vi "单体采集信息-new.vi"(0 "can卡类型":u8, 1 "设备索引号":u8, 2 "CAN端口":u8, 3 "VIC_Receive":refnum<vi>, 4 "数据":refnum<vi>, 5 "数据位置":refnum<vi>) -> ()   [LabVIEW 2013]
panel:
  out "Life:":dbl=25.0
  in  "213":bool
  in  "一次置位":bool
  in  "刷新":bool
  out "VCI_Receive 2":T1
  in  "板号":u8
  out "电池信息":T2
  in  "电池信息读取":bool
  out "时间":string
  in  "充电均衡":u32(colorbox)=6618880
  in  "放电均衡":u32(colorbox)=16711680
  out "均衡信息":string[][](table)=[["第1串", "1", "单体检测其它故障", "第25串", "1", "单体检测其它故障", "第49串", "1", "单体检测其它故障", "第73串", "1", "单体检测其它故障", "第97串", "1", "单体检测其它故障", "第121串", "1", "单体检测其它故障", "第145串", "1", "单体检测其它故障", "第169串", "1", "单体检测其它故障", "第193串", "1", "单体检测其它故障", "第217串", "1", "单体检测其它故障", "第241串", "1", "单体检测其它故障", "第265串", "1", "单体检测其它故障", "第289串", "1", "单体检测其它故障", ""], ["第2串", "", "", "第26串", "", "", "第50串", "", "", "第74串", "", "", "第98串", "", "", "第122串", "", "", "第146串", "", "", "第170串", "", "", "第194串", "", "", "第218串", "", "", "第242串", "", "", "第266串", "", "", "第290串", "", "", ""], ["第3串", "", "", "第27串", "", "", "第51串", "", "", "第75串", "", "", "第99串", "", "", "第123串", "", "", "第147串", "", "", "第171串", "", "", "第195串", "", "", "第219串", "", "", "第243串", "", "", "第267串", "", "", "第291串", "", "", ""], ["第4串", "", "", "第28串", "", "", "第52串", "", "", "第76串", "", "", "第100串", "", "", "第124串", "", "", "第148串", "", "", "第172串", "", "", "第196串", "", "", "第220串", "", "", "第244串", "", "", "第268串", "", "", "第292串", "", "", ""], ["第5串", "", "", "第29串", "", "", "第53串", "", "", "第77串", "", "", "第101串", "", "", "第125串", "", "", "第149串", "", "", "第173串", "", "", "第197串", "", "", "第221串", "", "", "第245串", "", "", "第269串", "", "", "第293串", "", "", ""], ["第6串", "", "", "第30串", "", "", "第54串", "", "", "第78串", "", "", "第102串", "", "", "第126串", "", "", "第150串", "", "", "第174串", "", "", "第198串", "", "", "第222串", "", "", "第246串", "", "", "第270串", "", "", "第294串", "", "", ""], ["第7串", "", "", "第31串", "", "", "第55串", "", "", "第79串", "", "", "第103串", "", "", "第127串", "", "", "第151串", "", "", "第175串", "", "", "第199串", "", "", "第223串", "", "", "第247串", "", "", "第271串", "", "", "第295串", "", "", ""], ["第8串", "", "", "第32串", "", "", "第56串", "", "", "第80串", "", "", "第104串", "", "", "第128串", "", "", "第152串", "", "", "第176串", "", "", "第200串", "", "", "第224串", "", "", "第248串", "", "", "第272串", "", "", "第296串", "", "", ""], ["第9串", "", "", "第33串", "", "", "第57串", "", "", "第81串", "", "", "第105串", "", "", "第129串", "", "", "第153串", "", "", "第177串", "", "", "第201串", "", "", "第225串", "", "", "第249串", "", "", "第273串", "", "", "第297串", "", "", ""], ["第10串", "", "", "第34串", "", "", "第58串", "", "", "第82串", "", "", "第106串", "", "", "第130串", "", "", "第154串", "", "", "第178串", "", "", "第202串", "", "", "第226串", "", "", "第250串", "", "", "第274串", "", "", "第298串", "", "", ""], ["第11串", "", "", "第35串", "", "", "第59串", "", "", "第83串", "", "", "第107串", "", "", "第131串", "", "", "第155串", "", "", "第179串", "", "", "第203串", "", "", "第227串", "", "", "第251串", "", "", "第275串", "", "", "第299串", "", "", ""], ["第12串", "", "", "第36串", "", "", "第60串", "", "", "第84串", "", "", "第108串", "", "", "第132串", "", "", "第156串", "", "", "第180串", "", "", "第204串", "", "", "第228串", "", "", "第252串", "", "", "第276串", "", "", "第300串", "", "", ""], ["第13串", "", "", "第37串", "", "", "第61串", "", "", "第85串", "", "", "第109串", "", "", "第133串", "", "", "第157串", "", "", "第181串", "", "", "第205串", "", "", "第229串", "", "", "第253串", "", "", "第277串", "", "", "", "", "", ""], ["第14串", "", "", "第38串", "", "", "第62串", "", "", "第86串", "", "", "第110串", "", "", "第134串", "", "", "第158串", "", "", "第182串", "", "", "第206串", "", "", "第230串", "", "", "第254串", "", "", "第278串", "", "", "", "", "", ""], ["第15串", "", "", "第39串", "", "", "第63串", "", "", "第87串", "", "", "第111串", "", "", "第135串", "", "", "第159串", "", "", "第183串", "", "", "第207串", "", "", "第231串", "", "", "第255串", "", "", "第279串", "", "", "", "", "", ""], ["第16串", "", "", "第40串", "", "", "第64串", "", "", "第88串", "", "", "第112串", "", "", "第136串", "", "", "第160串", "", "", "第184串", "", "", "第208串", "", "", "第232串", "", "", "第256串", "", "", "第280串", "", "", "", "", "", ""], ["第17串", "", "", "第41串", "", "", "第65串", "", "", "第89串", "", "", "第113串", "", "", "第137串", "", "", "第161串", "", "", "第185串", "", "", "第209串", "", "", "第233串", "", "", "第257串", "", "", "第281串", "", "", "", "", "", ""], ["第18串", "", "", "第42串", "", "", "第66串", "", "", "第90串", "", "", "第114串", "", "", "第138串", "", "", "第162串", "", "", "第186串", "", "", "第210串", "", "", "第234串", "", "", "第258串", "", "", "第282串", "", "", "", "", "", ""], ["第19串", "", "", "第43串", "", "", "第67串", "", "", "第91串", "", "", "第115串", "", "", "第139串", "", "", "第163串", "", "", "第187串", "", "", "第211串", "", "", "第235串", "", "", "第259串", "", "", "第283串", "", "", "", "", "", ""], ["第20串", "", "", "第44串", "", "", "第68串", "", "", "第92串", "", "", "第116串", "", "", "第140串", "", "", "第164串", "", "", "第188串", "", "", "第212串", "", "", "第236串", "", "", "第260串", "", "", "第284串", "", "", "", "", "", ""], ["第21串", "", "", "第45串", "", "", "第69串", "", "", "第93串", "", "", "第117串", "", "", "第141串", "", "", "第165串", "", "", "第189串", "", "", "第213串", "", "", "第237串", "", "", "第261串", "", "", "第285串", "", "", "", "", "", ""], ["第22串", "", "", "第46串", "", "", "第70串", "", "", "第94串", "", "", "第118串", "", "", "第142串", "", "", "第166串", "", "", "第190串", "", "", "第214串", "", "", "第238串", "", "", "第262串", "", "", "第286串", "", "", "", "", "", ""], ["第23串", "", "", "第47串", "", "", "第71串", "", "", "第95串", "", "", "第119串", "", "", "第143串", "", "", "第167串", "", "", "第191串", "", "", "第215串", "", "", "第239串", "", "", "第263串", "", "", "第287串", "", "", "", "", "", ""], ["第24串", "", "", "第48串", "", "", "第72串", "", "", "第96串", "", "", "第120串", "", "", "第144串", "", "", "第168串", "", "", "第192串", "", "", "第216串", "", "", "第240串", "", "", "第264串", "", "", "第288串", "", "", "", "", "", ""]]
  out "SOC":string[][](table)=[["第1串", "", "", "第25串", "", "", "第49串", "", "", "第73串", "", "", "第97串", "", "", "第121串", "", "", "第145串", "", "", "第169串", "", "", "第193串", "", "", "第217串", "", "", "第241串", "", "", "第265串", "", "", "第289串", "", "", ""], ["第2串", "", "", "第26串", "", "", "第50串", "", "", "第74串", "", "", "第98串", "", "", "第122串", "", "", "第146串", "", "", "第170串", "", "", "第194串", "", "", "第218串", "", "", "第242串", "", "", "第266串", "", "", "第290串", "", "", ""], ["第3串", "", "", "第27串", "", "", "第51串", "", "", "第75串", "", "", "第99串", "", "", "第123串", "", "", "第147串", "", "", "第171串", "", "", "第195串", "", "", "第219串", "", "", "第243串", "", "", "第267串", "", "", "第291串", "", "", ""], ["第4串", "", "", "第28串", "", "", "第52串", "", "", "第76串", "", "", "第100串", "", "", "第124串", "", "", "第148串", "", "", "第172串", "", "", "第196串", "", "", "第220串", "", "", "第244串", "", "", "第268串", "", "", "第292串", "", "", ""], ["第5串", "", "", "第29串", "", "", "第53串", "", "", "第77串", "", "", "第101串", "", "", "第125串", "", "", "第149串", "", "", "第173串", "", "", "第197串", "", "", "第221串", "", "", "第245串", "", "", "第269串", "", "", "第293串", "", "", ""], ["第6串", "", "", "第30串", "", "", "第54串", "", "", "第78串", "", "", "第102串", "", "", "第126串", "", "", "第150串", "", "", "第174串", "", "", "第198串", "", "", "第222串", "", "", "第246串", "", "", "第270串", "", "", "第294串", "", "", ""], ["第7串", "", "", "第31串", "", "", "第55串", "", "", "第79串", "", "", "第103串", "", "", "第127串", "", "", "第151串", "", "", "第175串", "", "", "第199串", "", "", "第223串", "", "", "第247串", "", "", "第271串", "", "", "第295串", "", "", ""], ["第8串", "", "", "第32串", "", "", "第56串", "", "", "第80串", "", "", "第104串", "", "", "第128串", "", "", "第152串", "", "", "第176串", "", "", "第200串", "", "", "第224串", "", "", "第248串", "", "", "第272串", "", "", "第296串", "", "", ""], ["第9串", "", "", "第33串", "", "", "第57串", "", "", "第81串", "", "", "第105串", "", "", "第129串", "", "", "第153串", "", "", "第177串", "", "", "第201串", "", "", "第225串", "", "", "第249串", "", "", "第273串", "", "", "第297串", "", "", ""], ["第10串", "", "", "第34串", "", "", "第58串", "", "", "第82串", "", "", "第106串", "", "", "第130串", "", "", "第154串", "", "", "第178串", "", "", "第202串", "", "", "第226串", "", "", "第250串", "", "", "第274串", "", "", "第298串", "", "", ""], ["第11串", "", "", "第35串", "", "", "第59串", "", "", "第83串", "", "", "第107串", "", "", "第131串", "", "", "第155串", "", "", "第179串", "", "", "第203串", "", "", "第227串", "", "", "第251串", "", "", "第275串", "", "", "第299串", "", "", ""], ["第12串", "", "", "第36串", "", "", "第60串", "", "", "第84串", "", "", "第108串", "", "", "第132串", "", "", "第156串", "", "", "第180串", "", "", "第204串", "", "", "第228串", "", "", "第252串", "", "", "第276串", "", "", "第300串", "", "", ""], ["第13串", "", "", "第37串", "", "", "第61串", "", "", "第85串", "", "", "第109串", "", "", "第133串", "", "", "第157串", "", "", "第181串", "", "", "第205串", "", "", "第229串", "", "", "第253串", "", "", "第277串", "", "", "", "", "", ""], ["第14串", "", "", "第38串", "", "", "第62串", "", "", "第86串", "", "", "第110串", "", "", "第134串", "", "", "第158串", "", "", "第182串", "", "", "第206串", "", "", "第230串", "", "", "第254串", "", "", "第278串", "", "", "", "", "", ""], ["第15串", "", "", "第39串", "", "", "第63串", "", "", "第87串", "", "", "第111串", "", "", "第135串", "", "", "第159串", "", "", "第183串", "", "", "第207串", "", "", "第231串", "", "", "第255串", "", "", "第279串", "", "", "", "", "", ""], ["第16串", "", "", "第40串", "", "", "第64串", "", "", "第88串", "", "", "第112串", "", "", "第136串", "", "", "第160串", "", "", "第184串", "", "", "第208串", "", "", "第232串", "", "", "第256串", "", "", "第280串", "", "", "", "", "", ""], ["第17串", "", "", "第41串", "", "", "第65串", "", "", "第89串", "", "", "第113串", "", "", "第137串", "", "", "第161串", "", "", "第185串", "", "", "第209串", "", "", "第233串", "", "", "第257串", "", "", "第281串", "", "", "", "", "", ""], ["第18串", "", "", "第42串", "", "", "第66串", "", "", "第90串", "", "", "第114串", "", "", "第138串", "", "", "第162串", "", "", "第186串", "", "", "第210串", "", "", "第234串", "", "", "第258串", "", "", "第282串", "", "", "", "", "", ""], ["第19串", "", "", "第43串", "", "", "第67串", "", "", "第91串", "", "", "第115串", "", "", "第139串", "", "", "第163串", "", "", "第187串", "", "", "第211串", "", "", "第235串", "", "", "第259串", "", "", "第283串", "", "", "", "", "", ""], ["第20串", "", "", "第44串", "", "", "第68串", "", "", "第92串", "", "", "第116串", "", "", "第140串", "", "", "第164串", "", "", "第188串", "", "", "第212串", "", "", "第236串", "", "", "第260串", "", "", "第284串", "", "", "", "", "", ""], ["第21串", "", "", "第45串", "", "", "第69串", "", "", "第93串", "", "", "第117串", "", "", "第141串", "", "", "第165串", "", "", "第189串", "", "", "第213串", "", "", "第237串", "", "", "第261串", "", "", "第285串", "", "", "", "", "", ""], ["第22串", "", "", "第46串", "", "", "第70串", "", "", "第94串", "", "", "第118串", "", "", "第142串", "", "", "第166串", "", "", "第190串", "", "", "第214串", "", "", "第238串", "", "", "第262串", "", "", "第286串", "", "", "", "", "", ""], ["第23串", "", "", "第47串", "", "", "第71串", "", "", "第95串", "", "", "第119串", "", "", "第143串", "", "", "第167串", "", "", "第191串", "", "", "第215串", "", "", "第239串", "", "", "第263串", "", "", "第287串", "", "", "", "", "", ""], ["第24串", "", "", "第48串", "", "", "第72串", "", "", "第96串", "", "", "第120串", "", "", "第144串", "", "", "第168串", "", "", "第192串", "", "", "第216串", "", "", "第240串", "", "", "第264串", "", "", "第288串", "", "", "", "", "", ""]]
  out "内阻":string[][](table)=[["第1串", "", "", "第25串", "", "", "第49串", "", "", "第73串", "", "", "第97串", "", "", "第121串", "", "", "第145串", "", "", "第169串", "", "", "第193串", "", "", "第217串", "", "", "第241串", "", "", "第265串", "", "", "第289串", "", "", ""], ["第2串", "", "", "第26串", "", "", "第50串", "", "", "第74串", "", "", "第98串", "", "", "第122串", "", "", "第146串", "", "", "第170串", "", "", "第194串", "", "", "第218串", "", "", "第242串", "", "", "第266串", "", "", "第290串", "", "", ""], ["第3串", "", "", "第27串", "", "", "第51串", "", "", "第75串", "", "", "第99串", "", "", "第123串", "", "", "第147串", "", "", "第171串", "", "", "第195串", "", "", "第219串", "", "", "第243串", "", "", "第267串", "", "", "第291串", "", "", ""], ["第4串", "", "", "第28串", "", "", "第52串", "", "", "第76串", "", "", "第100串", "", "", "第124串", "", "", "第148串", "", "", "第172串", "", "", "第196串", "", "", "第220串", "", "", "第244串", "", "", "第268串", "", "", "第292串", "", "", ""], ["第5串", "", "", "第29串", "", "", "第53串", "", "", "第77串", "", "", "第101串", "", "", "第125串", "", "", "第149串", "", "", "第173串", "", "", "第197串", "", "", "第221串", "", "", "第245串", "", "", "第269串", "", "", "第293串", "", "", ""], ["第6串", "", "", "第30串", "", "", "第54串", "", "", "第78串", "", "", "第102串", "", "", "第126串", "", "", "第150串", "", "", "第174串", "", "", "第198串", "", "", "第222串", "", "", "第246串", "", "", "第270串", "", "", "第294串", "", "", ""], ["第7串", "", "", "第31串", "", "", "第55串", "", "", "第79串", "", "", "第103串", "", "", "第127串", "", "", "第151串", "", "", "第175串", "", "", "第199串", "", "", "第223串", "", "", "第247串", "", "", "第271串", "", "", "第295串", "", "", ""], ["第8串", "", "", "第32串", "", "", "第56串", "", "", "第80串", "", "", "第104串", "", "", "第128串", "", "", "第152串", "", "", "第176串", "", "", "第200串", "", "", "第224串", "", "", "第248串", "", "", "第272串", "", "", "第296串", "", "", ""], ["第9串", "", "", "第33串", "", "", "第57串", "", "", "第81串", "", "", "第105串", "", "", "第129串", "", "", "第153串", "", "", "第177串", "", "", "第201串", "", "", "第225串", "", "", "第249串", "", "", "第273串", "", "", "第297串", "", "", ""], ["第10串", "", "", "第34串", "", "", "第58串", "", "", "第82串", "", "", "第106串", "", "", "第130串", "", "", "第154串", "", "", "第178串", "", "", "第202串", "", "", "第226串", "", "", "第250串", "", "", "第274串", "", "", "第298串", "", "", ""], ["第11串", "", "", "第35串", "", "", "第59串", "", "", "第83串", "", "", "第107串", "", "", "第131串", "", "", "第155串", "", "", "第179串", "", "", "第203串", "", "", "第227串", "", "", "第251串", "", "", "第275串", "", "", "第299串", "", "", ""], ["第12串", "", "", "第36串", "", "", "第60串", "", "", "第84串", "", "", "第108串", "", "", "第132串", "", "", "第156串", "", "", "第180串", "", "", "第204串", "", "", "第228串", "", "", "第252串", "", "", "第276串", "", "", "第300串", "", "", ""], ["第13串", "", "", "第37串", "", "", "第61串", "", "", "第85串", "", "", "第109串", "", "", "第133串", "", "", "第157串", "", "", "第181串", "", "", "第205串", "", "", "第229串", "", "", "第253串", "", "", "第277串", "", "", "", "", "", ""], ["第14串", "", "", "第38串", "", "", "第62串", "", "", "第86串", "", "", "第110串", "", "", "第134串", "", "", "第158串", "", "", "第182串", "", "", "第206串", "", "", "第230串", "", "", "第254串", "", "", "第278串", "", "", "", "", "", ""], ["第15串", "", "", "第39串", "", "", "第63串", "", "", "第87串", "", "", "第111串", "", "", "第135串", "", "", "第159串", "", "", "第183串", "", "", "第207串", "", "", "第231串", "", "", "第255串", "", "", "第279串", "", "", "", "", "", ""], ["第16串", "", "", "第40串", "", "", "第64串", "", "", "第88串", "", "", "第112串", "", "", "第136串", "", "", "第160串", "", "", "第184串", "", "", "第208串", "", "", "第232串", "", "", "第256串", "", "", "第280串", "", "", "", "", "", ""], ["第17串", "", "", "第41串", "", "", "第65串", "", "", "第89串", "", "", "第113串", "", "", "第137串", "", "", "第161串", "", "", "第185串", "", "", "第209串", "", "", "第233串", "", "", "第257串", "", "", "第281串", "", "", "", "", "", ""], ["第18串", "", "", "第42串", "", "", "第66串", "", "", "第90串", "", "", "第114串", "", "", "第138串", "", "", "第162串", "", "", "第186串", "", "", "第210串", "", "", "第234串", "", "", "第258串", "", "", "第282串", "", "", "", "", "", ""], ["第19串", "", "", "第43串", "", "", "第67串", "", "", "第91串", "", "", "第115串", "", "", "第139串", "", "", "第163串", "", "", "第187串", "", "", "第211串", "", "", "第235串", "", "", "第259串", "", "", "第283串", "", "", "", "", "", ""], ["第20串", "", "", "第44串", "", "", "第68串", "", "", "第92串", "", "", "第116串", "", "", "第140串", "", "", "第164串", "", "", "第188串", "", "", "第212串", "", "", "第236串", "", "", "第260串", "", "", "第284串", "", "", "", "", "", ""], ["第21串", "", "", "第45串", "", "", "第69串", "", "", "第93串", "", "", "第117串", "", "", "第141串", "", "", "第165串", "", "", "第189串", "", "", "第213串", "", "", "第237串", "", "", "第261串", "", "", "第285串", "", "", "", "", "", ""], ["第22串", "", "", "第46串", "", "", "第70串", "", "", "第94串", "", "", "第118串", "", "", "第142串", "", "", "第166串", "", "", "第190串", "", "", "第214串", "", "", "第238串", "", "", "第262串", "", "", "第286串", "", "", "", "", "", ""], ["第23串", "", "", "第47串", "", "", "第71串", "", "", "第95串", "", "", "第119串", "", "", "第143串", "", "", "第167串", "", "", "第191串", "", "", "第215串", "", "", "第239串", "", "", "第263串", "", "", "第287串", "", "", "", "", "", ""], ["第24串", "", "", "第48串", "", "", "第72串", "", "", "第96串", "", "", "第120串", "", "", "第144串", "", "", "第168串", "", "", "第192串", "", "", "第216串", "", "", "第240串", "", "", "第264串", "", "", "第288串", "", "", "", "", "", ""]]
  out "温度表格":string[][](table)=[["第1串", "", "", "第25串", "", "", "第49串", "", "", "第73串", "", "", "第97串", "", "", "第121串", "", "", "第145串", "", "", "第169串", "", "", "第193串", "", "", "第217串", "", "", "第241串", "", "", "第265串", "", "", "第289串", "", "", ""], ["第2串", "", "", "第26串", "", "", "第50串", "", "", "第74串", "", "", "第98串", "", "", "第122串", "", "", "第146串", "", "", "第170串", "", "", "第194串", "", "", "第218串", "", "", "第242串", "", "", "第266串", "", "", "第290串", "", "", ""], ["第3串", "", "", "第27串", "", "", "第51串", "", "", "第75串", "", "", "第99串", "", "", "第123串", "", "", "第147串", "", "", "第171串", "", "", "第195串", "", "", "第219串", "", "", "第243串", "", "", "第267串", "", "", "第291串", "", "", ""], ["第4串", "", "", "第28串", "", "", "第52串", "", "", "第76串", "", "", "第100串", "", "", "第124串", "", "", "第148串", "", "", "第172串", "", "", "第196串", "", "", "第220串", "", "", "第244串", "", "", "第268串", "", "", "第292串", "", "", ""], ["第5串", "", "", "第29串", "", "", "第53串", "", "", "第77串", "", "", "第101串", "", "", "第125串", "", "", "第149串", "", "", "第173串", "", "", "第197串", "", "", "第221串", "", "", "第245串", "", "", "第269串", "", "", "第293串", "", "", ""], ["第6串", "", "", "第30串", "", "", "第54串", "", "", "第78串", "", "", "第102串", "", "", "第126串", "", "", "第150串", "", "", "第174串", "", "", "第198串", "", "", "第222串", "", "", "第246串", "", "", "第270串", "", "", "第294串", "", "", ""], ["第7串", "", "", "第31串", "", "", "第55串", "", "", "第79串", "", "", "第103串", "", "", "第127串", "", "", "第151串", "", "", "第175串", "", "", "第199串", "", "", "第223串", "", "", "第247串", "", "", "第271串", "", "", "第295串", "", "", ""], ["第8串", "", "", "第32串", "", "", "第56串", "", "", "第80串", "", "", "第104串", "", "", "第128串", "", "", "第152串", "", "", "第176串", "", "", "第200串", "", "", "第224串", "", "", "第248串", "", "", "第272串", "", "", "第296串", "", "", ""], ["第9串", "", "", "第33串", "", "", "第57串", "", "", "第81串", "", "", "第105串", "", "", "第129串", "", "", "第153串", "", "", "第177串", "", "", "第201串", "", "", "第225串", "", "", "第249串", "", "", "第273串", "", "", "第297串", "", "", ""], ["第10串", "", "", "第34串", "", "", "第58串", "", "", "第82串", "", "", "第106串", "", "", "第130串", "", "", "第154串", "", "", "第178串", "", "", "第202串", "", "", "第226串", "", "", "第250串", "", "", "第274串", "", "", "第298串", "", "", ""], ["第11串", "", "", "第35串", "", "", "第59串", "", "", "第83串", "", "", "第107串", "", "", "第131串", "", "", "第155串", "", "", "第179串", "", "", "第203串", "", "", "第227串", "", "", "第251串", "", "", "第275串", "", "", "第299串", "", "", ""], ["第12串", "", "", "第36串", "", "", "第60串", "", "", "第84串", "", "", "第108串", "", "", "第132串", "", "", "第156串", "", "", "第180串", "", "", "第204串", "", "", "第228串", "", "", "第252串", "", "", "第276串", "", "", "第300串", "", "", ""], ["第13串", "", "", "第37串", "", "", "第61串", "", "", "第85串", "", "", "第109串", "", "", "第133串", "", "", "第157串", "", "", "第181串", "", "", "第205串", "", "", "第229串", "", "", "第253串", "", "", "第277串", "", "", "", "", "", ""], ["第14串", "", "", "第38串", "", "", "第62串", "", "", "第86串", "", "", "第110串", "", "", "第134串", "", "", "第158串", "", "", "第182串", "", "", "第206串", "", "", "第230串", "", "", "第254串", "", "", "第278串", "", "", "", "", "", ""], ["第15串", "", "", "第39串", "", "", "第63串", "", "", "第87串", "", "", "第111串", "", "", "第135串", "", "", "第159串", "", "", "第183串", "", "", "第207串", "", "", "第231串", "", "", "第255串", "", "", "第279串", "", "", "", "", "", ""], ["第16串", "", "", "第40串", "", "", "第64串", "", "", "第88串", "", "", "第112串", "", "", "第136串", "", "", "第160串", "", "", "第184串", "", "", "第208串", "", "", "第232串", "", "", "第256串", "", "", "第280串", "", "", "", "", "", ""], ["第17串", "", "", "第41串", "", "", "第65串", "", "", "第89串", "", "", "第113串", "", "", "第137串", "", "", "第161串", "", "", "第185串", "", "", "第209串", "", "", "第233串", "", "", "第257串", "", "", "第281串", "", "", "", "", "", ""], ["第18串", "", "", "第42串", "", "", "第66串", "", "", "第90串", "", "", "第114串", "", "", "第138串", "", "", "第162串", "", "", "第186串", "", "", "第210串", "", "", "第234串", "", "", "第258串", "", "", "第282串", "", "", "", "", "", ""], ["第19串", "", "", "第43串", "", "", "第67串", "", "", "第91串", "", "", "第115串", "", "", "第139串", "", "", "第163串", "", "", "第187串", "", "", "第211串", "", "", "第235串", "", "", "第259串", "", "", "第283串", "", "", "", "", "", ""], ["第20串", "", "", "第44串", "", "", "第68串", "", "", "第92串", "", "", "第116串", "", "", "第140串", "", "", "第164串", "", "", "第188串", "", "", "第212串", "", "", "第236串", "", "", "第260串", "", "", "第284串", "", "", "", "", "", ""], ["第21串", "", "", "第45串", "", "", "第69串", "", "", "第93串", "", "", "第117串", "", "", "第141串", "", "", "第165串", "", "", "第189串", "", "", "第213串", "", "", "第237串", "", "", "第261串", "", "", "第285串", "", "", "", "", "", ""], ["第22串", "", "", "第46串", "", "", "第70串", "", "", "第94串", "", "", "第118串", "", "", "第142串", "", "", "第166串", "", "", "第190串", "", "", "第214串", "", "", "第238串", "", "", "第262串", "", "", "第286串", "", "", "", "", "", ""], ["第23串", "", "", "第47串", "", "", "第71串", "", "", "第95串", "", "", "第119串", "", "", "第143串", "", "", "第167串", "", "", "第191串", "", "", "第215串", "", "", "第239串", "", "", "第263串", "", "", "第287串", "", "", "", "", "", ""], ["第24串", "", "", "第48串", "", "", "第72串", "", "", "第96串", "", "", "第120串", "", "", "第144串", "", "", "第168串", "", "", "第192串", "", "", "第216串", "", "", "第240串", "", "", "第264串", "", "", "第288串", "", "", "", "", "", ""]]
  in  "主界面选项":T3(radio)
  in  "电池信息选项":enum16{"电池信息", "历史信息"}(ring)
  out "位置":dbl[](array[numeric])
  out "输出数据":dbl[](array[numeric])
  in  "命令":u32=133
  in  "VCI_Receive":T1 {"Rsv3" max=0 format="%x"; "Rsv2" min=101 format="%x"; "Rsv1" format="%x"; "Data8" format="%x"; "Data7" format="%x"; "Data6" format="%x"; "Data5" format="%x"; "Data4" format="%x"; "Data3" format="%x"; "Data2" format="%x"; "Data1" format="%x"; "DataLen" format="%x"; "ExternFlag" format="%x"; "RemoteFlag" format="%x"; "SendType" format="%x"; "TimeFlag" format="%x"; "TimeStamp" format="%x"; "ID" format="%x"}
  out "状态":bool
  in  "停止":bool
  in  "选项卡控件":enum32{"单体电压", "单体温度", "单体内阻", "单体SOC"}(tab)
  in  "偏差":dbl=0.008 format="%.3f"
  in  "基准":dbl=3.3 format="%.3f"
  out "等待均衡":u32(colorbox)=16776770
  in  "故障信息选择按键 2":enum32{"单选选项2", "单选选项2 2", "单选选项2 3", "单选选项1"}(radio)=enum."单选选项1"
  out "电压选择":enum32{"1-96", "97-192", "193-288", "289-300"}(tab)
  out "1":T4={"1 102"={"第1串"=0.0, "第2串"=0.0, "第3串"=0.0, "第4串"=0.0, "第5串"=0.0, "第6串"=0.0, "第7串"=0.0, "第8串"=0.0, "第9串"=0.0, "第10串"=0.0, "第11串"=0.0, "第12串"=0.0, "第一串 2"=0.0, "第一串 4"=0.0, "第一串 6"=0.0, "第一串 8"=0.0, "第一串 10"=0.0, "第一串 12"=0.0, "第一串 14"=0.0, "第一串 16"=0.0, "第一串 18"=0.0, "第一串 20"=0.0, "第一串 22"=0.0, "第一串 24"=0.0}, "1 3"={"第13串"=0.0, "第14串"=0.0, "第15串"=0.0, "第16串"=0.0, "第17串"=0.0, "第18串"=0.0, "第19串"=0.0, "第20串"=0.0, "第21串"=0.0, "第22串"=0.0, "第23串"=0.0, "第24串"=0.0, "第一串 2"=0.0, "第一串 4"=0.0, "第一串 6"=0.0, "第一串 8"=0.0, "第一串 10"=0.0, "第一串 12"=0.0, "第一串 14"=0.0, "第一串 16"=0.0, "第一串 18"=0.0, "第一串 20"=0.0, "第一串 22"=0.0, "第一串 24"=0.0}, "1 4"={"第25串"=0.0, "第26串"=0.0, "第27串"=0.0, "第28串"=0.0, "第29串"=0.0, "第30串"=0.0, "第31串"=0.0, "第32串"=0.0, "第33串"=0.0, "第34串"=0.0, "第35串"=0.0, "第36串"=0.0, "第一串 2"=0.0, "第一串 4"=0.0, "第一串 6"=0.0, "第一串 8"=0.0, "第一串 10"=0.0, "第一串 12"=0.0, "第一串 14"=0.0, "第一串 16"=0.0, "第一串 18"=0.0, "第一串 20"=0.0, "第一串 22"=0.0, "第一串 24"=0.0}, "1 6"={"第37串"=0.0, "第38串"=0.0, "第39串"=0.0, "第40串"=0.0, "第41串"=0.0, "第42串"=0.0, "第43串"=0.0, "第44串"=0.0, "第45串"=0.0, "第46串"=0.0, "第47串"=0.0, "第48串"=0.0, "第一串 2"=0.0, "第一串 4"=0.0, "第一串 6"=0.0, "第一串 8"=0.0, "第一串 10"=0.0, "第一串 12"=0.0, "第一串 14"=0.0, "第一串 16"=0.0, "第一串 18"=0.0, "第一串 20"=0.0, "第一串 22"=0.0, "第一串 24"=0.0}, "1 7"={"第49串"=0.0, "第50串"=0.0, "第51串"=0.0, "第52串"=0.0, "第53串"=0.0, "第54串"=0.0, "第55串"=0.0, "第56串"=0.0, "第57串"=0.0, "第58串"=0.0, "第59串"=0.0, "第60串"=0.0, "第一串 2"=0.0, "第一串 4"=0.0, "第一串 6"=0.0, "第一串 8"=0.0, "第一串 10"=0.0, "第一串 12"=0.0, "第一串 14"=0.0, "第一串 16"=0.0, "第一串 18"=0.0, "第一串 20"=0.0, "第一串 22"=0.0, "第一串 24"=0.0}, "1 8"={"第61串"=0.0, "第62串"=0.0, "第63串"=0.0, "第64串"=0.0, "第65串"=0.0, "第66串"=0.0, "第67串"=0.0, "第68串"=0.0, "第69串"=0.0, "第70串"=0.0, "第71串"=0.0, "第72串"=0.0, "第一串 2"=0.0, "第一串 4"=0.0, "第一串 6"=0.0, "第一串 8"=0.0, "第一串 10"=0.0, "第一串 12"=0.0, "第一串 14"=0.0, "第一串 16"=0.0, "第一串 18"=0.0, "第一串 20"=0.0, "第一串 22"=0.0, "第一串 24"=0.0}, "1 9"={"第73串"=0.0, "第74串"=0.0, "第75串"=0.0, "第76串"=0.0, "第77串"=0.0, "第78串"=0.0, "第79串"=0.0, "第80串"=0.0, "第81串"=0.0, "第82串"=0.0, "第83串"=0.0, "第84串"=0.0, "第一串 2"=0.0, "第一串 4"=0.0, "第一串 6"=0.0, "第一串 8"=0.0, "第一串 10"=0.0, "第一串 12"=0.0, "第一串 14"=0.0, "第一串 16"=0.0, "第一串 18"=0.0, "第一串 20"=0.0, "第一串 22"=0.0, "第一串 24"=0.0}, "1 10"={"第85串"=0.0, "第86串"=0.0, "第87串"=0.0, "第88串"=0.0, "第89串"=0.0, "第90串"=0.0, "第91串"=0.0, "第92串"=0.0, "第93串"=0.0, "第94串"=0.0, "第95串"=0.0, "第96串"=0.0, "第一串 2"=0.0, "第一串 4"=0.0, "第一串 6"=0.0, "第一串 8"=0.0, "第一串 10"=0.0, "第一串 12"=0.0, "第一串 14"=0.0, "第一串 16"=0.0, "第一串 18"=0.0, "第一串 20"=0.0, "第一串 22"=0.0, "第一串 24"=0.0}, "1 12"={"充电1"=13816530, "充电1"=13816530, "充电1"=13816530, "充电1"=13816530, "充电1"=13816530, "充电1"=13816530, "充电1"=13816530, "充电1"=13816530, "充电1"=13816530, "充电1"=13816530, "充电1"=13816530, "充电1"=13816530}, "1 28"={"充电1"=13816530, "充电1"=13816530, "充电1"=13816530, "充电1"=13816530, "充电1"=13816530, "充电1"=13816530, "充电1"=13816530, "充电1"=13816530, "充电1"=13816530, "充电1"=13816530, "充电1"=13816530, "充电1"=13816530}, "1 25"={"充电1"=0, "充电1"=0, "充电1"=0, "充电1"=0, "充电1"=0, "充电1"=0, "充电1"=0, "充电1"=0, "充电1"=0, "充电1"=0, "充电1"=0, "充电1"=0}, "1 31"={"充电1"=0, "充电1"=0, "充电1"=0, "充电1"=0, "充电1"=0, "充电1"=0, "充电1"=0, "充电1"=0, "充电1"=0, "充电1"=0, "充电1"=0, "充电1"=0}, "1 16"={"充电1"=0, "充电1"=0, "充电1"=0, "充电1"=0, "充电1"=0, "充电1"=0, "充电1"=0, "充电1"=0, "充电1"=0, "充电1"=0, "充电1"=0, "充电1"=0}, "1 19"={"充电1"=0, "充电1"=0, "充电1"=0, "充电1"=0, "充电1"=0, "充电1"=0, "充电1"=0, "充电1"=0, "充电1"=0, "充电1"=0, "充电1"=0, "充电1"=0}, "1 22"={"充电1"=0, "充电1"=0, "充电1"=0, "充电1"=0, "充电1"=0, "充电1"=0, "充电1"=0, "充电1"=0, "充电1"=0, "充电1"=0, "充电1"=0, "充电1"=0}, "1 34"={"充电1"=0, "充电1"=0, "充电1"=0, "充电1"=0, "充电1"=0, "充电1"=0, "充电1"=0, "充电1"=0, "充电1"=0, "充电1"=0, "充电1"=0, "充电1"=0}, "1 11"={"充电1"=13816530, "充电1"=13816530, "充电1"=13816530, "充电1"=13816530, "充电1"=13816530, "充电1"=13816530, "充电1"=13816530, "充电1"=13816530, "充电1"=13816530, "充电1"=13816530, "充电1"=13816530, "充电1"=13816530}, "1 27"={"充电1"=0, "充电1"=0, "充电1"=0, "充电1"=0, "充电1"=0, "充电1"=0, "充电1"=0, "充电1"=0, "充电1"=0, "充电1"=0, "充电1"=0, "充电1"=0}, "1 24"={"充电1"=0, "充电1"=0, "充电1"=0, "充电1"=0, "充电1"=0, "充电1"=0, "充电1"=0, "充电1"=0, "充电1"=0, "充电1"=0, "充电1"=0, "充电1"=0}, "1 30"={"充电1"=0, "充电1"=0, "充电1"=0, "充电1"=0, "充电1"=0, "充电1"=0, "充电1"=0, "充电1"=0, "充电1"=0, "充电1"=0, "充电1"=0, "充电1"=0}, "1 15"={"充电1"=0, "充电1"=0, "充电1"=0, "充电1"=0, "充电1"=0, "充电1"=0, "充电1"=0, "充电1"=0, "充电1"=0, "充电1"=0, "充电1"=0, "充电1"=0}, "1 18"={"充电1"=0, "充电1"=0, "充电1"=0, "充电1"=0, "充电1"=0, "充电1"=0, "充电1"=0, "充电1"=0, "充电1"=0, "充电1"=0, "充电1"=0, "充电1"=0}, "1 21"={"充电1"=0, "充电1"=0, "充电1"=0, "充电1"=0, "充电1"=0, "充电1"=0, "充电1"=0, "充电1"=0, "充电1"=0, "充电1"=0, "充电1"=0, "充电1"=0}, "1 33"={"充电1"=0, "充电1"=0, "充电1"=0, "充电1"=0, "充电1"=0, "充电1"=0, "充电1"=0, "充电1"=0, "充电1"=0, "充电1"=0, "充电1"=0, "充电1"=0}, "1 13"={"均衡故障"=0, "均衡故障 2"=0.0, "均衡故障 3"=0.0, "均衡故障 4"=0.0, "均衡故障 5"=0.0, "均衡故障 6"=0.0, "均衡故障 7"=0.0, "均衡故障 8"=0.0, "均衡故障 9"=0.0, "均衡故障 10"=0.0, "均衡故障 11"=0.0, "均衡故障 12"=0.0}, "1 26"={"均衡故障"=0, "均衡故障 2"=0.0, "均衡故障 3"=0.0, "均衡故障 4"=0.0, "均衡故障 5"=0.0, "均衡故障 6"=0.0, "均衡故障 7"=0.0, "均衡故障 8"=0.0, "均衡故障 9"=0.0, "均衡故障 10"=0.0, "均衡故障 11"=0.0, "均衡故障 12"=0.0}, "1 23"={"均衡故障"=0, "均衡故障 2"=0.0, "均衡故障 3"=0.0, "均衡故障 4"=0.0, "均衡故障 5"=0.0, "均衡故障 6"=0.0, "均衡故障 7"=0.0, "均衡故障 8"=0.0, "均衡故障 9"=0.0, "均衡故障 10"=0.0, "均衡故障 11"=0.0, "均衡故障 12"=0.0}, "1 29"={"均衡故障"=0, "均衡故障 2"=0.0, "均衡故障 3"=0.0, "均衡故障 4"=0.0, "均衡故障 5"=0.0, "均衡故障 6"=0.0, "均衡故障 7"=0.0, "均衡故障 8"=0.0, "均衡故障 9"=0.0, "均衡故障 10"=0.0, "均衡故障 11"=0.0, "均衡故障 12"=0.0}, "1 14"={"均衡故障"=0, "均衡故障 2"=0.0, "均衡故障 3"=0.0, "均衡故障 4"=0.0, "均衡故障 5"=0.0, "均衡故障 6"=0.0, "均衡故障 7"=0.0, "均衡故障 8"=0.0, "均衡故障 9"=0.0, "均衡故障 10"=0.0, "均衡故障 11"=0.0, "均衡故障 12"=0.0}, "1 17"={"均衡故障"=0, "均衡故障 2"=0.0, "均衡故障 3"=0.0, "均衡故障 4"=0.0, "均衡故障 5"=0.0, "均衡故障 6"=0.0, "均衡故障 7"=0.0, "均衡故障 8"=0.0, "均衡故障 9"=0.0, "均衡故障 10"=0.0, "均衡故障 11"=0.0, "均衡故障 12"=0.0}, "1 20"={"均衡故障"=0, "均衡故障 2"=0.0, "均衡故障 3"=0.0, "均衡故障 4"=0.0, "均衡故障 5"=0.0, "均衡故障 6"=0.0, "均衡故障 7"=0.0, "均衡故障 8"=0.0, "均衡故障 9"=0.0, "均衡故障 10"=0.0, "均衡故障 11"=0.0, "均衡故障 12"=0.0}, "1 32"={"均衡故障"=0, "均衡故障 2"=0.0, "均衡故障 3"=0.0, "均衡故障 4"=0.0, "均衡故障 5"=0.0, "均衡故障 6"=0.0, "均衡故障 7"=0.0, "均衡故障 8"=0.0, "均衡故障 9"=0.0, "均衡故障 10"=0.0, "均衡故障 11"=0.0, "均衡故障 12"=0.0}} {"1 102"."第一串 24" format="%#.2f"; "1 102"."第12串" format="%.3f"; "1 102"."第一串 22" format="%#.2f"; "1 102"."第11串" format="%.3f"; "1 102"."第一串 20" format="%#.2f"; "1 102"."第10串" format="%.3f"; "1 102"."第一串 18" format="%#.2f"; "1 102"."第9串" format="%.3f"; "1 102"."第一串 16" format="%#.2f"; "1 102"."第8串" format="%.3f"; "1 102"."第一串 14" format="%#.2f"; "1 102"."第7串" format="%.3f"; "1 102"."第一串 12" format="%#.2f"; "1 102"."第6串" format="%.3f"; "1 102"."第一串 10" format="%#.2f"; "1 102"."第5串" format="%.3f"; "1 102"."第一串 8" format="%#.2f"; "1 102"."第4串" format="%.3f"; "1 102"."第一串 6" format="%#.2f"; "1 102"."第3串" format="%.3f"; "1 102"."第一串 4" format="%#.2f"; "1 102"."第2串" format="%.3f"; "1 102"."第一串 2" format="%#.2f"; "1 102"."第1串" format="%.3f"; "1 10"."第96串" format="%.3f"; "1 10"."第95串" format="%.3f"; "1 10"."第94串" format="%.3f"; "1 10"."第93串" format="%.3f"; "1 10"."第92串" format="%.3f"; "1 10"."第91串" format="%.3f"; "1 10"."第90串" format="%.3f"; "1 10"."第89串" format="%.3f"; "1 10"."第88串" format="%.3f"; "1 10"."第87串" format="%.3f"; "1 10"."第86串" format="%.3f"; "1 10"."第85串" format="%.3f"; "1 9"."第84串" format="%.3f"; "1 9"."第83串" format="%.3f"; "1 9"."第82串" format="%.3f"; "1 9"."第81串" format="%.3f"; "1 9"."第80串" format="%.3f"; "1 9"."第79串" format="%.3f"; "1 9"."第78串" format="%.3f"; "1 9"."第77串" format="%.3f"; "1 9"."第76串" format="%.3f"; "1 9"."第75串" format="%.3f"; "1 9"."第74串" format="%.3f"; "1 9"."第73串" format="%.3f"; "1 8"."第72串" format="%.3f"; "1 8"."第71串" format="%.3f"; "1 8"."第70串" format="%.3f"; "1 8"."第69串" format="%.3f"; "1 8"."第68串" format="%.3f"; "1 8"."第67串" format="%.3f"; "1 8"."第66串" format="%.3f"; "1 8"."第65串" format="%.3f"; "1 8"."第64串" format="%.3f"; "1 8"."第63串" format="%.3f"; "1 8"."第62串" format="%.3f"; "1 8"."第61串" format="%.3f"; "1 7"."第60串" format="%.3f"; "1 7"."第59串" format="%.3f"; "1 7"."第58串" format="%.3f"; "1 7"."第57串" format="%.3f"; "1 7"."第56串" format="%.3f"; "1 7"."第55串" format="%.3f"; "1 7"."第54串" format="%.3f"; "1 7"."第53串" format="%.3f"; "1 7"."第52串" format="%.3f"; "1 7"."第51串" format="%.3f"; "1 7"."第50串" format="%.3f"; "1 7"."第49串" format="%.3f"; "1 6"."第48串" format="%.3f"; "1 6"."第47串" format="%.3f"; "1 6"."第46串" format="%.3f"; "1 6"."第45串" format="%.3f"; "1 6"."第44串" format="%.3f"; "1 6"."第43串" format="%.3f"; "1 6"."第42串" format="%.3f"; "1 6"."第41串" format="%.3f"; "1 6"."第40串" format="%.3f"; "1 6"."第39串" format="%.3f"; "1 6"."第38串" format="%.3f"; "1 6"."第37串" format="%.3f"; "1 4"."第36串" format="%.3f"; "1 4"."第35串" format="%.3f"; "1 4"."第34串" format="%.3f"; "1 4"."第33串" format="%.3f"; "1 4"."第32串" format="%.3f"; "1 4"."第31串" format="%.3f"; "1 4"."第30串" format="%.3f"; "1 4"."第29串" format="%.3f"; "1 4"."第28串" format="%.3f"; "1 4"."第27串" format="%.3f"; "1 4"."第26串" format="%.3f"; "1 4"."第25串" format="%.3f"; "1 3"."第24串" format="%.3f"; "1 3"."第23串" format="%.3f"; "1 3"."第22串" format="%.3f"; "1 3"."第21串" format="%.3f"; "1 3"."第20串" format="%.3f"; "1 3"."第19串" format="%.3f"; "1 3"."第18串" format="%.3f"; "1 3"."第17串" format="%.3f"; "1 3"."第16串" format="%.3f"; "1 3"."第15串" format="%.3f"; "1 3"."第14串" format="%.3f"; "1 3"."第13串" format="%.3f"}
  out "2":T5={"1 26"={"第97串"=0.0, "第98串"=0.0, "第99串"=0.0, "第100串"=0.0, "第101串"=0.0, "第102串"=0.0, "第103串"=0.0, "第104串"=0.0, "第105串"=0.0, "第106串"=0.0, "第107串"=0.0, "第108串"=0.0, "第一串 2"=0.0, "第一串 4"=0.0, "第一串 6"=0.0, "第一串 8"=0.0, "第一串 10"=0.0, "第一串 12"=0.0, "第一串 14"=0.0, "第一串 16"=0.0, "第一串 18"=0.0, "第一串 20"=0.0, "第一串 22"=0.0, "第一串 24"=0.0}, "1 27"={"第109串"=0.0, "第110串"=0.0, "第111串"=0.0, "第112串"=0.0, "第113串"=0.0, "第114串"=0.0, "第115串"=0.0, "第116串"=0.0, "第117串"=0.0, "第118串"=0.0, "第119串"=0.0, "第120串"=0.0, "第一串 2"=0.0, "第一串 4"=0.0, "第一串 6"=0.0, "第一串 8"=0.0, "第一串 10"=0.0, "第一串 12"=0.0, "第一串 14"=0.0, "第一串 16"=0.0, "第一串 18"=0.0, "第一串 20"=0.0, "第一串 22"=0.0, "第一串 24"=0.0}, "1 28"={"第121串"=0.0, "第122串"=0.0, "第123串"=0.0, "第124串"=0.0, "第125串"=0.0, "第126串"=0.0, "第127串"=0.0, "第128串"=0.0, "第129串"=0.0, "第130串"=0.0, "第131串"=0.0, "第132串"=0.0, "第一串 2"=0.0, "第一串 4"=0.0, "第一串 6"=0.0, "第一串 8"=0.0, "第一串 10"=0.0, "第一串 12"=0.0, "第一串 14"=0.0, "第一串 16"=0.0, "第一串 18"=0.0, "第一串 20"=0.0, "第一串 22"=0.0, "第一串 24"=0.0}, "1 29"={"第133串"=0.0, "第134串"=0.0, "第135串"=0.0, "第136串"=0.0, "第137串"=0.0, "第138串"=0.0, "第139串"=0.0, "第140串"=0.0, "第141串"=0.0, "第142串"=0.0, "第143串"=0.0, "第144串"=0.0, "第一串 2"=0.0, "第一串 4"=0.0, "第一串 6"=0.0, "第一串 8"=0.0, "第一串 10"=0.0, "第一串 12"=0.0, "第一串 14"=0.0, "第一串 16"=0.0, "第一串 18"=0.0, "第一串 20"=0.0, "第一串 22"=0.0, "第一串 24"=0.0}, "1 30"={"第145串"=0.0, "第146串"=0.0, "第147串"=0.0, "第148串"=0.0, "第149串"=0.0, "第150串"=0.0, "第151串"=0.0, "第152串"=0.0, "第153串"=0.0, "第154串"=0.0, "第155串"=0.0, "第156串"=0.0, "第一串 2"=0.0, "第一串 4"=0.0, "第一串 6"=0.0, "第一串 8"=0.0, "第一串 10"=0.0, "第一串 12"=0.0, "第一串 14"=0.0, "第一串 16"=0.0, "第一串 18"=0.0, "第一串 20"=0.0, "第一串 22"=0.0, "第一串 24"=0.0}, "1 31"={"第157串"=0.0, "第158串"=0.0, "第159串"=0.0, "第160串"=0.0, "第161串"=0.0, "第162串"=0.0, "第163串"=0.0, "第164串"=0.0, "第165串"=0.0, "第166串"=0.0, "第167串"=0.0, "第168串"=0.0, "第一串 2"=0.0, "第一串 4"=0.0, "第一串 6"=0.0, "第一串 8"=0.0, "第一串 10"=0.0, "第一串 12"=0.0, "第一串 14"=0.0, "第一串 16"=0.0, "第一串 18"=0.0, "第一串 20"=0.0, "第一串 22"=0.0, "第一串 24"=0.0}, "1 32"={"第169串"=0.0, "第170串"=0.0, "第171串"=0.0, "第172串"=0.0, "第173串"=0.0, "第174串"=0.0, "第175串"=0.0, "第176串"=0.0, "第177串"=0.0, "第178串"=0.0, "第179串"=0.0, "第180串"=0.0, "第一串 2"=0.0, "第一串 4"=0.0, "第一串 6"=0.0, "第一串 8"=0.0, "第一串 10"=0.0, "第一串 12"=0.0, "第一串 14"=0.0, "第一串 16"=0.0, "第一串 18"=0.0, "第一串 20"=0.0, "第一串 22"=0.0, "第一串 24"=0.0}, "1 33"={"第181串"=0.0, "第182串"=0.0, "第183串"=0.0, "第184串"=0.0, "第185串"=0.0, "第186串"=0.0, "第187串"=0.0, "第188串"=0.0, "第189串"=0.0, "第190串"=0.0, "第191串"=0.0, "第192串"=0.0, "第一串 2"=0.0, "第一串 4"=0.0, "第一串 6"=0.0, "第一串 8"=0.0, "第一串 10"=0.0, "第一串 12"=0.0, "第一串 14"=0.0, "第一串 16"=0.0, "第一串 18"=0.0, "第一串 20"=0.0, "第一串 22"=0.0, "第一串 24"=0.0}, "1 16"={"充电1"=13816530, "充电1"=13816530, "充电1"=13816530, "充电1"=13816530, "充电1"=13816530, "充电1"=13816530, "充电1"=13816530, "充电1"=13816530, "充电1"=13816530, "充电1"=13816530, "充电1"=13816530, "充电1"=13816530}, "1 44"={"充电1"=13816530, "充电1"=13816530, "充电1"=13816530, "充电1"=13816530, "充电1"=13816530, "充电1"=13816530, "充电1"=13816530, "充电1"=13816530, "充电1"=13816530, "充电1"=13816530, "充电1"=13816530, "充电1"=13816530}, "1 36"={"充电1"=13816530, "充电1"=13816530, "充电1"=13816530, "充电1"=13816530, "充电1"=13816530, "充电1"=13816530, "充电1"=13816530, "充电1"=13816530, "充电1"=13816530, "充电1"=13816530, "充电1"=13816530, "充电1"=13816530}, "1 47"={"充电1"=13816530, "充电1"=13816530, "充电1"=13816530, "充电1"=13816530, "充电1"=13816530, "充电1"=13816530, "充电1"=13816530, "充电1"=13816530, "充电1"=13816530, "充电1"=13816530, "充电1"=13816530, "充电1"=13816530}, "1 19"={"充电1"=13816530, "充电1"=13816530, "充电1"=13816530, "充电1"=13816530, "充电1"=13816530, "充电1"=13816530, "充电1"=13816530, "充电1"=13816530, "充电1"=13816530, "充电1"=13816530, "充电1"=13816530, "充电1"=13816530}, "1 38"={"充电1"=13816530, "充电1"=13816530, "充电1"=13816530, "充电1"=13816530, "充电1"=13816530, "充电1"=13816530, "充电1"=13816530, "充电1"=13816530, "充电1"=13816530, "充电1"=13816530, "充电1"=13816530, "充电1"=13816530}, "1 41"={"充电1"=13816530, "充电1"=13816530, "充电1"=13816530, "充电1"=13816530, "充电1"=13816530, "充电1"=13816530, "充电1"=13816530, "充电1"=13816530, "充电1"=13816530, "充电1"=13816530, "充电1"=13816530, "充电1"=13816530}, "1 50"={"充电1"=13816530, "充电1"=13816530, "充电1"=13816530, "充电1"=13816530, "充电1"=13816530, "充电1"=13816530, "充电1"=13816530, "充电1"=13816530, "充电1"=13816530, "充电1"=13816530, "充电1"=13816530, "充电1"=13816530}, "1 15"={"充电1"=13816530, "充电1"=13816530, "充电1"=13816530, "充电1"=13816530, "充电1"=13816530, "充电1"=13816530, "充电1"=13816530, "充电1"=13816530, "充电1"=13816530, "充电1"=13816530, "充电1"=13816530, "充电1"=13816530}, "1 43"={"充电1"=13816530, "充电1"=13816530, "充电1"=13816530, "充电1"=13816530, "充电1"=13816530, "充电1"=13816530, "充电1"=13816530, "充电1"=13816530, "充电1"=13816530, "充电1"=13816530, "充电1"=13816530, "充电1"=13816530}, "1 35"={"充电1"=13816530, "充电1"=13816530, "充电1"=13816530, "充电1"=13816530, "充电1"=13816530, "充电1"=13816530, "充电1"=13816530, "充电1"=13816530, "充电1"=13816530, "充电1"=13816530, "充电1"=13816530, "充电1"=13816530}, "1 46"={"充电1"=13816530, "充电1"=13816530, "充电1"=13816530, "充电1"=13816530, "充电1"=13816530, "充电1"=13816530, "充电1"=13816530, "充电1"=13816530, "充电1"=13816530, "充电1"=13816530, "充电1"=13816530, "充电1"=13816530}, "1 18"={"充电1"=13816530, "充电1"=13816530, "充电1"=13816530, "充电1"=13816530, "充电1"=13816530, "充电1"=13816530, "充电1"=13816530, "充电1"=13816530, "充电1"=13816530, "充电1"=13816530, "充电1"=13816530, "充电1"=13816530}, "1 37"={"充电1"=13816530, "充电1"=13816530, "充电1"=13816530, "充电1"=13816530, "充电1"=13816530, "充电1"=13816530, "充电1"=13816530, "充电1"=13816530, "充电1"=13816530, "充电1"=13816530, "充电1"=13816530, "充电1"=13816530}, "1 40"={"充电1"=13816530, "充电1"=13816530, "充电1"=13816530, "充电1"=13816530, "充电1"=13816530, "充电1"=13816530, "充电1"=13816530, "充电1"=13816530, "充电1"=13816530, "充电1"=13816530, "充电1"=13816530, "充电1"=13816530}, "1 49"={"充电1"=13816530, "充电1"=13816530, "充电1"=13816530, "充电1"=13816530, "充电1"=13816530, "充电1"=13816530, "充电1"=13816530, "充电1"=13816530, "充电1"=13816530, "充电1"=13816530, "充电1"=13816530, "充电1"=13816530}, "1 14"={"均衡故障"=15, "均衡故障 2"=0.0, "均衡故障 3"=0.0, "均衡故障 4"=0.0, "均衡故障 5"=0.0, "均衡故障 6"=0.0, "均衡故障 7"=0.0, "均衡故障 8"=0.0, "均衡故障 9"=0.0, "均衡故障 10"=0.0, "均衡故障 11"=0.0, "均衡故障 12"=0.0}, "1 42"={"均衡故障"=15, "均衡故障 2"=0.0, "均衡故障 3"=0.0, "均衡故障 4"=0.0, "均衡故障 5"=0.0, "均衡故障 6"=0.0, "均衡故障 7"=0.0, "均衡故障 8"=0.0, "均衡故障 9"=0.0, "均衡故障 10"=0.0, "均衡故障 11"=0.0, "均衡故障 12"=0.0}, "1 34"={"均衡故障"=15, "均衡故障 2"=0.0, "均衡故障 3"=0.0, "均衡故障 4"=0.0, "均衡故障 5"=0.0, "均衡故障 6"=0.0, "均衡故障 7"=0.0, "均衡故障 8"=0.0, "均衡故障 9"=0.0, "均衡故障 10"=0.0, "均衡故障 11"=0.0, "均衡故障 12"=0.0}, "1 45"={"均衡故障"=15, "均衡故障 2"=0.0, "均衡故障 3"=0.0, "均衡故障 4"=0.0, "均衡故障 5"=0.0, "均衡故障 6"=0.0, "均衡故障 7"=0.0, "均衡故障 8"=0.0, "均衡故障 9"=0.0, "均衡故障 10"=0.0, "均衡故障 11"=0.0, "均衡故障 12"=0.0}, "1 17"={"均衡故障"=15, "均衡故障 2"=0.0, "均衡故障 3"=0.0, "均衡故障 4"=0.0, "均衡故障 5"=0.0, "均衡故障 6"=0.0, "均衡故障 7"=0.0, "均衡故障 8"=0.0, "均衡故障 9"=0.0, "均衡故障 10"=0.0, "均衡故障 11"=0.0, "均衡故障 12"=0.0}, "1 20"={"均衡故障"=15, "均衡故障 2"=0.0, "均衡故障 3"=0.0, "均衡故障 4"=0.0, "均衡故障 5"=0.0, "均衡故障 6"=0.0, "均衡故障 7"=0.0, "均衡故障 8"=0.0, "均衡故障 9"=0.0, "均衡故障 10"=0.0, "均衡故障 11"=0.0, "均衡故障 12"=0.0}, "1 39"={"均衡故障"=15, "均衡故障 2"=0.0, "均衡故障 3"=0.0, "均衡故障 4"=0.0, "均衡故障 5"=0.0, "均衡故障 6"=0.0, "均衡故障 7"=0.0, "均衡故障 8"=0.0, "均衡故障 9"=0.0, "均衡故障 10"=0.0, "均衡故障 11"=0.0, "均衡故障 12"=0.0}, "1 48"={"均衡故障"=15, "均衡故障 2"=0.0, "均衡故障 3"=0.0, "均衡故障 4"=0.0, "均衡故障 5"=0.0, "均衡故障 6"=0.0, "均衡故障 7"=0.0, "均衡故障 8"=0.0, "均衡故障 9"=0.0, "均衡故障 10"=0.0, "均衡故障 11"=0.0, "均衡故障 12"=0.0}} {"1 33"."第192串" format="%.3f"; "1 33"."第191串" format="%.3f"; "1 33"."第190串" format="%.3f"; "1 33"."第189串" format="%.3f"; "1 33"."第188串" format="%.3f"; "1 33"."第187串" format="%.3f"; "1 33"."第186串" format="%.3f"; "1 33"."第185串" format="%.3f"; "1 33"."第184串" format="%.3f"; "1 33"."第183串" format="%.3f"; "1 33"."第182串" format="%.3f"; "1 33"."第181串" format="%.3f"; "1 32"."第180串" format="%.3f"; "1 32"."第179串" format="%.3f"; "1 32"."第178串" format="%.3f"; "1 32"."第177串" format="%.3f"; "1 32"."第176串" format="%.3f"; "1 32"."第175串" format="%.3f"; "1 32"."第174串" format="%.3f"; "1 32"."第173串" format="%.3f"; "1 32"."第172串" format="%.3f"; "1 32"."第171串" format="%.3f"; "1 32"."第170串" format="%.3f"; "1 32"."第169串" format="%.3f"; "1 31"."第168串" format="%.3f"; "1 31"."第167串" format="%.3f"; "1 31"."第166串" format="%.3f"; "1 31"."第165串" format="%.3f"; "1 31"."第164串" format="%.3f"; "1 31"."第163串" format="%.3f"; "1 31"."第162串" format="%.3f"; "1 31"."第161串" format="%.3f"; "1 31"."第160串" format="%.3f"; "1 31"."第159串" format="%.3f"; "1 31"."第158串" format="%.3f"; "1 31"."第157串" format="%.3f"; "1 30"."第156串" format="%.3f"; "1 30"."第155串" format="%.3f"; "1 30"."第154串" format="%.3f"; "1 30"."第153串" format="%.3f"; "1 30"."第152串" format="%.3f"; "1 30"."第151串" format="%.3f"; "1 30"."第150串" format="%.3f"; "1 30"."第149串" format="%.3f"; "1 30"."第148串" format="%.3f"; "1 30"."第147串" format="%.3f"; "1 30"."第146串" format="%.3f"; "1 30"."第145串" format="%.3f"; "1 29"."第144串" format="%.3f"; "1 29"."第143串" format="%.3f"; "1 29"."第142串" format="%.3f"; "1 29"."第141串" format="%.3f"; "1 29"."第140串" format="%.3f"; "1 29"."第139串" format="%.3f"; "1 29"."第138串" format="%.3f"; "1 29"."第137串" format="%.3f"; "1 29"."第136串" format="%.3f"; "1 29"."第135串" format="%.3f"; "1 29"."第134串" format="%.3f"; "1 29"."第133串" format="%.3f"; "1 28"."第132串" format="%.3f"; "1 28"."第131串" format="%.3f"; "1 28"."第130串" format="%.3f"; "1 28"."第129串" format="%.3f"; "1 28"."第128串" format="%.3f"; "1 28"."第127串" format="%.3f"; "1 28"."第126串" format="%.3f"; "1 28"."第125串" format="%.3f"; "1 28"."第124串" format="%.3f"; "1 28"."第123串" format="%.3f"; "1 28"."第122串" format="%.3f"; "1 28"."第121串" format="%.3f"; "1 27"."第120串" format="%.3f"; "1 27"."第119串" format="%.3f"; "1 27"."第118串" format="%.3f"; "1 27"."第117串" format="%.3f"; "1 27"."第116串" format="%.3f"; "1 27"."第115串" format="%.3f"; "1 27"."第114串" format="%.3f"; "1 27"."第113串" format="%.3f"; "1 27"."第112串" format="%.3f"; "1 27"."第111串" format="%.3f"; "1 27"."第110串" format="%.3f"; "1 27"."第109串" format="%.3f"; "1 26"."第一串 24" format="%#.2f"; "1 26"."第108串" format="%.3f"; "1 26"."第一串 22" format="%#.2f"; "1 26"."第107串" format="%.3f"; "1 26"."第一串 20" format="%#.2f"; "1 26"."第106串" format="%.3f"; "1 26"."第一串 18" format="%#.2f"; "1 26"."第105串" format="%.3f"; "1 26"."第一串 16" format="%#.2f"; "1 26"."第104串" format="%.3f"; "1 26"."第一串 14" format="%#.2f"; "1 26"."第103串" format="%.3f"; "1 26"."第一串 12" format="%#.2f"; "1 26"."第102串" format="%.3f"; "1 26"."第一串 10" format="%#.2f"; "1 26"."第101串" format="%.3f"; "1 26"."第一串 8" format="%#.2f"; "1 26"."第100串" format="%.3f"; "1 26"."第一串 6" format="%#.2f"; "1 26"."第99串" format="%.3f"; "1 26"."第一串 4" format="%#.2f"; "1 26"."第98串" format="%.3f"; "1 26"."第一串 2" format="%#.2f"; "1 26"."第97串" format="%.3f"}
  out "3":T6={"1 18"={"第193串"=0.0, "第194串"=0.0, "第195串"=0.0, "第196串"=0.0, "第197串"=0.0, "第198串"=0.0, "第199串"=0.0, "第200串"=0.0, "第201串"=0.0, "第202串"=0.0, "第203串"=0.0, "第204串"=0.0, "第一串 2"=0.0, "第一串 4"=0.0, "第一串 6"=0.0, "第一串 8"=0.0, "第一串 10"=0.0, "第一串 12"=0.0, "第一串 14"=0.0, "第一串 16"=0.0, "第一串 18"=0.0, "第一串 20"=0.0, "第一串 22"=0.0, "第一串 24"=0.0}, "1 19"={"第205串"=0.0, "第206串"=0.0, "第207串"=0.0, "第208串"=0.0, "第209串"=0.0, "第210串"=0.0, "第211串"=0.0, "第212串"=0.0, "第213串"=0.0, "第214串"=0.0, "第215串"=0.0, "第216串"=0.0, "第一串 2"=0.0, "第一串 4"=0.0, "第一串 6"=0.0, "第一串 8"=0.0, "第一串 10"=0.0, "第一串 12"=0.0, "第一串 14"=0.0, "第一串 16"=0.0, "第一串 18"=0.0, "第一串 20"=0.0, "第一串 22"=0.0, "第一串 24"=0.0}, "1 20"={"第217串"=0.0, "第218串"=0.0, "第219串"=0.0, "第220串"=0.0, "第221串"=0.0, "第222串"=0.0, "第223串"=0.0, "第224串"=0.0, "第225串"=0.0, "第226串"=0.0, "第227串"=0.0, "第228串"=0.0, "第一串 2"=0.0, "第一串 4"=0.0, "第一串 6"=0.0, "第一串 8"=0.0, "第一串 10"=0.0, "第一串 12"=0.0, "第一串 14"=0.0, "第一串 16"=0.0, "第一串 18"=0.0, "第一串 20"=0.0, "第一串 22"=0.0, "第一串 24"=0.0}, "1 21"={"第229串"=0.0, "第230串"=0.0, "第231串"=0.0, "第232串"=0.0, "第233串"=0.0, "第234串"=0.0, "第235串"=0.0, "第236串"=0.0, "第237串"=0.0, "第238串"=0.0, "第239串"=0.0, "第240串"=0.0, "第一串 2"=0.0, "第一串 4"=0.0, "第一串 6"=0.0, "第一串 8"=0.0, "第一串 10"=0.0, "第一串 12"=0.0, "第一串 14"=0.0, "第一串 16"=0.0, "第一串 18"=0.0, "第一串 20"=0.0, "第一串 22"=0.0, "第一串 24"=0.0}, "1 22"={"第241串"=0.0, "第242串"=0.0, "第243串"=0.0, "第244串"=0.0, "第245串"=0.0, "第246串"=0.0, "第247串"=0.0, "第248串"=0.0, "第249串"=0.0, "第250串"=0.0, "第251串"=0.0, "第252串"=0.0, "第一串 2"=0.0, "第一串 4"=0.0, "第一串 6"=0.0, "第一串 8"=0.0, "第一串 10"=0.0, "第一串 12"=0.0, "第一串 14"=0.0, "第一串 16"=0.0, "第一串 18"=0.0, "第一串 20"=0.0, "第一串 22"=0.0, "第一串 24"=0.0}, "1 23"={"第253串"=0.0, "第254串"=0.0, "第255串"=0.0, "第256串"=0.0, "第257串"=0.0, "第258串"=0.0, "第259串"=0.0, "第260串"=0.0, "第261串"=0.0, "第262串"=0.0, "第263串"=0.0, "第264串"=0.0, "第一串 2"=0.0, "第一串 4"=0.0, "第一串 6"=0.0, "第一串 8"=0.0, "第一串 10"=0.0, "第一串 12"=0.0, "第一串 14"=0.0, "第一串 16"=0.0, "第一串 18"=0.0, "第一串 20"=0.0, "第一串 22"=0.0, "第一串 24"=0.0}, "1 24"={"第265串"=0.0, "第266串"=0.0, "第267串"=0.0, "第268串"=0.0, "第269串"=0.0, "第270串"=0.0, "第271串"=0.0, "第272串"=0.0, "第273串"=0.0, "第274串"=0.0, "第275串"=0.0, "第276串"=0.0, "第一串 2"=0.0, "第一串 4"=0.0, "第一串 6"=0.0, "第一串 8"=0.0, "第一串 10"=0.0, "第一串 12"=0.0, "第一串 14"=0.0, "第一串 16"=0.0, "第一串 18"=0.0, "第一串 20"=0.0, "第一串 22"=0.0, "第一串 24"=0.0}, "1 25"={"第277串"=0.0, "第278串"=0.0, "第279串"=0.0, "第280串"=0.0, "第281串"=0.0, "第282串"=0.0, "第283串"=0.0, "第284串"=0.0, "第285串"=0.0, "第286串"=0.0, "第287串"=0.0, "第288串"=0.0, "第一串 2"=0.0, "第一串 4"=0.0, "第一串 6"=0.0, "第一串 8"=0.0, "第一串 10"=0.0, "第一串 12"=0.0, "第一串 14"=0.0, "第一串 16"=0.0, "第一串 18"=0.0, "第一串 20"=0.0, "第一串 22"=0.0, "第一串 24"=0.0}, "1 12"={"充电1"=13816530, "充电1"=13816530, "充电1"=13816530, "充电1"=13816530, "充电1"=13816530, "充电1"=13816530, "充电1"=13816530, "充电1"=13816530, "充电1"=13816530, "充电1"=13816530, "充电1"=13816530, "充电1"=13816530}, "1 39"={"充电1"=13816530, "充电1"=13816530, "充电1"=13816530, "充电1"=13816530, "充电1"=13816530, "充电1"=13816530, "充电1"=13816530, "充电1"=13816530, "充电1"=13816530, "充电1"=13816530, "充电1"=13816530, "充电1"=13816530}, "1 28"={"充电1"=13816530, "充电1"=13816530, "充电1"=13816530, "充电1"=13816530, "充电1"=13816530, "充电1"=13816530, "充电1"=13816530, "充电1"=13816530, "充电1"=13816530, "充电1"=13816530, "充电1"=13816530, "充电1"=13816530}, "1 42"={"充电1"=13816530, "充电1"=13816530, "充电1"=13816530, "充电1"=13816530, "充电1"=13816530, "充电1"=13816530, "充电1"=13816530, "充电1"=13816530, "充电1"=13816530, "充电1"=13816530, "充电1"=13816530, "充电1"=13816530}, "1 16"={"充电1"=13816530, "充电1"=13816530, "充电1"=13816530, "充电1"=13816530, "充电1"=13816530, "充电1"=13816530, "充电1"=13816530, "充电1"=13816530, "充电1"=13816530, "充电1"=13816530, "充电1"=13816530, "充电1"=13816530}, "1 30"={"充电1"=13816530, "充电1"=13816530, "充电1"=13816530, "充电1"=13816530, "充电1"=13816530, "充电1"=13816530, "充电1"=13816530, "充电1"=13816530, "充电1"=13816530, "充电1"=13816530, "充电1"=13816530, "充电1"=13816530}, "1 33"={"充电1"=13816530, "充电1"=13816530, "充电1"=13816530, "充电1"=13816530, "充电1"=13816530, "充电1"=13816530, "充电1"=13816530, "充电1"=13816530, "充电1"=13816530, "充电1"=13816530, "充电1"=13816530, "充电1"=13816530}, "1 36"={"充电1"=13816530, "充电1"=13816530, "充电1"=13816530, "充电1"=13816530, "充电1"=13816530, "充电1"=13816530, "充电1"=13816530, "充电1"=13816530, "充电1"=13816530, "充电1"=13816530, "充电1"=13816530, "充电1"=13816530}, "1 11"={"充电1"=13816530, "充电1"=13816530, "充电1"=13816530, "充电1"=13816530, "充电1"=13816530, "充电1"=13816530, "充电1"=13816530, "充电1"=13816530, "充电1"=13816530, "充电1"=13816530, "充电1"=13816530, "充电1"=13816530}, "1 38"={"充电1"=13816530, "充电1"=13816530, "充电1"=13816530, "充电1"=13816530, "充电1"=13816530, "充电1"=13816530, "充电1"=13816530, "充电1"=13816530, "充电1"=13816530, "充电1"=13816530, "充电1"=13816530, "充电1"=13816530}, "1 27"={"充电1"=13816530, "充电1"=13816530, "充电1"=13816530, "充电1"=13816530, "充电1"=13816530, "充电1"=13816530, "充电1"=13816530, "充电1"=13816530, "充电1"=13816530, "充电1"=13816530, "充电1"=13816530, "充电1"=13816530}, "1 41"={"充电1"=13816530, "充电1"=13816530, "充电1"=13816530, "充电1"=13816530, "充电1"=13816530, "充电1"=13816530, "充电1"=13816530, "充电1"=13816530, "充电1"=13816530, "充电1"=13816530, "充电1"=13816530, "充电1"=13816530}, "1 15"={"充电1"=13816530, "充电1"=13816530, "充电1"=13816530, "充电1"=13816530, "充电1"=13816530, "充电1"=13816530, "充电1"=13816530, "充电1"=13816530, "充电1"=13816530, "充电1"=13816530, "充电1"=13816530, "充电1"=13816530}, "1 29"={"充电1"=13816530, "充电1"=13816530, "充电1"=13816530, "充电1"=13816530, "充电1"=13816530, "充电1"=13816530, "充电1"=13816530, "充电1"=13816530, "充电1"=13816530, "充电1"=13816530, "充电1"=13816530, "充电1"=13816530}, "1 32"={"充电1"=13816530, "充电1"=13816530, "充电1"=13816530, "充电1"=13816530, "充电1"=13816530, "充电1"=13816530, "充电1"=13816530, "充电1"=13816530, "充电1"=13816530, "充电1"=13816530, "充电1"=13816530, "充电1"=13816530}, "1 35"={"充电1"=13816530, "充电1"=13816530, "充电1"=13816530, "充电1"=13816530, "充电1"=13816530, "充电1"=13816530, "充电1"=13816530, "充电1"=13816530, "充电1"=13816530, "充电1"=13816530, "充电1"=13816530, "充电1"=13816530}, "1 13"={"均衡故障"=0, "均衡故障 2"=0.0, "均衡故障 3"=0.0, "均衡故障 4"=0.0, "均衡故障 5"=0.0, "均衡故障 6"=0.0, "均衡故障 7"=0.0, "均衡故障 8"=0.0, "均衡故障 9"=0.0, "均衡故障 10"=0.0, "均衡故障 11"=0.0, "均衡故障 12"=0.0}, "1 37"={"均衡故障"=0, "均衡故障 2"=0.0, "均衡故障 3"=0.0, "均衡故障 4"=0.0, "均衡故障 5"=0.0, "均衡故障 6"=0.0, "均衡故障 7"=0.0, "均衡故障 8"=0.0, "均衡故障 9"=0.0, "均衡故障 10"=0.0, "均衡故障 11"=0.0, "均衡故障 12"=0.0}, "1 26"={"均衡故障"=0, "均衡故障 2"=0.0, "均衡故障 3"=0.0, "均衡故障 4"=0.0, "均衡故障 5"=0.0, "均衡故障 6"=0.0, "均衡故障 7"=0.0, "均衡故障 8"=0.0, "均衡故障 9"=0.0, "均衡故障 10"=0.0, "均衡故障 11"=0.0, "均衡故障 12"=0.0}, "1 40"={"均衡故障"=0, "均衡故障 2"=0.0, "均衡故障 3"=0.0, "均衡故障 4"=0.0, "均衡故障 5"=0.0, "均衡故障 6"=0.0, "均衡故障 7"=0.0, "均衡故障 8"=0.0, "均衡故障 9"=0.0, "均衡故障 10"=0.0, "均衡故障 11"=0.0, "均衡故障 12"=0.0}, "1 14"={"均衡故障"=0, "均衡故障 2"=0.0, "均衡故障 3"=0.0, "均衡故障 4"=0.0, "均衡故障 5"=0.0, "均衡故障 6"=0.0, "均衡故障 7"=0.0, "均衡故障 8"=0.0, "均衡故障 9"=0.0, "均衡故障 10"=0.0, "均衡故障 11"=0.0, "均衡故障 12"=0.0}, "1 17"={"均衡故障"=0, "均衡故障 2"=0.0, "均衡故障 3"=0.0, "均衡故障 4"=0.0, "均衡故障 5"=0.0, "均衡故障 6"=0.0, "均衡故障 7"=0.0, "均衡故障 8"=0.0, "均衡故障 9"=0.0, "均衡故障 10"=0.0, "均衡故障 11"=0.0, "均衡故障 12"=0.0}, "1 31"={"均衡故障"=0, "均衡故障 2"=0.0, "均衡故障 3"=0.0, "均衡故障 4"=0.0, "均衡故障 5"=0.0, "均衡故障 6"=0.0, "均衡故障 7"=0.0, "均衡故障 8"=0.0, "均衡故障 9"=0.0, "均衡故障 10"=0.0, "均衡故障 11"=0.0, "均衡故障 12"=0.0}, "1 34"={"均衡故障"=0, "均衡故障 2"=0.0, "均衡故障 3"=0.0, "均衡故障 4"=0.0, "均衡故障 5"=0.0, "均衡故障 6"=0.0, "均衡故障 7"=0.0, "均衡故障 8"=0.0, "均衡故障 9"=0.0, "均衡故障 10"=0.0, "均衡故障 11"=0.0, "均衡故障 12"=0.0}} {"1 25"."第288串" format="%.3f"; "1 25"."第287串" format="%.3f"; "1 25"."第286串" format="%.3f"; "1 25"."第285串" format="%.3f"; "1 25"."第284串" format="%.3f"; "1 25"."第283串" format="%.3f"; "1 25"."第282串" format="%.3f"; "1 25"."第281串" format="%.3f"; "1 25"."第280串" format="%.3f"; "1 25"."第279串" format="%.3f"; "1 25"."第278串" format="%.3f"; "1 25"."第277串" format="%.3f"; "1 24"."第276串" format="%.3f"; "1 24"."第275串" format="%.3f"; "1 24"."第274串" format="%.3f"; "1 24"."第273串" format="%.3f"; "1 24"."第272串" format="%.3f"; "1 24"."第271串" format="%.3f"; "1 24"."第270串" format="%.3f"; "1 24"."第269串" format="%.3f"; "1 24"."第268串" format="%.3f"; "1 24"."第267串" format="%.3f"; "1 24"."第266串" format="%.3f"; "1 24"."第265串" format="%.3f"; "1 23"."第264串" format="%.3f"; "1 23"."第263串" format="%.3f"; "1 23"."第262串" format="%.3f"; "1 23"."第261串" format="%.3f"; "1 23"."第260串" format="%.3f"; "1 23"."第259串" format="%.3f"; "1 23"."第258串" format="%.3f"; "1 23"."第257串" format="%.3f"; "1 23"."第256串" format="%.3f"; "1 23"."第255串" format="%.3f"; "1 23"."第254串" format="%.3f"; "1 23"."第253串" format="%.3f"; "1 22"."第252串" format="%.3f"; "1 22"."第251串" format="%.3f"; "1 22"."第250串" format="%.3f"; "1 22"."第249串" format="%.3f"; "1 22"."第248串" format="%.3f"; "1 22"."第247串" format="%.3f"; "1 22"."第246串" format="%.3f"; "1 22"."第245串" format="%.3f"; "1 22"."第244串" format="%.3f"; "1 22"."第243串" format="%.3f"; "1 22"."第242串" format="%.3f"; "1 22"."第241串" format="%.3f"; "1 21"."第240串" format="%.3f"; "1 21"."第239串" format="%.3f"; "1 21"."第238串" format="%.3f"; "1 21"."第237串" format="%.3f"; "1 21"."第236串" format="%.3f"; "1 21"."第235串" format="%.3f"; "1 21"."第234串" format="%.3f"; "1 21"."第233串" format="%.3f"; "1 21"."第232串" format="%.3f"; "1 21"."第231串" format="%.3f"; "1 21"."第230串" format="%.3f"; "1 21"."第229串" format="%.3f"; "1 20"."第228串" format="%.3f"; "1 20"."第227串" format="%.3f"; "1 20"."第226串" format="%.3f"; "1 20"."第225串" format="%.3f"; "1 20"."第224串" format="%.3f"; "1 20"."第223串" format="%.3f"; "1 20"."第222串" format="%.3f"; "1 20"."第221串" format="%.3f"; "1 20"."第220串" format="%.3f"; "1 20"."第219串" format="%.3f"; "1 20"."第218串" format="%.3f"; "1 20"."第217串" format="%.3f"; "1 19"."第216串" format="%.3f"; "1 19"."第215串" format="%.3f"; "1 19"."第214串" format="%.3f"; "1 19"."第213串" format="%.3f"; "1 19"."第212串" format="%.3f"; "1 19"."第211串" format="%.3f"; "1 19"."第210串" format="%.3f"; "1 19"."第209串" format="%.3f"; "1 19"."第208串" format="%.3f"; "1 19"."第207串" format="%.3f"; "1 19"."第206串" format="%.3f"; "1 19"."第205串" format="%.3f"; "1 18"."第一串 24" format="%#.2f"; "1 18"."第204串" format="%.3f"; "1 18"."第一串 22" format="%#.2f"; "1 18"."第203串" format="%.3f"; "1 18"."第一串 20" format="%#.2f"; "1 18"."第202串" format="%.3f"; "1 18"."第一串 18" format="%#.2f"; "1 18"."第201串" format="%.3f"; "1 18"."第一串 16" format="%#.2f"; "1 18"."第200串" format="%.3f"; "1 18"."第一串 14" format="%#.2f"; "1 18"."第199串" format="%.3f"; "1 18"."第一串 12" format="%#.2f"; "1 18"."第198串" format="%.3f"; "1 18"."第一串 10" format="%#.2f"; "1 18"."第197串" format="%.3f"; "1 18"."第一串 8" format="%#.2f"; "1 18"."第196串" format="%.3f"; "1 18"."第一串 6" format="%#.2f"; "1 18"."第195串" format="%.3f"; "1 18"."第一串 4" format="%#.2f"; "1 18"."第194串" format="%.3f"; "1 18"."第一串 2" format="%#.2f"; "1 18"."第193串" format="%.3f"}
  out "1 5":T7 {"第一串 24" format="%#.2f"; "第300串" format="%.3f"; "第一串 22" format="%#.2f"; "第299串" format="%.3f"; "第一串 20" format="%#.2f"; "第298串" format="%.3f"; "第一串 18" format="%#.2f"; "第297串" format="%.3f"; "第一串 16" format="%#.2f"; "第296串" format="%.3f"; "第一串 14" format="%#.2f"; "第295串" format="%.3f"; "第一串 12" format="%#.2f"; "第294串" format="%.3f"; "第一串 10" format="%#.2f"; "第293串" format="%.3f"; "第一串 8" format="%#.2f"; "第292串" format="%.3f"; "第一串 6" format="%#.2f"; "第291串" format="%.3f"; "第一串 4" format="%#.2f"; "第290串" format="%.3f"; "第一串 2" format="%#.2f"; "第289串" format="%.3f"}
  out "1 13":T8
  out "放电均衡":T9={"充电1"=13816530, "充电1"=13816530, "充电1"=13816530, "充电1"=13816530, "充电1"=13816530, "充电1"=13816530, "充电1"=13816530, "充电1"=13816530, "充电1"=13816530, "充电1"=13816530, "充电1"=13816530, "充电1"=13816530}
  out "充电均衡":T9={"充电1"=13816530, "充电1"=13816530, "充电1"=13816530, "充电1"=13816530, "充电1"=13816530, "充电1"=13816530, "充电1"=13816530, "充电1"=13816530, "充电1"=13816530, "充电1"=13816530, "充电1"=13816530, "充电1"=13816530}
  out "放电均衡":u32(colorbox)=6618880
  out "充电均衡":u32(colorbox)=16860
  in  "布尔":bool caption="判定"
  in  "故障信息选择按键 3":enum32{"单选选项2", "单选选项2 2", "单选选项2 3", "单选选项1"}(radio)=enum."单选选项1"
  out "电压选择 2":enum32{"1-96", "97-192", "193-288", "289-300"}(tab)
  out "4":T10 {"1 102"."第一串 24" format="%#.2f"; "1 102"."第12串" format="%#.2f"; "1 102"."第一串 22" format="%#.2f"; "1 102"."第11串" format="%#.2f"; "1 102"."第一串 20" format="%#.2f"; "1 102"."第10串" format="%#.2f"; "1 102"."第一串 18" format="%#.2f"; "1 102"."第9串" format="%#.2f"; "1 102"."第一串 16" format="%#.2f"; "1 102"."第8串" format="%#.2f"; "1 102"."第一串 14" format="%#.2f"; "1 102"."第7串" format="%#.2f"; "1 102"."第一串 12" format="%#.2f"; "1 102"."第6串" format="%#.2f"; "1 102"."第一串 10" format="%#.2f"; "1 102"."第5串" format="%#.2f"; "1 102"."第一串 8" format="%#.2f"; "1 102"."第4串" format="%#.2f"; "1 102"."第一串 6" format="%#.2f"; "1 102"."第3串" format="%#.2f"; "1 102"."第一串 4" format="%#.2f"; "1 102"."第2串" format="%#.2f"; "1 102"."第一串 2" format="%#.2f"; "1 102"."第1串" format="%#.2f"}
  out "5":T11 {"1 26"."第一串 24" format="%#.2f"; "1 26"."第108串" format="%#.2f"; "1 26"."第一串 22" format="%#.2f"; "1 26"."第107串" format="%#.2f"; "1 26"."第一串 20" format="%#.2f"; "1 26"."第106串" format="%#.2f"; "1 26"."第一串 18" format="%#.2f"; "1 26"."第105串" format="%#.2f"; "1 26"."第一串 16" format="%#.2f"; "1 26"."第104串" format="%#.2f"; "1 26"."第一串 14" format="%#.2f"; "1 26"."第103串" format="%#.2f"; "1 26"."第一串 12" format="%#.2f"; "1 26"."第102串" format="%#.2f"; "1 26"."第一串 10" format="%#.2f"; "1 26"."第101串" format="%#.2f"; "1 26"."第一串 8" format="%#.2f"; "1 26"."第100串" format="%#.2f"; "1 26"."第一串 6" format="%#.2f"; "1 26"."第99串" format="%#.2f"; "1 26"."第一串 4" format="%#.2f"; "1 26"."第98串" format="%#.2f"; "1 26"."第一串 2" format="%#.2f"; "1 26"."第97串" format="%#.2f"}
  out "6":T12 {"1 18"."第一串 24" format="%#.2f"; "1 18"."第204串" format="%#.2f"; "1 18"."第一串 22" format="%#.2f"; "1 18"."第203串" format="%#.2f"; "1 18"."第一串 20" format="%#.2f"; "1 18"."第202串" format="%#.2f"; "1 18"."第一串 18" format="%#.2f"; "1 18"."第201串" format="%#.2f"; "1 18"."第一串 16" format="%#.2f"; "1 18"."第200串" format="%#.2f"; "1 18"."第一串 14" format="%#.2f"; "1 18"."第199串" format="%#.2f"; "1 18"."第一串 12" format="%#.2f"; "1 18"."第198串" format="%#.2f"; "1 18"."第一串 10" format="%#.2f"; "1 18"."第197串" format="%#.2f"; "1 18"."第一串 8" format="%#.2f"; "1 18"."第196串" format="%#.2f"; "1 18"."第一串 6" format="%#.2f"; "1 18"."第195串" format="%#.2f"; "1 18"."第一串 4" format="%#.2f"; "1 18"."第194串" format="%#.2f"; "1 18"."第一串 2" format="%#.2f"; "1 18"."第193串" format="%#.2f"}
  out "1 6":T7 {"第一串 24" format="%#.2f"; "第300串" format="%#.2f"; "第一串 22" format="%#.2f"; "第299串" format="%#.2f"; "第一串 20" format="%#.2f"; "第298串" format="%#.2f"; "第一串 18" format="%#.2f"; "第297串" format="%#.2f"; "第一串 16" format="%#.2f"; "第296串" format="%#.2f"; "第一串 14" format="%#.2f"; "第295串" format="%#.2f"; "第一串 12" format="%#.2f"; "第294串" format="%#.2f"; "第一串 10" format="%#.2f"; "第293串" format="%#.2f"; "第一串 8" format="%#.2f"; "第292串" format="%#.2f"; "第一串 6" format="%#.2f"; "第291串" format="%#.2f"; "第一串 4" format="%#.2f"; "第290串" format="%#.2f"; "第一串 2" format="%#.2f"; "第289串" format="%#.2f"}
  in  "偏差":dbl=2.0 format="%#.0f"
  in  "基准":dbl=25.0 format="%#.0f"
  in  "布尔 2":bool caption="判定"
  in  "故障信息选择按键 4":enum32{"单选选项2", "单选选项2 2", "单选选项2 3", "单选选项1"}(radio)=enum."单选选项1"
  out "电压选择 3":enum32{"1-96", "97-192", "193-288", "289-300"}(tab)
  out "1 106":T13 {"1 102"."第一串 24" format="%#.2f"; "1 102"."第12串" format="%#.2f"; "1 102"."第一串 22" format="%#.2f"; "1 102"."第11串" format="%#.2f"; "1 102"."第一串 20" format="%#.2f"; "1 102"."第10串" format="%#.2f"; "1 102"."第一串 18" format="%#.2f"; "1 102"."第9串" format="%#.2f"; "1 102"."第一串 16" format="%#.2f"; "1 102"."第8串" format="%#.2f"; "1 102"."第一串 14" format="%#.2f"; "1 102"."第7串" format="%#.2f"; "1 102"."第一串 12" format="%#.2f"; "1 102"."第6串" format="%#.2f"; "1 102"."第一串 10" format="%#.2f"; "1 102"."第5串" format="%#.2f"; "1 102"."第一串 8" format="%#.2f"; "1 102"."第4串" format="%#.2f"; "1 102"."第一串 6" format="%#.2f"; "1 102"."第3串" format="%#.2f"; "1 102"."第一串 4" format="%#.2f"; "1 102"."第2串" format="%#.2f"; "1 102"."第一串 2" format="%#.2f"; "1 102"."第1串" format="%#.2f"}
  out "1 107":T11 {"1 26"."第一串 24" format="%#.2f"; "1 26"."第108串" format="%#.2f"; "1 26"."第一串 22" format="%#.2f"; "1 26"."第107串" format="%#.2f"; "1 26"."第一串 20" format="%#.2f"; "1 26"."第106串" format="%#.2f"; "1 26"."第一串 18" format="%#.2f"; "1 26"."第105串" format="%#.2f"; "1 26"."第一串 16" format="%#.2f"; "1 26"."第104串" format="%#.2f"; "1 26"."第一串 14" format="%#.2f"; "1 26"."第103串" format="%#.2f"; "1 26"."第一串 12" format="%#.2f"; "1 26"."第102串" format="%#.2f"; "1 26"."第一串 10" format="%#.2f"; "1 26"."第101串" format="%#.2f"; "1 26"."第一串 8" format="%#.2f"; "1 26"."第100串" format="%#.2f"; "1 26"."第一串 6" format="%#.2f"; "1 26"."第99串" format="%#.2f"; "1 26"."第一串 4" format="%#.2f"; "1 26"."第98串" format="%#.2f"; "1 26"."第一串 2" format="%#.2f"; "1 26"."第97串" format="%#.2f"}
  out "1 28":T12 {"1 18"."第一串 24" format="%#.2f"; "1 18"."第204串" format="%#.2f"; "1 18"."第一串 22" format="%#.2f"; "1 18"."第203串" format="%#.2f"; "1 18"."第一串 20" format="%#.2f"; "1 18"."第202串" format="%#.2f"; "1 18"."第一串 18" format="%#.2f"; "1 18"."第201串" format="%#.2f"; "1 18"."第一串 16" format="%#.2f"; "1 18"."第200串" format="%#.2f"; "1 18"."第一串 14" format="%#.2f"; "1 18"."第199串" format="%#.2f"; "1 18"."第一串 12" format="%#.2f"; "1 18"."第198串" format="%#.2f"; "1 18"."第一串 10" format="%#.2f"; "1 18"."第197串" format="%#.2f"; "1 18"."第一串 8" format="%#.2f"; "1 18"."第196串" format="%#.2f"; "1 18"."第一串 6" format="%#.2f"; "1 18"."第195串" format="%#.2f"; "1 18"."第一串 4" format="%#.2f"; "1 18"."第194串" format="%#.2f"; "1 18"."第一串 2" format="%#.2f"; "1 18"."第193串" format="%#.2f"}
  out "1 7":T7 {"第一串 24" format="%#.2f"; "第300串" format="%#.2f"; "第一串 22" format="%#.2f"; "第299串" format="%#.2f"; "第一串 20" format="%#.2f"; "第298串" format="%#.2f"; "第一串 18" format="%#.2f"; "第297串" format="%#.2f"; "第一串 16" format="%#.2f"; "第296串" format="%#.2f"; "第一串 14" format="%#.2f"; "第295串" format="%#.2f"; "第一串 12" format="%#.2f"; "第294串" format="%#.2f"; "第一串 10" format="%#.2f"; "第293串" format="%#.2f"; "第一串 8" format="%#.2f"; "第292串" format="%#.2f"; "第一串 6" format="%#.2f"; "第291串" format="%#.2f"; "第一串 4" format="%#.2f"; "第290串" format="%#.2f"; "第一串 2" format="%#.2f"; "第289串" format="%#.2f"}
  in  "故障信息选择按键 5":enum32{"单选选项2", "单选选项2 2", "单选选项2 3", "单选选项1"}(radio)=enum."单选选项1"
  out "电压选择 4":enum32{"1-96", "97-192", "193-288", "289-300"}(tab)
  out "1 108":T13 {"1 102"."第一串 24" format="%#.2f"; "1 102"."第12串" format="%#.2f"; "1 102"."第一串 22" format="%#.2f"; "1 102"."第11串" format="%#.2f"; "1 102"."第一串 20" format="%#.2f"; "1 102"."第10串" format="%#.2f"; "1 102"."第一串 18" format="%#.2f"; "1 102"."第9串" format="%#.2f"; "1 102"."第一串 16" format="%#.2f"; "1 102"."第8串" format="%#.2f"; "1 102"."第一串 14" format="%#.2f"; "1 102"."第7串" format="%#.2f"; "1 102"."第一串 12" format="%#.2f"; "1 102"."第6串" format="%#.2f"; "1 102"."第一串 10" format="%#.2f"; "1 102"."第5串" format="%#.2f"; "1 102"."第一串 8" format="%#.2f"; "1 102"."第4串" format="%#.2f"; "1 102"."第一串 6" format="%#.2f"; "1 102"."第3串" format="%#.2f"; "1 102"."第一串 4" format="%#.2f"; "1 102"."第2串" format="%#.2f"; "1 102"."第一串 2" format="%#.2f"; "1 102"."第1串" format="%#.2f"}
  out "1 109":T11 {"1 26"."第一串 24" format="%#.2f"; "1 26"."第108串" format="%#.2f"; "1 26"."第一串 22" format="%#.2f"; "1 26"."第107串" format="%#.2f"; "1 26"."第一串 20" format="%#.2f"; "1 26"."第106串" format="%#.2f"; "1 26"."第一串 18" format="%#.2f"; "1 26"."第105串" format="%#.2f"; "1 26"."第一串 16" format="%#.2f"; "1 26"."第104串" format="%#.2f"; "1 26"."第一串 14" format="%#.2f"; "1 26"."第103串" format="%#.2f"; "1 26"."第一串 12" format="%#.2f"; "1 26"."第102串" format="%#.2f"; "1 26"."第一串 10" format="%#.2f"; "1 26"."第101串" format="%#.2f"; "1 26"."第一串 8" format="%#.2f"; "1 26"."第100串" format="%#.2f"; "1 26"."第一串 6" format="%#.2f"; "1 26"."第99串" format="%#.2f"; "1 26"."第一串 4" format="%#.2f"; "1 26"."第98串" format="%#.2f"; "1 26"."第一串 2" format="%#.2f"; "1 26"."第97串" format="%#.2f"}
  out "1 29":T12 {"1 18"."第一串 24" format="%#.2f"; "1 18"."第204串" format="%#.2f"; "1 18"."第一串 22" format="%#.2f"; "1 18"."第203串" format="%#.2f"; "1 18"."第一串 20" format="%#.2f"; "1 18"."第202串" format="%#.2f"; "1 18"."第一串 18" format="%#.2f"; "1 18"."第201串" format="%#.2f"; "1 18"."第一串 16" format="%#.2f"; "1 18"."第200串" format="%#.2f"; "1 18"."第一串 14" format="%#.2f"; "1 18"."第199串" format="%#.2f"; "1 18"."第一串 12" format="%#.2f"; "1 18"."第198串" format="%#.2f"; "1 18"."第一串 10" format="%#.2f"; "1 18"."第197串" format="%#.2f"; "1 18"."第一串 8" format="%#.2f"; "1 18"."第196串" format="%#.2f"; "1 18"."第一串 6" format="%#.2f"; "1 18"."第195串" format="%#.2f"; "1 18"."第一串 4" format="%#.2f"; "1 18"."第194串" format="%#.2f"; "1 18"."第一串 2" format="%#.2f"; "1 18"."第193串" format="%#.2f"}
  out "1 8":T7 {"第一串 24" format="%#.2f"; "第300串" format="%#.2f"; "第一串 22" format="%#.2f"; "第299串" format="%#.2f"; "第一串 20" format="%#.2f"; "第298串" format="%#.2f"; "第一串 18" format="%#.2f"; "第297串" format="%#.2f"; "第一串 16" format="%#.2f"; "第296串" format="%#.2f"; "第一串 14" format="%#.2f"; "第295串" format="%#.2f"; "第一串 12" format="%#.2f"; "第294串" format="%#.2f"; "第一串 10" format="%#.2f"; "第293串" format="%#.2f"; "第一串 8" format="%#.2f"; "第292串" format="%#.2f"; "第一串 6" format="%#.2f"; "第291串" format="%#.2f"; "第一串 4" format="%#.2f"; "第290串" format="%#.2f"; "第一串 2" format="%#.2f"; "第289串" format="%#.2f"}
  out "单选选项2":bool
  # "主板详细信息"
  # "主板详细信息"
  # "监控上位机"
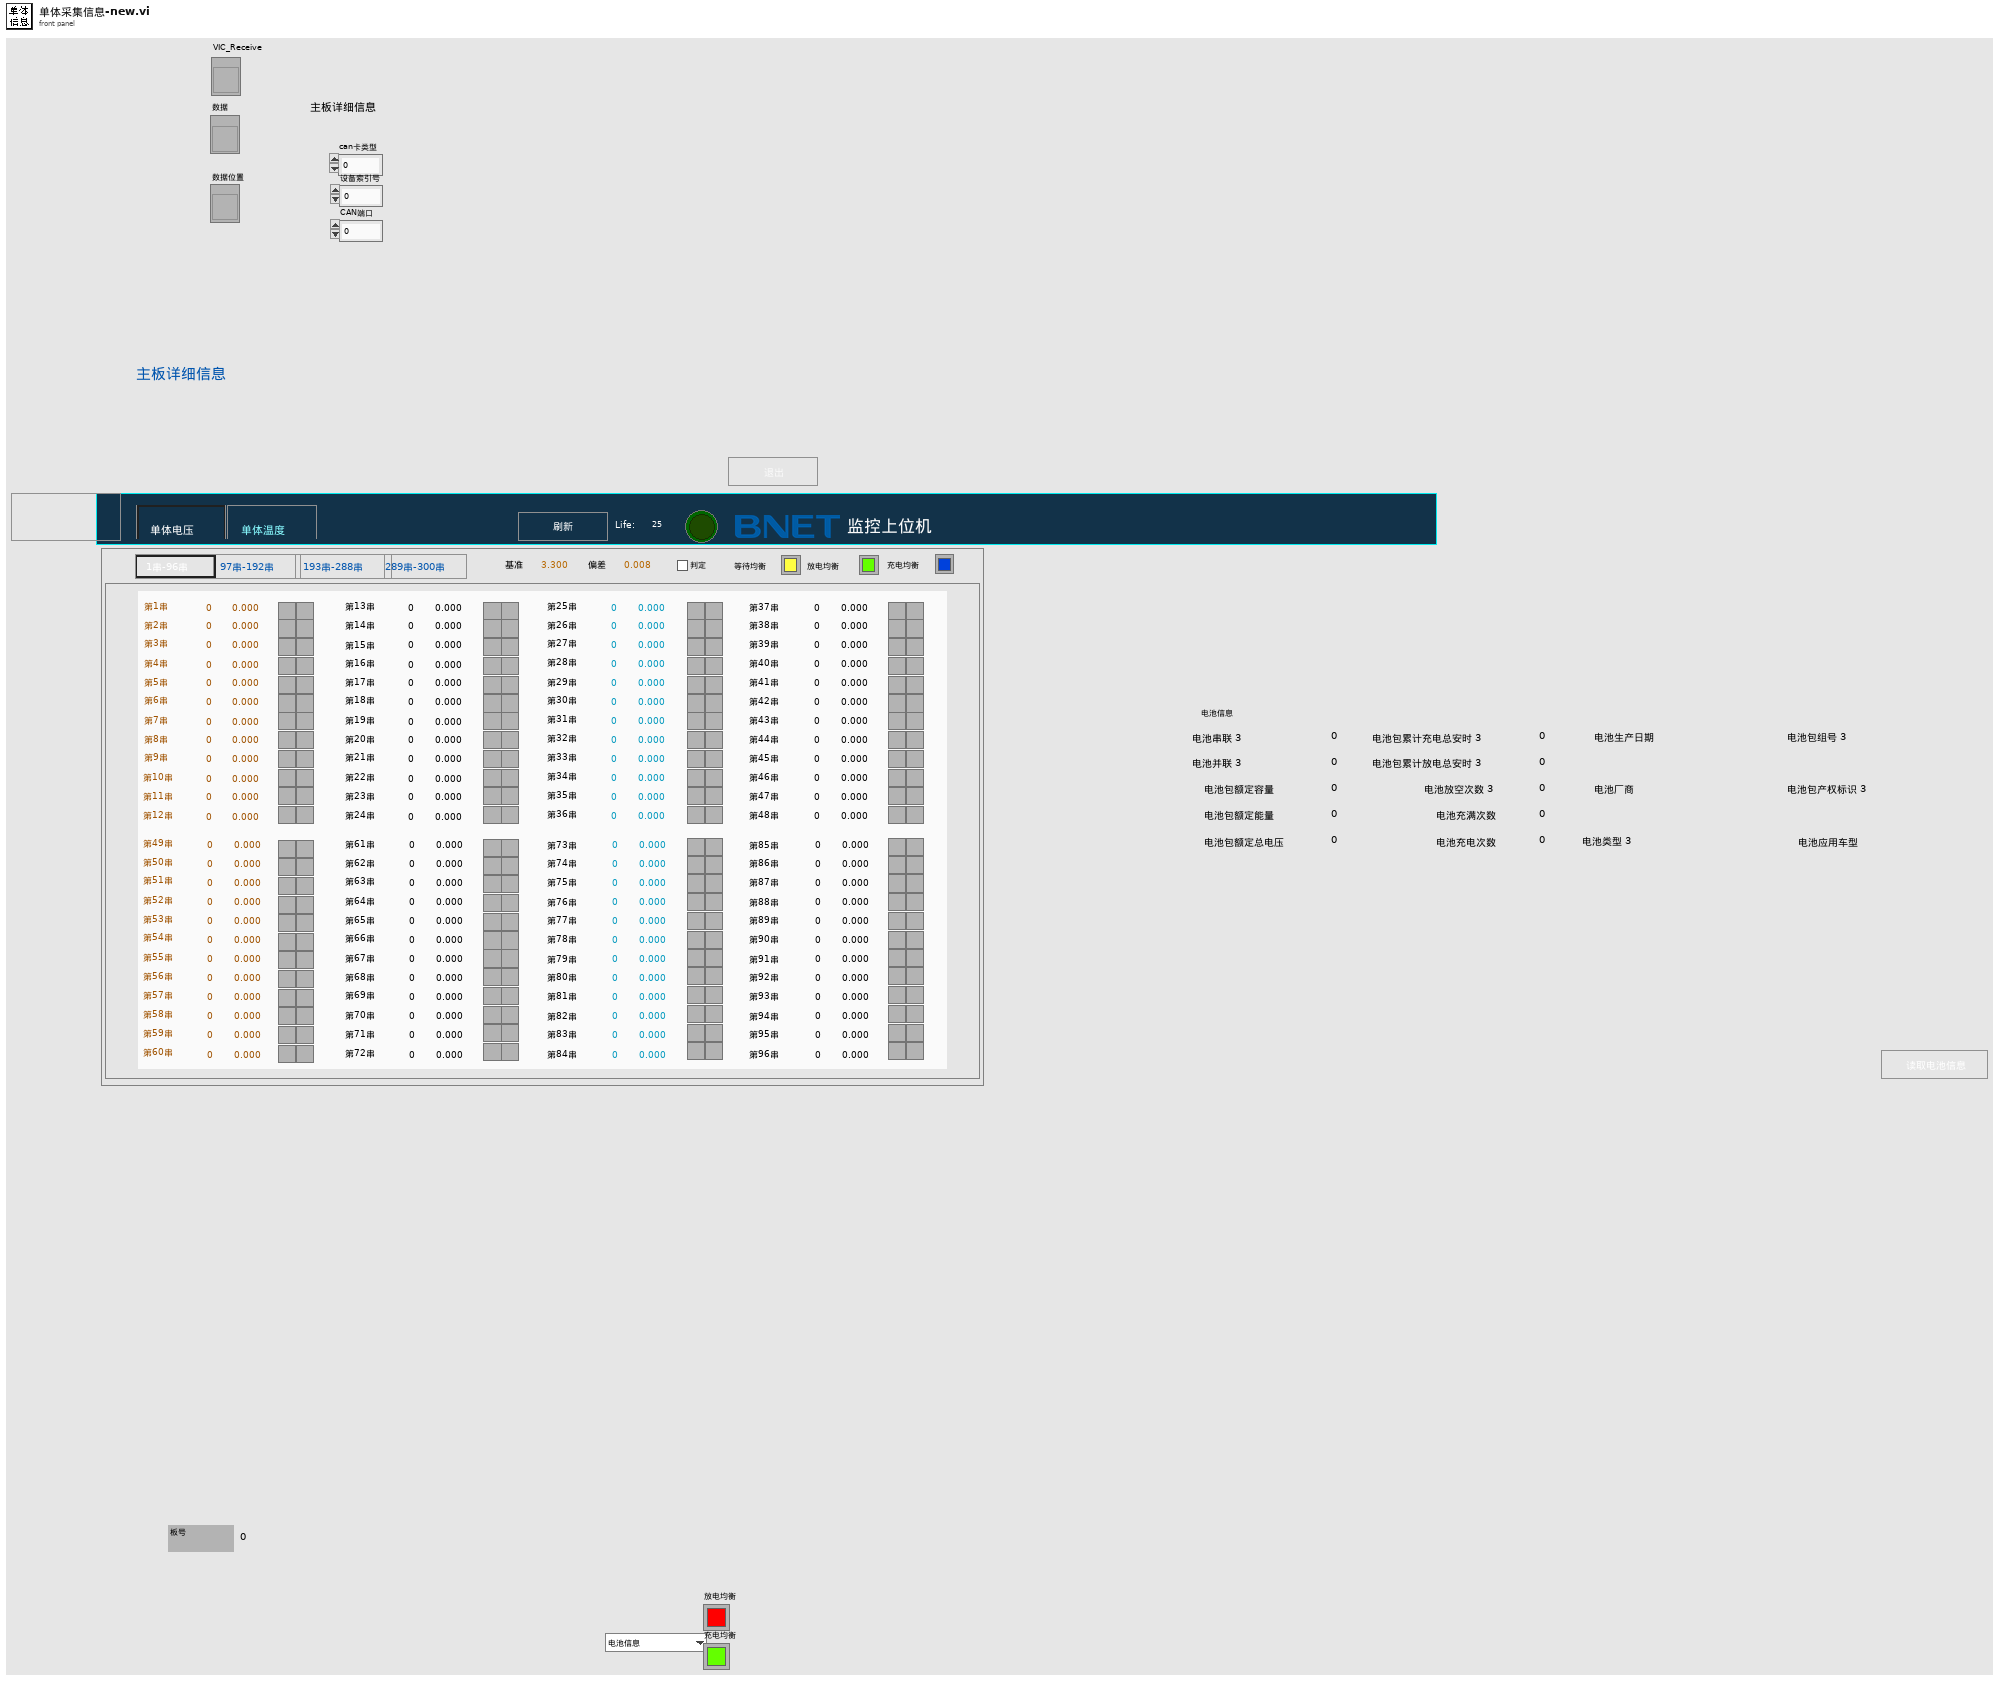
[diagram p1: front panel]
types:
  T1 = cluster{"ID":u32, "TimeStamp":u32, "TimeFlag":u8, "SendType":u8, "RemoteFlag":u8, "ExternFlag":u8, "DataLen":u8, "Data1":u8, "Data2":u8, "Data3":u8, "Data4":u8, "Data5":u8, "Data6":u8, "Data7":u8, "Data8":u8, "Rsv1":u8, "Rsv2":u8, "Rsv3":u8}
  T2 = cluster{"电池串联 3":dbl, "电池并联 3":dbl, "电池包累计放电总安时 3":dbl, "电池包额定容量":dbl, "电池包额定能量":dbl, "电池包额定总电压":dbl, "电池包累计充电总安时 3":dbl, "电池充满次数":dbl, "电池放空次数 3":dbl, "电池充电次数":dbl, "电池生产日期":string, "电池厂商":string, "电池类型 3":string, "电池包组号 3":string, "电池包产权标识 3":string, "电池应用车型":string}
  T3 = enum32{"单选选项2 5", "单选选项2 6", "单选选项2 7", "单选选项2 8"}
  T4 = cluster{"1 102":cluster{"第1串":dbl, "第2串":dbl, "第3串":dbl, "第4串":dbl, "第5串":dbl, "第6串":dbl, "第7串":dbl, "第8串":dbl, "第9串":dbl, "第10串":dbl, "第11串":dbl, "第12串":dbl, "第一串 2":dbl, "第一串 4":dbl, "第一串 6":dbl, "第一串 8":dbl, "第一串 10":dbl, "第一串 12":dbl, "第一串 14":dbl, "第一串 16":dbl, "第一串 18":dbl, "第一串 20":dbl, "第一串 22":dbl, "第一串 24":dbl}, "1 3":cluster{"第13串":dbl, "第14串":dbl, "第15串":dbl, "第16串":dbl, "第17串":dbl, "第18串":dbl, "第19串":dbl, "第20串":dbl, "第21串":dbl, "第22串":dbl, "第23串":dbl, "第24串":dbl, "第一串 2":dbl, "第一串 4":dbl, "第一串 6":dbl, "第一串 8":dbl, "第一串 10":dbl, "第一串 12":dbl, "第一串 14":dbl, "第一串 16":dbl, "第一串 18":dbl, "第一串 20":dbl, "第一串 22":dbl, "第一串 24":dbl}, "1 4":cluster{"第25串":dbl, "第26串":dbl, "第27串":dbl, "第28串":dbl, "第29串":dbl, "第30串":dbl, "第31串":dbl, "第32串":dbl, "第33串":dbl, "第34串":dbl, "第35串":dbl, "第36串":dbl, "第一串 2":dbl, "第一串 4":dbl, "第一串 6":dbl, "第一串 8":dbl, "第一串 10":dbl, "第一串 12":dbl, "第一串 14":dbl, "第一串 16":dbl, "第一串 18":dbl, "第一串 20":dbl, "第一串 22":dbl, "第一串 24":dbl}, "1 6":cluster{"第37串":dbl, "第38串":dbl, "第39串":dbl, "第40串":dbl, "第41串":dbl, "第42串":dbl, "第43串":dbl, "第44串":dbl, "第45串":dbl, "第46串":dbl, "第47串":dbl, "第48串":dbl, "第一串 2":dbl, "第一串 4":dbl, "第一串 6":dbl, "第一串 8":dbl, "第一串 10":dbl, "第一串 12":dbl, "第一串 14":dbl, "第一串 16":dbl, "第一串 18":dbl, "第一串 20":dbl, "第一串 22":dbl, "第一串 24":dbl}, "1 7":cluster{"第49串":dbl, "第50串":dbl, "第51串":dbl, "第52串":dbl, "第53串":dbl, "第54串":dbl, "第55串":dbl, "第56串":dbl, "第57串":dbl, "第58串":dbl, "第59串":dbl, "第60串":dbl, "第一串 2":dbl, "第一串 4":dbl, "第一串 6":dbl, "第一串 8":dbl, "第一串 10":dbl, "第一串 12":dbl, "第一串 14":dbl, "第一串 16":dbl, "第一串 18":dbl, "第一串 20":dbl, "第一串 22":dbl, "第一串 24":dbl}, "1 8":cluster{"第61串":dbl, "第62串":dbl, "第63串":dbl, "第64串":dbl, "第65串":dbl, "第66串":dbl, "第67串":dbl, "第68串":dbl, "第69串":dbl, "第70串":dbl, "第71串":dbl, "第72串":dbl, "第一串 2":dbl, "第一串 4":dbl, "第一串 6":dbl, "第一串 8":dbl, "第一串 10":dbl, "第一串 12":dbl, "第一串 14":dbl, "第一串 16":dbl, "第一串 18":dbl, "第一串 20":dbl, "第一串 22":dbl, "第一串 24":dbl}, "1 9":cluster{"第73串":dbl, "第74串":dbl, "第75串":dbl, "第76串":dbl, "第77串":dbl, "第78串":dbl, "第79串":dbl, "第80串":dbl, "第81串":dbl, "第82串":dbl, "第83串":dbl, "第84串":dbl, "第一串 2":dbl, "第一串 4":dbl, "第一串 6":dbl, "第一串 8":dbl, "第一串 10":dbl, "第一串 12":dbl, "第一串 14":dbl, "第一串 16":dbl, "第一串 18":dbl, "第一串 20":dbl, "第一串 22":dbl, "第一串 24":dbl}, "1 10":cluster{"第85串":dbl, "第86串":dbl, "第87串":dbl, "第88串":dbl, "第89串":dbl, "第90串":dbl, "第91串":dbl, "第92串":dbl, "第93串":dbl, "第94串":dbl, "第95串":dbl, "第96串":dbl, "第一串 2":dbl, "第一串 4":dbl, "第一串 6":dbl, "第一串 8":dbl, "第一串 10":dbl, "第一串 12":dbl, "第一串 14":dbl, "第一串 16":dbl, "第一串 18":dbl, "第一串 20":dbl, "第一串 22":dbl, "第一串 24":dbl}, "1 12":cluster{"充电1":u32, "充电1":u32, "充电1":u32, "充电1":u32, "充电1":u32, "充电1":u32, "充电1":u32, "充电1":u32, "充电1":u32, "充电1":u32, "充电1":u32, "充电1":u32}, "1 28":cluster{"充电1":u32, "充电1":u32, "充电1":u32, "充电1":u32, "充电1":u32, "充电1":u32, "充电1":u32, "充电1":u32, "充电1":u32, "充电1":u32, "充电1":u32, "充电1":u32}, "1 25":cluster{"充电1":u32, "充电1":u32, "充电1":u32, "充电1":u32, "充电1":u32, "充电1":u32, "充电1":u32, "充电1":u32, "充电1":u32, "充电1":u32, "充电1":u32, "充电1":u32}, "1 31":cluster{"充电1":u32, "充电1":u32, "充电1":u32, "充电1":u32, "充电1":u32, "充电1":u32, "充电1":u32, "充电1":u32, "充电1":u32, "充电1":u32, "充电1":u32, "充电1":u32}, "1 16":cluster{"充电1":u32, "充电1":u32, "充电1":u32, "充电1":u32, "充电1":u32, "充电1":u32, "充电1":u32, "充电1":u32, "充电1":u32, "充电1":u32, "充电1":u32, "充电1":u32}, "1 19":cluster{"充电1":u32, "充电1":u32, "充电1":u32, "充电1":u32, "充电1":u32, "充电1":u32, "充电1":u32, "充电1":u32, "充电1":u32, "充电1":u32, "充电1":u32, "充电1":u32}, "1 22":cluster{"充电1":u32, "充电1":u32, "充电1":u32, "充电1":u32, "充电1":u32, "充电1":u32, "充电1":u32, "充电1":u32, "充电1":u32, "充电1":u32, "充电1":u32, "充电1":u32}, "1 34":cluster{"充电1":u32, "充电1":u32, "充电1":u32, "充电1":u32, "充电1":u32, "充电1":u32, "充电1":u32, "充电1":u32, "充电1":u32, "充电1":u32, "充电1":u32, "充电1":u32}, "1 11":cluster{"充电1":u32, "充电1":u32, "充电1":u32, "充电1":u32, "充电1":u32, "充电1":u32, "充电1":u32, "充电1":u32, "充电1":u32, "充电1":u32, "充电1":u32, "充电1":u32}, "1 27":cluster{"充电1":u32, "充电1":u32, "充电1":u32, "充电1":u32, "充电1":u32, "充电1":u32, "充电1":u32, "充电1":u32, "充电1":u32, "充电1":u32, "充电1":u32, "充电1":u32}, "1 24":cluster{"充电1":u32, "充电1":u32, "充电1":u32, "充电1":u32, "充电1":u32, "充电1":u32, "充电1":u32, "充电1":u32, "充电1":u32, "充电1":u32, "充电1":u32, "充电1":u32}, "1 30":cluster{"充电1":u32, "充电1":u32, "充电1":u32, "充电1":u32, "充电1":u32, "充电1":u32, "充电1":u32, "充电1":u32, "充电1":u32, "充电1":u32, "充电1":u32, "充电1":u32}, "1 15":cluster{"充电1":u32, "充电1":u32, "充电1":u32, "充电1":u32, "充电1":u32, "充电1":u32, "充电1":u32, "充电1":u32, "充电1":u32, "充电1":u32, "充电1":u32, "充电1":u32}, "1 18":cluster{"充电1":u32, "充电1":u32, "充电1":u32, "充电1":u32, "充电1":u32, "充电1":u32, "充电1":u32, "充电1":u32, "充电1":u32, "充电1":u32, "充电1":u32, "充电1":u32}, "1 21":cluster{"充电1":u32, "充电1":u32, "充电1":u32, "充电1":u32, "充电1":u32, "充电1":u32, "充电1":u32, "充电1":u32, "充电1":u32, "充电1":u32, "充电1":u32, "充电1":u32}, "1 33":cluster{"充电1":u32, "充电1":u32, "充电1":u32, "充电1":u32, "充电1":u32, "充电1":u32, "充电1":u32, "充电1":u32, "充电1":u32, "充电1":u32, "充电1":u32, "充电1":u32}, "1 13":cluster{"均衡故障":i32, "均衡故障 2":dbl, "均衡故障 3":dbl, "均衡故障 4":dbl, "均衡故障 5":dbl, "均衡故障 6":dbl, "均衡故障 7":dbl, "均衡故障 8":dbl, "均衡故障 9":dbl, "均衡故障 10":dbl, "均衡故障 11":dbl, "均衡故障 12":dbl}, "1 26":cluster{"均衡故障":i32, "均衡故障 2":dbl, "均衡故障 3":dbl, "均衡故障 4":dbl, "均衡故障 5":dbl, "均衡故障 6":dbl, "均衡故障 7":dbl, "均衡故障 8":dbl, "均衡故障 9":dbl, "均衡故障 10":dbl, "均衡故障 11":dbl, "均衡故障 12":dbl}, "1 23":cluster{"均衡故障":i32, "均衡故障 2":dbl, "均衡故障 3":dbl, "均衡故障 4":dbl, "均衡故障 5":dbl, "均衡故障 6":dbl, "均衡故障 7":dbl, "均衡故障 8":dbl, "均衡故障 9":dbl, "均衡故障 10":dbl, "均衡故障 11":dbl, "均衡故障 12":dbl}, "1 29":cluster{"均衡故障":i32, "均衡故障 2":dbl, "均衡故障 3":dbl, "均衡故障 4":dbl, "均衡故障 5":dbl, "均衡故障 6":dbl, "均衡故障 7":dbl, "均衡故障 8":dbl, "均衡故障 9":dbl, "均衡故障 10":dbl, "均衡故障 11":dbl, "均衡故障 12":dbl}, "1 14":cluster{"均衡故障":i32, "均衡故障 2":dbl, "均衡故障 3":dbl, "均衡故障 4":dbl, "均衡故障 5":dbl, "均衡故障 6":dbl, "均衡故障 7":dbl, "均衡故障 8":dbl, "均衡故障 9":dbl, "均衡故障 10":dbl, "均衡故障 11":dbl, "均衡故障 12":dbl}, "1 17":cluster{"均衡故障":i32, "均衡故障 2":dbl, "均衡故障 3":dbl, "均衡故障 4":dbl, "均衡故障 5":dbl, "均衡故障 6":dbl, "均衡故障 7":dbl, "均衡故障 8":dbl, "均衡故障 9":dbl, "均衡故障 10":dbl, "均衡故障 11":dbl, "均衡故障 12":dbl}, "1 20":cluster{"均衡故障":i32, "均衡故障 2":dbl, "均衡故障 3":dbl, "均衡故障 4":dbl, "均衡故障 5":dbl, "均衡故障 6":dbl, "均衡故障 7":dbl, "均衡故障 8":dbl, "均衡故障 9":dbl, "均衡故障 10":dbl, "均衡故障 11":dbl, "均衡故障 12":dbl}, "1 32":cluster{"均衡故障":i32, "均衡故障 2":dbl, "均衡故障 3":dbl, "均衡故障 4":dbl, "均衡故障 5":dbl, "均衡故障 6":dbl, "均衡故障 7":dbl, "均衡故障 8":dbl, "均衡故障 9":dbl, "均衡故障 10":dbl, "均衡故障 11":dbl, "均衡故障 12":dbl}}
  T5 = cluster{"1 26":cluster{"第97串":dbl, "第98串":dbl, "第99串":dbl, "第100串":dbl, "第101串":dbl, "第102串":dbl, "第103串":dbl, "第104串":dbl, "第105串":dbl, "第106串":dbl, "第107串":dbl, "第108串":dbl, "第一串 2":dbl, "第一串 4":dbl, "第一串 6":dbl, "第一串 8":dbl, "第一串 10":dbl, "第一串 12":dbl, "第一串 14":dbl, "第一串 16":dbl, "第一串 18":dbl, "第一串 20":dbl, "第一串 22":dbl, "第一串 24":dbl}, "1 27":cluster{"第109串":dbl, "第110串":dbl, "第111串":dbl, "第112串":dbl, "第113串":dbl, "第114串":dbl, "第115串":dbl, "第116串":dbl, "第117串":dbl, "第118串":dbl, "第119串":dbl, "第120串":dbl, "第一串 2":dbl, "第一串 4":dbl, "第一串 6":dbl, "第一串 8":dbl, "第一串 10":dbl, "第一串 12":dbl, "第一串 14":dbl, "第一串 16":dbl, "第一串 18":dbl, "第一串 20":dbl, "第一串 22":dbl, "第一串 24":dbl}, "1 28":cluster{"第121串":dbl, "第122串":dbl, "第123串":dbl, "第124串":dbl, "第125串":dbl, "第126串":dbl, "第127串":dbl, "第128串":dbl, "第129串":dbl, "第130串":dbl, "第131串":dbl, "第132串":dbl, "第一串 2":dbl, "第一串 4":dbl, "第一串 6":dbl, "第一串 8":dbl, "第一串 10":dbl, "第一串 12":dbl, "第一串 14":dbl, "第一串 16":dbl, "第一串 18":dbl, "第一串 20":dbl, "第一串 22":dbl, "第一串 24":dbl}, "1 29":cluster{"第133串":dbl, "第134串":dbl, "第135串":dbl, "第136串":dbl, "第137串":dbl, "第138串":dbl, "第139串":dbl, "第140串":dbl, "第141串":dbl, "第142串":dbl, "第143串":dbl, "第144串":dbl, "第一串 2":dbl, "第一串 4":dbl, "第一串 6":dbl, "第一串 8":dbl, "第一串 10":dbl, "第一串 12":dbl, "第一串 14":dbl, "第一串 16":dbl, "第一串 18":dbl, "第一串 20":dbl, "第一串 22":dbl, "第一串 24":dbl}, "1 30":cluster{"第145串":dbl, "第146串":dbl, "第147串":dbl, "第148串":dbl, "第149串":dbl, "第150串":dbl, "第151串":dbl, "第152串":dbl, "第153串":dbl, "第154串":dbl, "第155串":dbl, "第156串":dbl, "第一串 2":dbl, "第一串 4":dbl, "第一串 6":dbl, "第一串 8":dbl, "第一串 10":dbl, "第一串 12":dbl, "第一串 14":dbl, "第一串 16":dbl, "第一串 18":dbl, "第一串 20":dbl, "第一串 22":dbl, "第一串 24":dbl}, "1 31":cluster{"第157串":dbl, "第158串":dbl, "第159串":dbl, "第160串":dbl, "第161串":dbl, "第162串":dbl, "第163串":dbl, "第164串":dbl, "第165串":dbl, "第166串":dbl, "第167串":dbl, "第168串":dbl, "第一串 2":dbl, "第一串 4":dbl, "第一串 6":dbl, "第一串 8":dbl, "第一串 10":dbl, "第一串 12":dbl, "第一串 14":dbl, "第一串 16":dbl, "第一串 18":dbl, "第一串 20":dbl, "第一串 22":dbl, "第一串 24":dbl}, "1 32":cluster{"第169串":dbl, "第170串":dbl, "第171串":dbl, "第172串":dbl, "第173串":dbl, "第174串":dbl, "第175串":dbl, "第176串":dbl, "第177串":dbl, "第178串":dbl, "第179串":dbl, "第180串":dbl, "第一串 2":dbl, "第一串 4":dbl, "第一串 6":dbl, "第一串 8":dbl, "第一串 10":dbl, "第一串 12":dbl, "第一串 14":dbl, "第一串 16":dbl, "第一串 18":dbl, "第一串 20":dbl, "第一串 22":dbl, "第一串 24":dbl}, "1 33":cluster{"第181串":dbl, "第182串":dbl, "第183串":dbl, "第184串":dbl, "第185串":dbl, "第186串":dbl, "第187串":dbl, "第188串":dbl, "第189串":dbl, "第190串":dbl, "第191串":dbl, "第192串":dbl, "第一串 2":dbl, "第一串 4":dbl, "第一串 6":dbl, "第一串 8":dbl, "第一串 10":dbl, "第一串 12":dbl, "第一串 14":dbl, "第一串 16":dbl, "第一串 18":dbl, "第一串 20":dbl, "第一串 22":dbl, "第一串 24":dbl}, "1 16":cluster{"充电1":u32, "充电1":u32, "充电1":u32, "充电1":u32, "充电1":u32, "充电1":u32, "充电1":u32, "充电1":u32, "充电1":u32, "充电1":u32, "充电1":u32, "充电1":u32}, "1 44":cluster{"充电1":u32, "充电1":u32, "充电1":u32, "充电1":u32, "充电1":u32, "充电1":u32, "充电1":u32, "充电1":u32, "充电1":u32, "充电1":u32, "充电1":u32, "充电1":u32}, "1 36":cluster{"充电1":u32, "充电1":u32, "充电1":u32, "充电1":u32, "充电1":u32, "充电1":u32, "充电1":u32, "充电1":u32, "充电1":u32, "充电1":u32, "充电1":u32, "充电1":u32}, "1 47":cluster{"充电1":u32, "充电1":u32, "充电1":u32, "充电1":u32, "充电1":u32, "充电1":u32, "充电1":u32, "充电1":u32, "充电1":u32, "充电1":u32, "充电1":u32, "充电1":u32}, "1 19":cluster{"充电1":u32, "充电1":u32, "充电1":u32, "充电1":u32, "充电1":u32, "充电1":u32, "充电1":u32, "充电1":u32, "充电1":u32, "充电1":u32, "充电1":u32, "充电1":u32}, "1 38":cluster{"充电1":u32, "充电1":u32, "充电1":u32, "充电1":u32, "充电1":u32, "充电1":u32, "充电1":u32, "充电1":u32, "充电1":u32, "充电1":u32, "充电1":u32, "充电1":u32}, "1 41":cluster{"充电1":u32, "充电1":u32, "充电1":u32, "充电1":u32, "充电1":u32, "充电1":u32, "充电1":u32, "充电1":u32, "充电1":u32, "充电1":u32, "充电1":u32, "充电1":u32}, "1 50":cluster{"充电1":u32, "充电1":u32, "充电1":u32, "充电1":u32, "充电1":u32, "充电1":u32, "充电1":u32, "充电1":u32, "充电1":u32, "充电1":u32, "充电1":u32, "充电1":u32}, "1 15":cluster{"充电1":u32, "充电1":u32, "充电1":u32, "充电1":u32, "充电1":u32, "充电1":u32, "充电1":u32, "充电1":u32, "充电1":u32, "充电1":u32, "充电1":u32, "充电1":u32}, "1 43":cluster{"充电1":u32, "充电1":u32, "充电1":u32, "充电1":u32, "充电1":u32, "充电1":u32, "充电1":u32, "充电1":u32, "充电1":u32, "充电1":u32, "充电1":u32, "充电1":u32}, "1 35":cluster{"充电1":u32, "充电1":u32, "充电1":u32, "充电1":u32, "充电1":u32, "充电1":u32, "充电1":u32, "充电1":u32, "充电1":u32, "充电1":u32, "充电1":u32, "充电1":u32}, "1 46":cluster{"充电1":u32, "充电1":u32, "充电1":u32, "充电1":u32, "充电1":u32, "充电1":u32, "充电1":u32, "充电1":u32, "充电1":u32, "充电1":u32, "充电1":u32, "充电1":u32}, "1 18":cluster{"充电1":u32, "充电1":u32, "充电1":u32, "充电1":u32, "充电1":u32, "充电1":u32, "充电1":u32, "充电1":u32, "充电1":u32, "充电1":u32, "充电1":u32, "充电1":u32}, "1 37":cluster{"充电1":u32, "充电1":u32, "充电1":u32, "充电1":u32, "充电1":u32, "充电1":u32, "充电1":u32, "充电1":u32, "充电1":u32, "充电1":u32, "充电1":u32, "充电1":u32}, "1 40":cluster{"充电1":u32, "充电1":u32, "充电1":u32, "充电1":u32, "充电1":u32, "充电1":u32, "充电1":u32, "充电1":u32, "充电1":u32, "充电1":u32, "充电1":u32, "充电1":u32}, "1 49":cluster{"充电1":u32, "充电1":u32, "充电1":u32, "充电1":u32, "充电1":u32, "充电1":u32, "充电1":u32, "充电1":u32, "充电1":u32, "充电1":u32, "充电1":u32, "充电1":u32}, "1 14":cluster{"均衡故障":i32, "均衡故障 2":dbl, "均衡故障 3":dbl, "均衡故障 4":dbl, "均衡故障 5":dbl, "均衡故障 6":dbl, "均衡故障 7":dbl, "均衡故障 8":dbl, "均衡故障 9":dbl, "均衡故障 10":dbl, "均衡故障 11":dbl, "均衡故障 12":dbl}, "1 42":cluster{"均衡故障":i32, "均衡故障 2":dbl, "均衡故障 3":dbl, "均衡故障 4":dbl, "均衡故障 5":dbl, "均衡故障 6":dbl, "均衡故障 7":dbl, "均衡故障 8":dbl, "均衡故障 9":dbl, "均衡故障 10":dbl, "均衡故障 11":dbl, "均衡故障 12":dbl}, "1 34":cluster{"均衡故障":i32, "均衡故障 2":dbl, "均衡故障 3":dbl, "均衡故障 4":dbl, "均衡故障 5":dbl, "均衡故障 6":dbl, "均衡故障 7":dbl, "均衡故障 8":dbl, "均衡故障 9":dbl, "均衡故障 10":dbl, "均衡故障 11":dbl, "均衡故障 12":dbl}, "1 45":cluster{"均衡故障":i32, "均衡故障 2":dbl, "均衡故障 3":dbl, "均衡故障 4":dbl, "均衡故障 5":dbl, "均衡故障 6":dbl, "均衡故障 7":dbl, "均衡故障 8":dbl, "均衡故障 9":dbl, "均衡故障 10":dbl, "均衡故障 11":dbl, "均衡故障 12":dbl}, "1 17":cluster{"均衡故障":i32, "均衡故障 2":dbl, "均衡故障 3":dbl, "均衡故障 4":dbl, "均衡故障 5":dbl, "均衡故障 6":dbl, "均衡故障 7":dbl, "均衡故障 8":dbl, "均衡故障 9":dbl, "均衡故障 10":dbl, "均衡故障 11":dbl, "均衡故障 12":dbl}, "1 20":cluster{"均衡故障":i32, "均衡故障 2":dbl, "均衡故障 3":dbl, "均衡故障 4":dbl, "均衡故障 5":dbl, "均衡故障 6":dbl, "均衡故障 7":dbl, "均衡故障 8":dbl, "均衡故障 9":dbl, "均衡故障 10":dbl, "均衡故障 11":dbl, "均衡故障 12":dbl}, "1 39":cluster{"均衡故障":i32, "均衡故障 2":dbl, "均衡故障 3":dbl, "均衡故障 4":dbl, "均衡故障 5":dbl, "均衡故障 6":dbl, "均衡故障 7":dbl, "均衡故障 8":dbl, "均衡故障 9":dbl, "均衡故障 10":dbl, "均衡故障 11":dbl, "均衡故障 12":dbl}, "1 48":cluster{"均衡故障":i32, "均衡故障 2":dbl, "均衡故障 3":dbl, "均衡故障 4":dbl, "均衡故障 5":dbl, "均衡故障 6":dbl, "均衡故障 7":dbl, "均衡故障 8":dbl, "均衡故障 9":dbl, "均衡故障 10":dbl, "均衡故障 11":dbl, "均衡故障 12":dbl}}
  T6 = cluster{"1 18":cluster{"第193串":dbl, "第194串":dbl, "第195串":dbl, "第196串":dbl, "第197串":dbl, "第198串":dbl, "第199串":dbl, "第200串":dbl, "第201串":dbl, "第202串":dbl, "第203串":dbl, "第204串":dbl, "第一串 2":dbl, "第一串 4":dbl, "第一串 6":dbl, "第一串 8":dbl, "第一串 10":dbl, "第一串 12":dbl, "第一串 14":dbl, "第一串 16":dbl, "第一串 18":dbl, "第一串 20":dbl, "第一串 22":dbl, "第一串 24":dbl}, "1 19":cluster{"第205串":dbl, "第206串":dbl, "第207串":dbl, "第208串":dbl, "第209串":dbl, "第210串":dbl, "第211串":dbl, "第212串":dbl, "第213串":dbl, "第214串":dbl, "第215串":dbl, "第216串":dbl, "第一串 2":dbl, "第一串 4":dbl, "第一串 6":dbl, "第一串 8":dbl, "第一串 10":dbl, "第一串 12":dbl, "第一串 14":dbl, "第一串 16":dbl, "第一串 18":dbl, "第一串 20":dbl, "第一串 22":dbl, "第一串 24":dbl}, "1 20":cluster{"第217串":dbl, "第218串":dbl, "第219串":dbl, "第220串":dbl, "第221串":dbl, "第222串":dbl, "第223串":dbl, "第224串":dbl, "第225串":dbl, "第226串":dbl, "第227串":dbl, "第228串":dbl, "第一串 2":dbl, "第一串 4":dbl, "第一串 6":dbl, "第一串 8":dbl, "第一串 10":dbl, "第一串 12":dbl, "第一串 14":dbl, "第一串 16":dbl, "第一串 18":dbl, "第一串 20":dbl, "第一串 22":dbl, "第一串 24":dbl}, "1 21":cluster{"第229串":dbl, "第230串":dbl, "第231串":dbl, "第232串":dbl, "第233串":dbl, "第234串":dbl, "第235串":dbl, "第236串":dbl, "第237串":dbl, "第238串":dbl, "第239串":dbl, "第240串":dbl, "第一串 2":dbl, "第一串 4":dbl, "第一串 6":dbl, "第一串 8":dbl, "第一串 10":dbl, "第一串 12":dbl, "第一串 14":dbl, "第一串 16":dbl, "第一串 18":dbl, "第一串 20":dbl, "第一串 22":dbl, "第一串 24":dbl}, "1 22":cluster{"第241串":dbl, "第242串":dbl, "第243串":dbl, "第244串":dbl, "第245串":dbl, "第246串":dbl, "第247串":dbl, "第248串":dbl, "第249串":dbl, "第250串":dbl, "第251串":dbl, "第252串":dbl, "第一串 2":dbl, "第一串 4":dbl, "第一串 6":dbl, "第一串 8":dbl, "第一串 10":dbl, "第一串 12":dbl, "第一串 14":dbl, "第一串 16":dbl, "第一串 18":dbl, "第一串 20":dbl, "第一串 22":dbl, "第一串 24":dbl}, "1 23":cluster{"第253串":dbl, "第254串":dbl, "第255串":dbl, "第256串":dbl, "第257串":dbl, "第258串":dbl, "第259串":dbl, "第260串":dbl, "第261串":dbl, "第262串":dbl, "第263串":dbl, "第264串":dbl, "第一串 2":dbl, "第一串 4":dbl, "第一串 6":dbl, "第一串 8":dbl, "第一串 10":dbl, "第一串 12":dbl, "第一串 14":dbl, "第一串 16":dbl, "第一串 18":dbl, "第一串 20":dbl, "第一串 22":dbl, "第一串 24":dbl}, "1 24":cluster{"第265串":dbl, "第266串":dbl, "第267串":dbl, "第268串":dbl, "第269串":dbl, "第270串":dbl, "第271串":dbl, "第272串":dbl, "第273串":dbl, "第274串":dbl, "第275串":dbl, "第276串":dbl, "第一串 2":dbl, "第一串 4":dbl, "第一串 6":dbl, "第一串 8":dbl, "第一串 10":dbl, "第一串 12":dbl, "第一串 14":dbl, "第一串 16":dbl, "第一串 18":dbl, "第一串 20":dbl, "第一串 22":dbl, "第一串 24":dbl}, "1 25":cluster{"第277串":dbl, "第278串":dbl, "第279串":dbl, "第280串":dbl, "第281串":dbl, "第282串":dbl, "第283串":dbl, "第284串":dbl, "第285串":dbl, "第286串":dbl, "第287串":dbl, "第288串":dbl, "第一串 2":dbl, "第一串 4":dbl, "第一串 6":dbl, "第一串 8":dbl, "第一串 10":dbl, "第一串 12":dbl, "第一串 14":dbl, "第一串 16":dbl, "第一串 18":dbl, "第一串 20":dbl, "第一串 22":dbl, "第一串 24":dbl}, "1 12":cluster{"充电1":u32, "充电1":u32, "充电1":u32, "充电1":u32, "充电1":u32, "充电1":u32, "充电1":u32, "充电1":u32, "充电1":u32, "充电1":u32, "充电1":u32, "充电1":u32}, "1 39":cluster{"充电1":u32, "充电1":u32, "充电1":u32, "充电1":u32, "充电1":u32, "充电1":u32, "充电1":u32, "充电1":u32, "充电1":u32, "充电1":u32, "充电1":u32, "充电1":u32}, "1 28":cluster{"充电1":u32, "充电1":u32, "充电1":u32, "充电1":u32, "充电1":u32, "充电1":u32, "充电1":u32, "充电1":u32, "充电1":u32, "充电1":u32, "充电1":u32, "充电1":u32}, "1 42":cluster{"充电1":u32, "充电1":u32, "充电1":u32, "充电1":u32, "充电1":u32, "充电1":u32, "充电1":u32, "充电1":u32, "充电1":u32, "充电1":u32, "充电1":u32, "充电1":u32}, "1 16":cluster{"充电1":u32, "充电1":u32, "充电1":u32, "充电1":u32, "充电1":u32, "充电1":u32, "充电1":u32, "充电1":u32, "充电1":u32, "充电1":u32, "充电1":u32, "充电1":u32}, "1 30":cluster{"充电1":u32, "充电1":u32, "充电1":u32, "充电1":u32, "充电1":u32, "充电1":u32, "充电1":u32, "充电1":u32, "充电1":u32, "充电1":u32, "充电1":u32, "充电1":u32}, "1 33":cluster{"充电1":u32, "充电1":u32, "充电1":u32, "充电1":u32, "充电1":u32, "充电1":u32, "充电1":u32, "充电1":u32, "充电1":u32, "充电1":u32, "充电1":u32, "充电1":u32}, "1 36":cluster{"充电1":u32, "充电1":u32, "充电1":u32, "充电1":u32, "充电1":u32, "充电1":u32, "充电1":u32, "充电1":u32, "充电1":u32, "充电1":u32, "充电1":u32, "充电1":u32}, "1 11":cluster{"充电1":u32, "充电1":u32, "充电1":u32, "充电1":u32, "充电1":u32, "充电1":u32, "充电1":u32, "充电1":u32, "充电1":u32, "充电1":u32, "充电1":u32, "充电1":u32}, "1 38":cluster{"充电1":u32, "充电1":u32, "充电1":u32, "充电1":u32, "充电1":u32, "充电1":u32, "充电1":u32, "充电1":u32, "充电1":u32, "充电1":u32, "充电1":u32, "充电1":u32}, "1 27":cluster{"充电1":u32, "充电1":u32, "充电1":u32, "充电1":u32, "充电1":u32, "充电1":u32, "充电1":u32, "充电1":u32, "充电1":u32, "充电1":u32, "充电1":u32, "充电1":u32}, "1 41":cluster{"充电1":u32, "充电1":u32, "充电1":u32, "充电1":u32, "充电1":u32, "充电1":u32, "充电1":u32, "充电1":u32, "充电1":u32, "充电1":u32, "充电1":u32, "充电1":u32}, "1 15":cluster{"充电1":u32, "充电1":u32, "充电1":u32, "充电1":u32, "充电1":u32, "充电1":u32, "充电1":u32, "充电1":u32, "充电1":u32, "充电1":u32, "充电1":u32, "充电1":u32}, "1 29":cluster{"充电1":u32, "充电1":u32, "充电1":u32, "充电1":u32, "充电1":u32, "充电1":u32, "充电1":u32, "充电1":u32, "充电1":u32, "充电1":u32, "充电1":u32, "充电1":u32}, "1 32":cluster{"充电1":u32, "充电1":u32, "充电1":u32, "充电1":u32, "充电1":u32, "充电1":u32, "充电1":u32, "充电1":u32, "充电1":u32, "充电1":u32, "充电1":u32, "充电1":u32}, "1 35":cluster{"充电1":u32, "充电1":u32, "充电1":u32, "充电1":u32, "充电1":u32, "充电1":u32, "充电1":u32, "充电1":u32, "充电1":u32, "充电1":u32, "充电1":u32, "充电1":u32}, "1 13":cluster{"均衡故障":i32, "均衡故障 2":dbl, "均衡故障 3":dbl, "均衡故障 4":dbl, "均衡故障 5":dbl, "均衡故障 6":dbl, "均衡故障 7":dbl, "均衡故障 8":dbl, "均衡故障 9":dbl, "均衡故障 10":dbl, "均衡故障 11":dbl, "均衡故障 12":dbl}, "1 37":cluster{"均衡故障":i32, "均衡故障 2":dbl, "均衡故障 3":dbl, "均衡故障 4":dbl, "均衡故障 5":dbl, "均衡故障 6":dbl, "均衡故障 7":dbl, "均衡故障 8":dbl, "均衡故障 9":dbl, "均衡故障 10":dbl, "均衡故障 11":dbl, "均衡故障 12":dbl}, "1 26":cluster{"均衡故障":i32, "均衡故障 2":dbl, "均衡故障 3":dbl, "均衡故障 4":dbl, "均衡故障 5":dbl, "均衡故障 6":dbl, "均衡故障 7":dbl, "均衡故障 8":dbl, "均衡故障 9":dbl, "均衡故障 10":dbl, "均衡故障 11":dbl, "均衡故障 12":dbl}, "1 40":cluster{"均衡故障":i32, "均衡故障 2":dbl, "均衡故障 3":dbl, "均衡故障 4":dbl, "均衡故障 5":dbl, "均衡故障 6":dbl, "均衡故障 7":dbl, "均衡故障 8":dbl, "均衡故障 9":dbl, "均衡故障 10":dbl, "均衡故障 11":dbl, "均衡故障 12":dbl}, "1 14":cluster{"均衡故障":i32, "均衡故障 2":dbl, "均衡故障 3":dbl, "均衡故障 4":dbl, "均衡故障 5":dbl, "均衡故障 6":dbl, "均衡故障 7":dbl, "均衡故障 8":dbl, "均衡故障 9":dbl, "均衡故障 10":dbl, "均衡故障 11":dbl, "均衡故障 12":dbl}, "1 17":cluster{"均衡故障":i32, "均衡故障 2":dbl, "均衡故障 3":dbl, "均衡故障 4":dbl, "均衡故障 5":dbl, "均衡故障 6":dbl, "均衡故障 7":dbl, "均衡故障 8":dbl, "均衡故障 9":dbl, "均衡故障 10":dbl, "均衡故障 11":dbl, "均衡故障 12":dbl}, "1 31":cluster{"均衡故障":i32, "均衡故障 2":dbl, "均衡故障 3":dbl, "均衡故障 4":dbl, "均衡故障 5":dbl, "均衡故障 6":dbl, "均衡故障 7":dbl, "均衡故障 8":dbl, "均衡故障 9":dbl, "均衡故障 10":dbl, "均衡故障 11":dbl, "均衡故障 12":dbl}, "1 34":cluster{"均衡故障":i32, "均衡故障 2":dbl, "均衡故障 3":dbl, "均衡故障 4":dbl, "均衡故障 5":dbl, "均衡故障 6":dbl, "均衡故障 7":dbl, "均衡故障 8":dbl, "均衡故障 9":dbl, "均衡故障 10":dbl, "均衡故障 11":dbl, "均衡故障 12":dbl}}
  T7 = cluster{"第289串":dbl, "第290串":dbl, "第291串":dbl, "第292串":dbl, "第293串":dbl, "第294串":dbl, "第295串":dbl, "第296串":dbl, "第297串":dbl, "第298串":dbl, "第299串":dbl, "第300串":dbl, "第一串 2":dbl, "第一串 4":dbl, "第一串 6":dbl, "第一串 8":dbl, "第一串 10":dbl, "第一串 12":dbl, "第一串 14":dbl, "第一串 16":dbl, "第一串 18":dbl, "第一串 20":dbl, "第一串 22":dbl, "第一串 24":dbl}
  T8 = cluster{"均衡故障":i32, "均衡故障 2":dbl, "均衡故障 3":dbl, "均衡故障 4":dbl, "均衡故障 5":dbl, "均衡故障 6":dbl, "均衡故障 7":dbl, "均衡故障 8":dbl, "均衡故障 9":dbl, "均衡故障 10":dbl, "均衡故障 11":dbl, "均衡故障 12":dbl}
  T9 = cluster{"充电1":u32, "充电1":u32, "充电1":u32, "充电1":u32, "充电1":u32, "充电1":u32, "充电1":u32, "充电1":u32, "充电1":u32, "充电1":u32, "充电1":u32, "充电1":u32}
  T10 = cluster{"1 102":cluster{"第1串":dbl, "第2串":dbl, "第3串":dbl, "第4串":dbl, "第5串":dbl, "第6串":dbl, "第7串":dbl, "第8串":dbl, "第9串":dbl, "第10串":dbl, "第11串":dbl, "第12串":dbl, "第一串 2":dbl, "第一串 4":dbl, "第一串 6":dbl, "第一串 8":dbl, "第一串 10":dbl, "第一串 12":dbl, "第一串 14":dbl, "第一串 16":dbl, "第一串 18":dbl, "第一串 20":dbl, "第一串 22":dbl, "第一串 24":dbl}, "1 3":cluster{"第13串":dbl, "第14串":dbl, "第15串":dbl, "第16串":dbl, "第17串":dbl, "第18串":dbl, "第19串":dbl, "第20串":dbl, "第21串":dbl, "第22串":dbl, "第23串":dbl, "第24串":dbl, "第一串 2":dbl, "第一串 4":dbl, "第一串 6":dbl, "第一串 8":dbl, "第一串 10":dbl, "第一串 12":dbl, "第一串 14":dbl, "第一串 16":dbl, "第一串 18":dbl, "第一串 20":dbl, "第一串 22":dbl, "第一串 24":dbl}, "1 4":cluster{"第25串":dbl, "第26串":dbl, "第27串":dbl, "第28串":dbl, "第29串":dbl, "第30串":dbl, "第31串":dbl, "第32串":dbl, "第33串":dbl, "第34串":dbl, "第35串":dbl, "第36串":dbl, "第一串 2":dbl, "第一串 4":dbl, "第一串 6":dbl, "第一串 8":dbl, "第一串 10":dbl, "第一串 12":dbl, "第一串 14":dbl, "第一串 16":dbl, "第一串 18":dbl, "第一串 20":dbl, "第一串 22":dbl, "第一串 24":dbl}, "1 6":cluster{"第37串":dbl, "第38串":dbl, "第39串":dbl, "第40串":dbl, "第41串":dbl, "第42串":dbl, "第43串":dbl, "第44串":dbl, "第45串":dbl, "第46串":dbl, "第47串":dbl, "第48串":dbl, "第一串 2":dbl, "第一串 4":dbl, "第一串 6":dbl, "第一串 8":dbl, "第一串 10":dbl, "第一串 12":dbl, "第一串 14":dbl, "第一串 16":dbl, "第一串 18":dbl, "第一串 20":dbl, "第一串 22":dbl, "第一串 24":dbl}, "1 7":cluster{"第49串":dbl, "第50串":dbl, "第51串":dbl, "第52串":dbl, "第53串":dbl, "第54串":dbl, "第55串":dbl, "第56串":dbl, "第57串":dbl, "第58串":dbl, "第59串":dbl, "第60串":dbl, "第一串 2":dbl, "第一串 4":dbl, "第一串 6":dbl, "第一串 8":dbl, "第一串 10":dbl, "第一串 12":dbl, "第一串 14":dbl, "第一串 16":dbl, "第一串 18":dbl, "第一串 20":dbl, "第一串 22":dbl, "第一串 24":dbl}, "1 8":cluster{"第61串":dbl, "第62串":dbl, "第63串":dbl, "第64串":dbl, "第65串":dbl, "第66串":dbl, "第67串":dbl, "第68串":dbl, "第69串":dbl, "第70串":dbl, "第71串":dbl, "第72串":dbl, "第一串 2":dbl, "第一串 4":dbl, "第一串 6":dbl, "第一串 8":dbl, "第一串 10":dbl, "第一串 12":dbl, "第一串 14":dbl, "第一串 16":dbl, "第一串 18":dbl, "第一串 20":dbl, "第一串 22":dbl, "第一串 24":dbl}, "1 9":cluster{"第73串":dbl, "第74串":dbl, "第75串":dbl, "第76串":dbl, "第77串":dbl, "第78串":dbl, "第79串":dbl, "第80串":dbl, "第81串":dbl, "第82串":dbl, "第83串":dbl, "第84串":dbl, "第一串 2":dbl, "第一串 4":dbl, "第一串 6":dbl, "第一串 8":dbl, "第一串 10":dbl, "第一串 12":dbl, "第一串 14":dbl, "第一串 16":dbl, "第一串 18":dbl, "第一串 20":dbl, "第一串 22":dbl, "第一串 24":dbl}, "1 10":cluster{"第85串":dbl, "第86串":dbl, "第87串":dbl, "第88串":dbl, "第89串":dbl, "第90串":dbl, "第91串":dbl, "第92串":dbl, "第93串":dbl, "第94串":dbl, "第95串":dbl, "第96串":dbl, "第一串 2":dbl, "第一串 4":dbl, "第一串 6":dbl, "第一串 8":dbl, "第一串 10":dbl, "第一串 12":dbl, "第一串 14":dbl, "第一串 16":dbl, "第一串 18":dbl, "第一串 20":dbl, "第一串 22":dbl, "第一串 24":dbl}}
  T11 = cluster{"1 26":cluster{"第97串":dbl, "第98串":dbl, "第99串":dbl, "第100串":dbl, "第101串":dbl, "第102串":dbl, "第103串":dbl, "第104串":dbl, "第105串":dbl, "第106串":dbl, "第107串":dbl, "第108串":dbl, "第一串 2":dbl, "第一串 4":dbl, "第一串 6":dbl, "第一串 8":dbl, "第一串 10":dbl, "第一串 12":dbl, "第一串 14":dbl, "第一串 16":dbl, "第一串 18":dbl, "第一串 20":dbl, "第一串 22":dbl, "第一串 24":dbl}, "1 27":cluster{"第109串":dbl, "第110串":dbl, "第111串":dbl, "第112串":dbl, "第113串":dbl, "第114串":dbl, "第115串":dbl, "第116串":dbl, "第117串":dbl, "第118串":dbl, "第119串":dbl, "第120串":dbl, "第一串 2":dbl, "第一串 4":dbl, "第一串 6":dbl, "第一串 8":dbl, "第一串 10":dbl, "第一串 12":dbl, "第一串 14":dbl, "第一串 16":dbl, "第一串 18":dbl, "第一串 20":dbl, "第一串 22":dbl, "第一串 24":dbl}, "1 28":cluster{"第121串":dbl, "第122串":dbl, "第123串":dbl, "第124串":dbl, "第125串":dbl, "第126串":dbl, "第127串":dbl, "第128串":dbl, "第129串":dbl, "第130串":dbl, "第131串":dbl, "第132串":dbl, "第一串 2":dbl, "第一串 4":dbl, "第一串 6":dbl, "第一串 8":dbl, "第一串 10":dbl, "第一串 12":dbl, "第一串 14":dbl, "第一串 16":dbl, "第一串 18":dbl, "第一串 20":dbl, "第一串 22":dbl, "第一串 24":dbl}, "1 29":cluster{"第133串":dbl, "第134串":dbl, "第135串":dbl, "第136串":dbl, "第137串":dbl, "第138串":dbl, "第139串":dbl, "第140串":dbl, "第141串":dbl, "第142串":dbl, "第143串":dbl, "第144串":dbl, "第一串 2":dbl, "第一串 4":dbl, "第一串 6":dbl, "第一串 8":dbl, "第一串 10":dbl, "第一串 12":dbl, "第一串 14":dbl, "第一串 16":dbl, "第一串 18":dbl, "第一串 20":dbl, "第一串 22":dbl, "第一串 24":dbl}, "1 30":cluster{"第145串":dbl, "第146串":dbl, "第147串":dbl, "第148串":dbl, "第149串":dbl, "第150串":dbl, "第151串":dbl, "第152串":dbl, "第153串":dbl, "第154串":dbl, "第155串":dbl, "第156串":dbl, "第一串 2":dbl, "第一串 4":dbl, "第一串 6":dbl, "第一串 8":dbl, "第一串 10":dbl, "第一串 12":dbl, "第一串 14":dbl, "第一串 16":dbl, "第一串 18":dbl, "第一串 20":dbl, "第一串 22":dbl, "第一串 24":dbl}, "1 31":cluster{"第157串":dbl, "第158串":dbl, "第159串":dbl, "第160串":dbl, "第161串":dbl, "第162串":dbl, "第163串":dbl, "第164串":dbl, "第165串":dbl, "第166串":dbl, "第167串":dbl, "第168串":dbl, "第一串 2":dbl, "第一串 4":dbl, "第一串 6":dbl, "第一串 8":dbl, "第一串 10":dbl, "第一串 12":dbl, "第一串 14":dbl, "第一串 16":dbl, "第一串 18":dbl, "第一串 20":dbl, "第一串 22":dbl, "第一串 24":dbl}, "1 32":cluster{"第169串":dbl, "第170串":dbl, "第171串":dbl, "第172串":dbl, "第173串":dbl, "第174串":dbl, "第175串":dbl, "第176串":dbl, "第177串":dbl, "第178串":dbl, "第179串":dbl, "第180串":dbl, "第一串 2":dbl, "第一串 4":dbl, "第一串 6":dbl, "第一串 8":dbl, "第一串 10":dbl, "第一串 12":dbl, "第一串 14":dbl, "第一串 16":dbl, "第一串 18":dbl, "第一串 20":dbl, "第一串 22":dbl, "第一串 24":dbl}, "1 33":cluster{"第181串":dbl, "第182串":dbl, "第183串":dbl, "第184串":dbl, "第185串":dbl, "第186串":dbl, "第187串":dbl, "第188串":dbl, "第189串":dbl, "第190串":dbl, "第191串":dbl, "第192串":dbl, "第一串 2":dbl, "第一串 4":dbl, "第一串 6":dbl, "第一串 8":dbl, "第一串 10":dbl, "第一串 12":dbl, "第一串 14":dbl, "第一串 16":dbl, "第一串 18":dbl, "第一串 20":dbl, "第一串 22":dbl, "第一串 24":dbl}}
  T12 = cluster{"1 18":cluster{"第193串":dbl, "第194串":dbl, "第195串":dbl, "第196串":dbl, "第197串":dbl, "第198串":dbl, "第199串":dbl, "第200串":dbl, "第201串":dbl, "第202串":dbl, "第203串":dbl, "第204串":dbl, "第一串 2":dbl, "第一串 4":dbl, "第一串 6":dbl, "第一串 8":dbl, "第一串 10":dbl, "第一串 12":dbl, "第一串 14":dbl, "第一串 16":dbl, "第一串 18":dbl, "第一串 20":dbl, "第一串 22":dbl, "第一串 24":dbl}, "1 19":cluster{"第205串":dbl, "第206串":dbl, "第207串":dbl, "第208串":dbl, "第209串":dbl, "第210串":dbl, "第211串":dbl, "第212串":dbl, "第213串":dbl, "第214串":dbl, "第215串":dbl, "第216串":dbl, "第一串 2":dbl, "第一串 4":dbl, "第一串 6":dbl, "第一串 8":dbl, "第一串 10":dbl, "第一串 12":dbl, "第一串 14":dbl, "第一串 16":dbl, "第一串 18":dbl, "第一串 20":dbl, "第一串 22":dbl, "第一串 24":dbl}, "1 20":cluster{"第217串":dbl, "第218串":dbl, "第219串":dbl, "第220串":dbl, "第221串":dbl, "第222串":dbl, "第223串":dbl, "第224串":dbl, "第225串":dbl, "第226串":dbl, "第227串":dbl, "第228串":dbl, "第一串 2":dbl, "第一串 4":dbl, "第一串 6":dbl, "第一串 8":dbl, "第一串 10":dbl, "第一串 12":dbl, "第一串 14":dbl, "第一串 16":dbl, "第一串 18":dbl, "第一串 20":dbl, "第一串 22":dbl, "第一串 24":dbl}, "1 21":cluster{"第229串":dbl, "第230串":dbl, "第231串":dbl, "第232串":dbl, "第233串":dbl, "第234串":dbl, "第235串":dbl, "第236串":dbl, "第237串":dbl, "第238串":dbl, "第239串":dbl, "第240串":dbl, "第一串 2":dbl, "第一串 4":dbl, "第一串 6":dbl, "第一串 8":dbl, "第一串 10":dbl, "第一串 12":dbl, "第一串 14":dbl, "第一串 16":dbl, "第一串 18":dbl, "第一串 20":dbl, "第一串 22":dbl, "第一串 24":dbl}, "1 22":cluster{"第241串":dbl, "第242串":dbl, "第243串":dbl, "第244串":dbl, "第245串":dbl, "第246串":dbl, "第247串":dbl, "第248串":dbl, "第249串":dbl, "第250串":dbl, "第251串":dbl, "第252串":dbl, "第一串 2":dbl, "第一串 4":dbl, "第一串 6":dbl, "第一串 8":dbl, "第一串 10":dbl, "第一串 12":dbl, "第一串 14":dbl, "第一串 16":dbl, "第一串 18":dbl, "第一串 20":dbl, "第一串 22":dbl, "第一串 24":dbl}, "1 23":cluster{"第253串":dbl, "第254串":dbl, "第255串":dbl, "第256串":dbl, "第257串":dbl, "第258串":dbl, "第259串":dbl, "第260串":dbl, "第261串":dbl, "第262串":dbl, "第263串":dbl, "第264串":dbl, "第一串 2":dbl, "第一串 4":dbl, "第一串 6":dbl, "第一串 8":dbl, "第一串 10":dbl, "第一串 12":dbl, "第一串 14":dbl, "第一串 16":dbl, "第一串 18":dbl, "第一串 20":dbl, "第一串 22":dbl, "第一串 24":dbl}, "1 24":cluster{"第265串":dbl, "第266串":dbl, "第267串":dbl, "第268串":dbl, "第269串":dbl, "第270串":dbl, "第271串":dbl, "第272串":dbl, "第273串":dbl, "第274串":dbl, "第275串":dbl, "第276串":dbl, "第一串 2":dbl, "第一串 4":dbl, "第一串 6":dbl, "第一串 8":dbl, "第一串 10":dbl, "第一串 12":dbl, "第一串 14":dbl, "第一串 16":dbl, "第一串 18":dbl, "第一串 20":dbl, "第一串 22":dbl, "第一串 24":dbl}, "1 25":cluster{"第277串":dbl, "第278串":dbl, "第279串":dbl, "第280串":dbl, "第281串":dbl, "第282串":dbl, "第283串":dbl, "第284串":dbl, "第285串":dbl, "第286串":dbl, "第287串":dbl, "第288串":dbl, "第一串 2":dbl, "第一串 4":dbl, "第一串 6":dbl, "第一串 8":dbl, "第一串 10":dbl, "第一串 12":dbl, "第一串 14":dbl, "第一串 16":dbl, "第一串 18":dbl, "第一串 20":dbl, "第一串 22":dbl, "第一串 24":dbl}}
  T13 = cluster{"1 3":cluster{"第13串":dbl, "第14串":dbl, "第15串":dbl, "第16串":dbl, "第17串":dbl, "第18串":dbl, "第19串":dbl, "第20串":dbl, "第21串":dbl, "第22串":dbl, "第23串":dbl, "第24串":dbl, "第一串 2":dbl, "第一串 4":dbl, "第一串 6":dbl, "第一串 8":dbl, "第一串 10":dbl, "第一串 12":dbl, "第一串 14":dbl, "第一串 16":dbl, "第一串 18":dbl, "第一串 20":dbl, "第一串 22":dbl, "第一串 24":dbl}, "1 4":cluster{"第25串":dbl, "第26串":dbl, "第27串":dbl, "第28串":dbl, "第29串":dbl, "第30串":dbl, "第31串":dbl, "第32串":dbl, "第33串":dbl, "第34串":dbl, "第35串":dbl, "第36串":dbl, "第一串 2":dbl, "第一串 4":dbl, "第一串 6":dbl, "第一串 8":dbl, "第一串 10":dbl, "第一串 12":dbl, "第一串 14":dbl, "第一串 16":dbl, "第一串 18":dbl, "第一串 20":dbl, "第一串 22":dbl, "第一串 24":dbl}, "1 6":cluster{"第37串":dbl, "第38串":dbl, "第39串":dbl, "第40串":dbl, "第41串":dbl, "第42串":dbl, "第43串":dbl, "第44串":dbl, "第45串":dbl, "第46串":dbl, "第47串":dbl, "第48串":dbl, "第一串 2":dbl, "第一串 4":dbl, "第一串 6":dbl, "第一串 8":dbl, "第一串 10":dbl, "第一串 12":dbl, "第一串 14":dbl, "第一串 16":dbl, "第一串 18":dbl, "第一串 20":dbl, "第一串 22":dbl, "第一串 24":dbl}, "1 7":cluster{"第49串":dbl, "第50串":dbl, "第51串":dbl, "第52串":dbl, "第53串":dbl, "第54串":dbl, "第55串":dbl, "第56串":dbl, "第57串":dbl, "第58串":dbl, "第59串":dbl, "第60串":dbl, "第一串 2":dbl, "第一串 4":dbl, "第一串 6":dbl, "第一串 8":dbl, "第一串 10":dbl, "第一串 12":dbl, "第一串 14":dbl, "第一串 16":dbl, "第一串 18":dbl, "第一串 20":dbl, "第一串 22":dbl, "第一串 24":dbl}, "1 8":cluster{"第61串":dbl, "第62串":dbl, "第63串":dbl, "第64串":dbl, "第65串":dbl, "第66串":dbl, "第67串":dbl, "第68串":dbl, "第69串":dbl, "第70串":dbl, "第71串":dbl, "第72串":dbl, "第一串 2":dbl, "第一串 4":dbl, "第一串 6":dbl, "第一串 8":dbl, "第一串 10":dbl, "第一串 12":dbl, "第一串 14":dbl, "第一串 16":dbl, "第一串 18":dbl, "第一串 20":dbl, "第一串 22":dbl, "第一串 24":dbl}, "1 9":cluster{"第73串":dbl, "第74串":dbl, "第75串":dbl, "第76串":dbl, "第77串":dbl, "第78串":dbl, "第79串":dbl, "第80串":dbl, "第81串":dbl, "第82串":dbl, "第83串":dbl, "第84串":dbl, "第一串 2":dbl, "第一串 4":dbl, "第一串 6":dbl, "第一串 8":dbl, "第一串 10":dbl, "第一串 12":dbl, "第一串 14":dbl, "第一串 16":dbl, "第一串 18":dbl, "第一串 20":dbl, "第一串 22":dbl, "第一串 24":dbl}, "1 10":cluster{"第85串":dbl, "第86串":dbl, "第87串":dbl, "第88串":dbl, "第89串":dbl, "第90串":dbl, "第91串":dbl, "第92串":dbl, "第93串":dbl, "第94串":dbl, "第95串":dbl, "第96串":dbl, "第一串 2":dbl, "第一串 4":dbl, "第一串 6":dbl, "第一串 8":dbl, "第一串 10":dbl, "第一串 12":dbl, "第一串 14":dbl, "第一串 16":dbl, "第一串 18":dbl, "第一串 20":dbl, "第一串 22":dbl, "第一串 24":dbl}, "1 102":cluster{"第1串":dbl, "第2串":dbl, "第3串":dbl, "第4串":dbl, "第5串":dbl, "第6串":dbl, "第7串":dbl, "第8串":dbl, "第9串":dbl, "第10串":dbl, "第11串":dbl, "第12串":dbl, "第一串 2":dbl, "第一串 4":dbl, "第一串 6":dbl, "第一串 8":dbl, "第一串 10":dbl, "第一串 12":dbl, "第一串 14":dbl, "第一串 16":dbl, "第一串 18":dbl, "第一串 20":dbl, "第一串 22":dbl, "第一串 24":dbl}}
  T14 = enum32{"Invalid", "Standard", "Closed", "Hidden", "Minimized", "Maximized"}
  T15 = cluster{"[0]":u32, "[1]":u32, "[2]":u32, "[3]":u32, "[4]":u32, "[5]":u32, "[6]":u32, "[7]":u32, "[8]":u32, "[9]":u32, "[10]":u32, "[11]":u32}
  T16 = cluster{"[0]":dbl, "[1]":dbl, "[2]":dbl, "[3]":dbl, "[4]":dbl, "[5]":dbl, "[6]":dbl, "[7]":dbl, "[8]":dbl, "[9]":dbl, "[10]":dbl, "[11]":dbl}
  T17 = cluster{"[0]":dbl, "[1]":dbl, "[2]":dbl, "[3]":dbl, "[4]":dbl, "[5]":dbl, "[6]":dbl, "[7]":dbl, "[8]":dbl, "[9]":dbl, "[10]":dbl, "[11]":dbl, "[12]":dbl, "[13]":dbl, "[14]":dbl, "[15]":dbl, "[16]":dbl, "[17]":dbl, "[18]":dbl, "[19]":dbl, "[20]":dbl, "[21]":dbl, "[22]":dbl, "[23]":dbl}
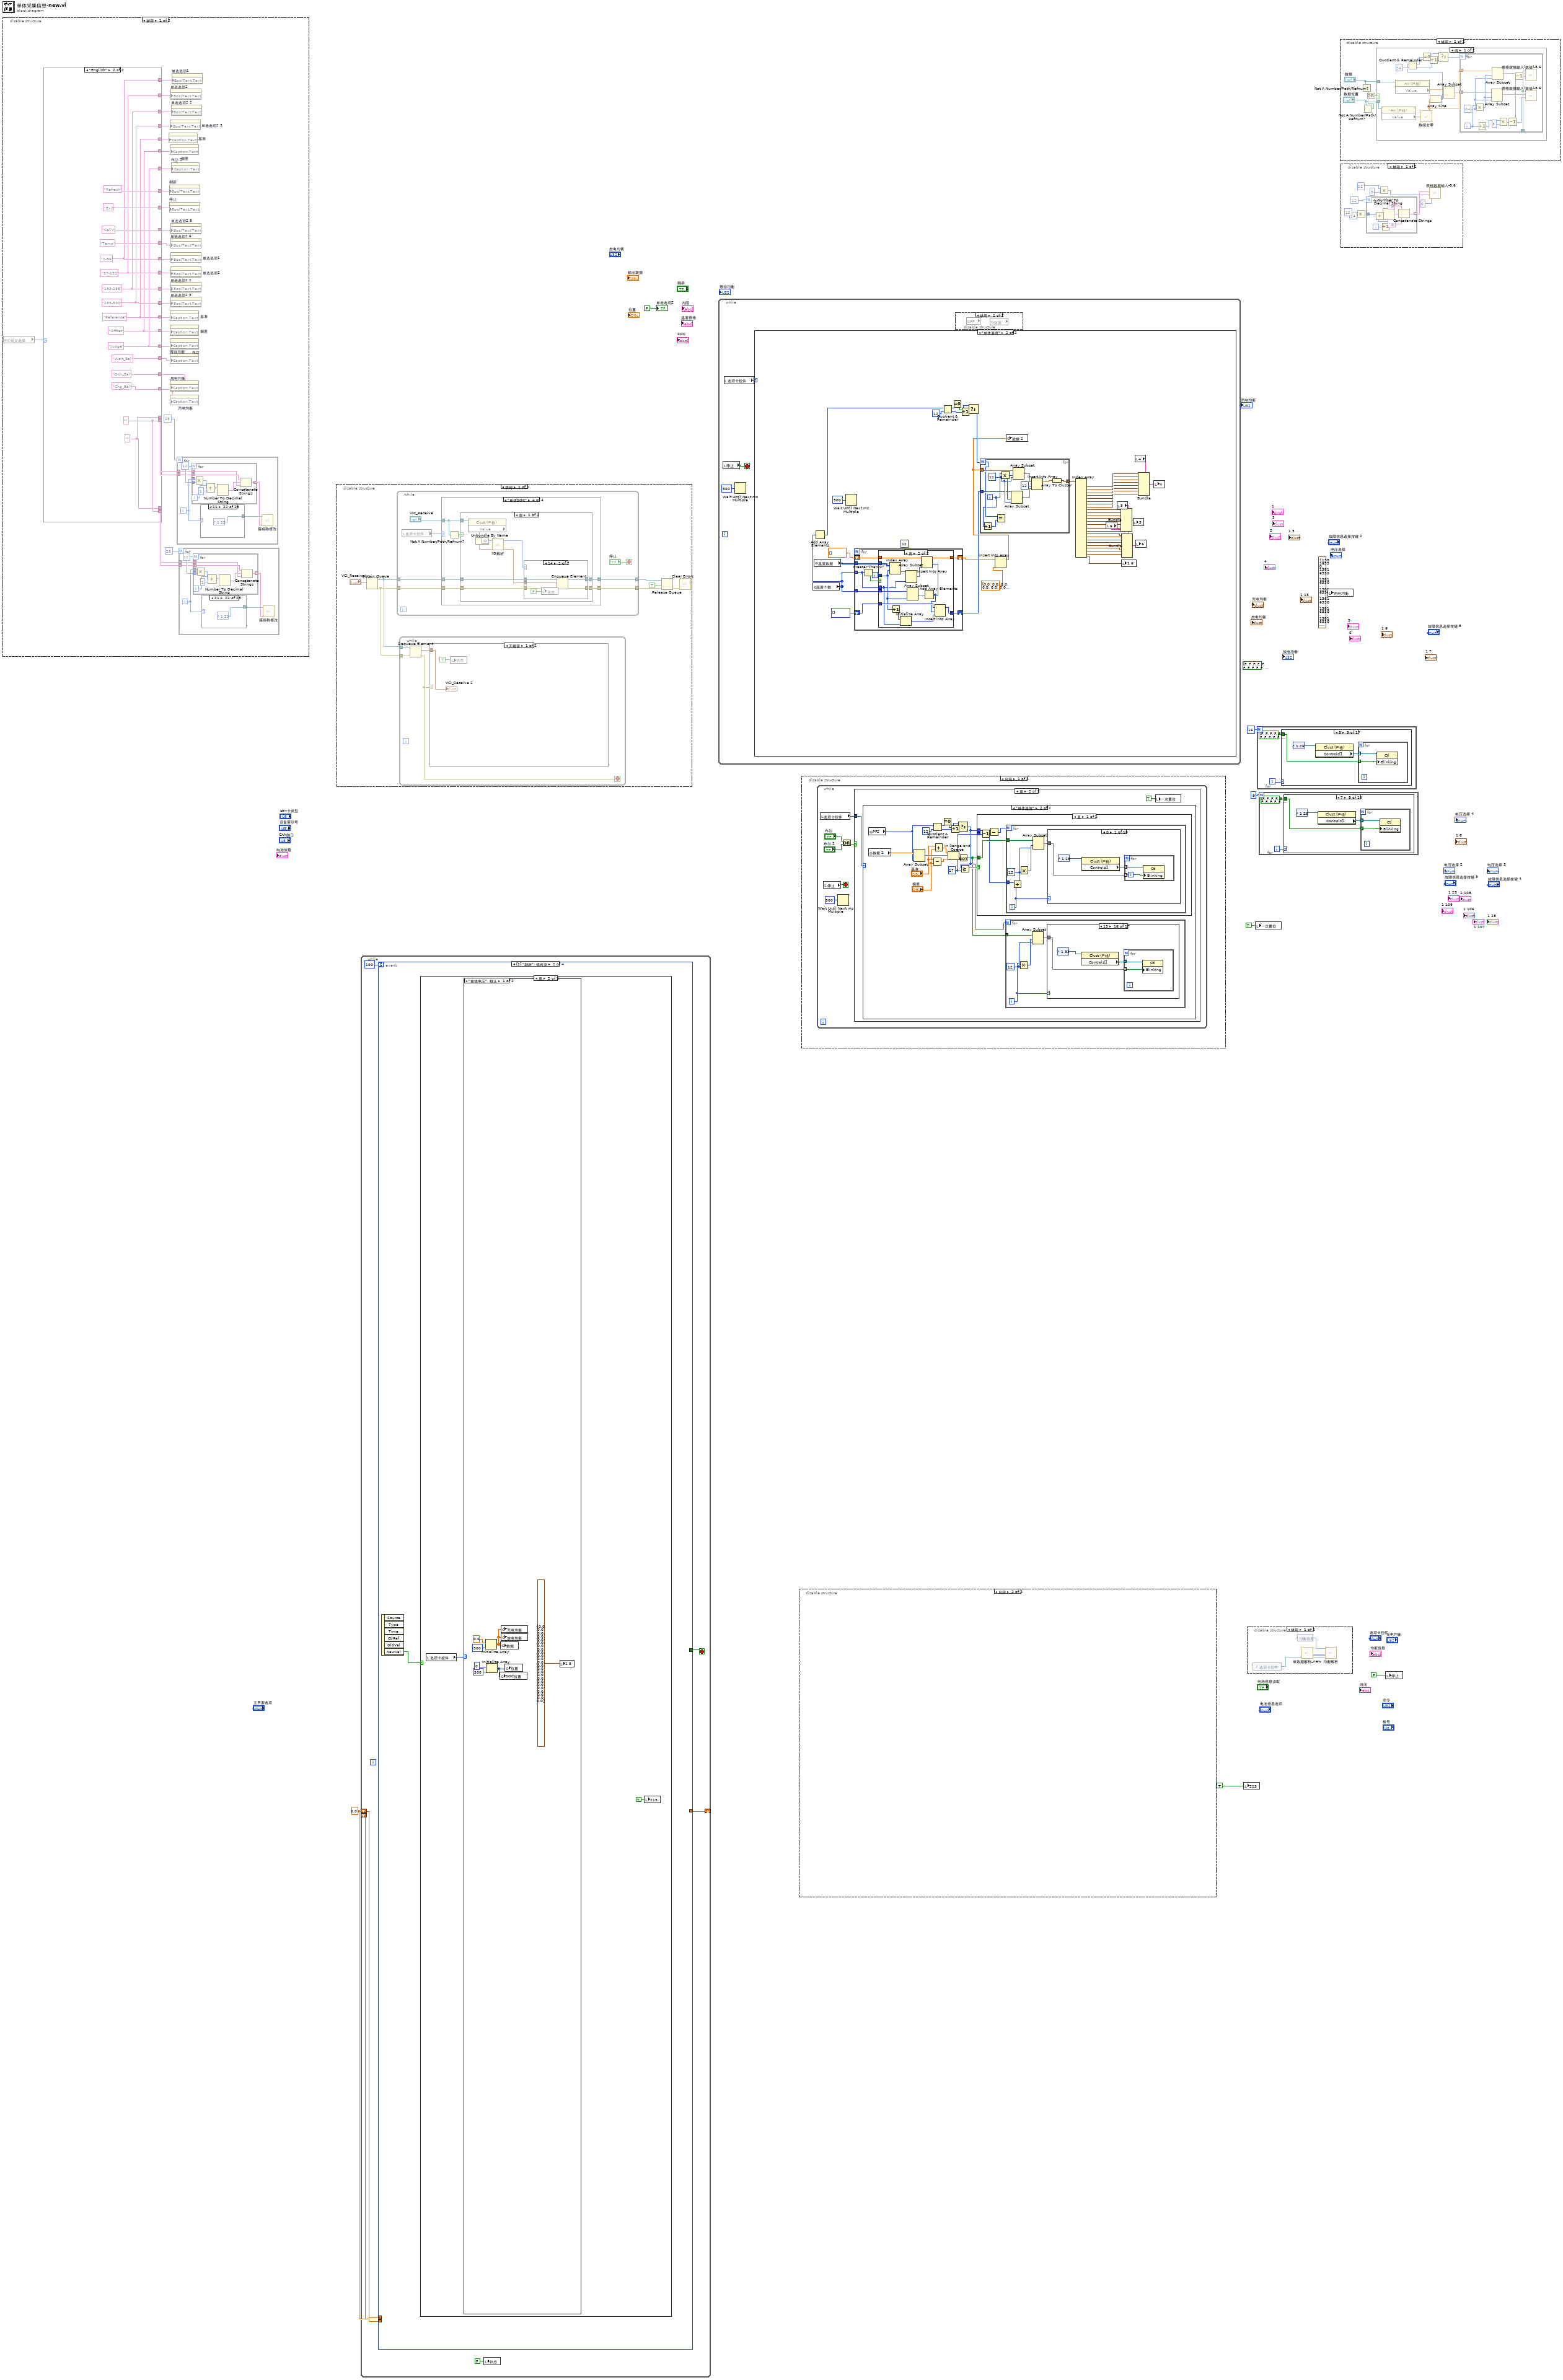
[diagram p0: block diagram]
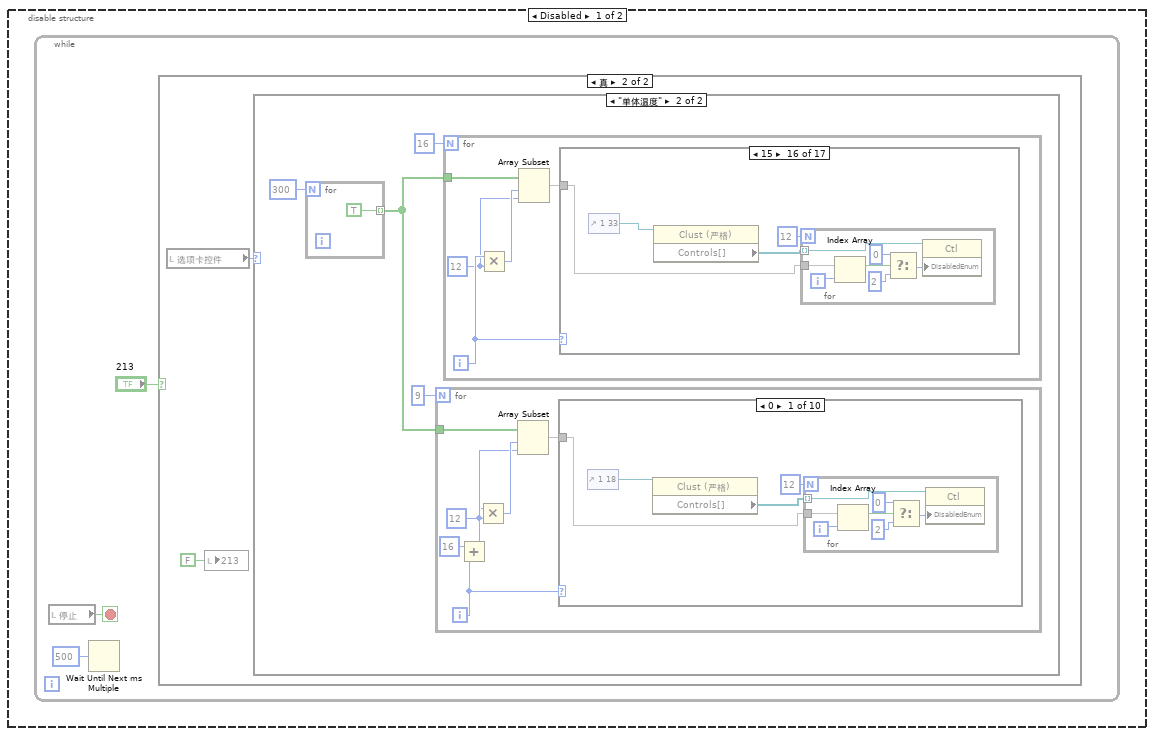
[diagram p2: hidden frame]
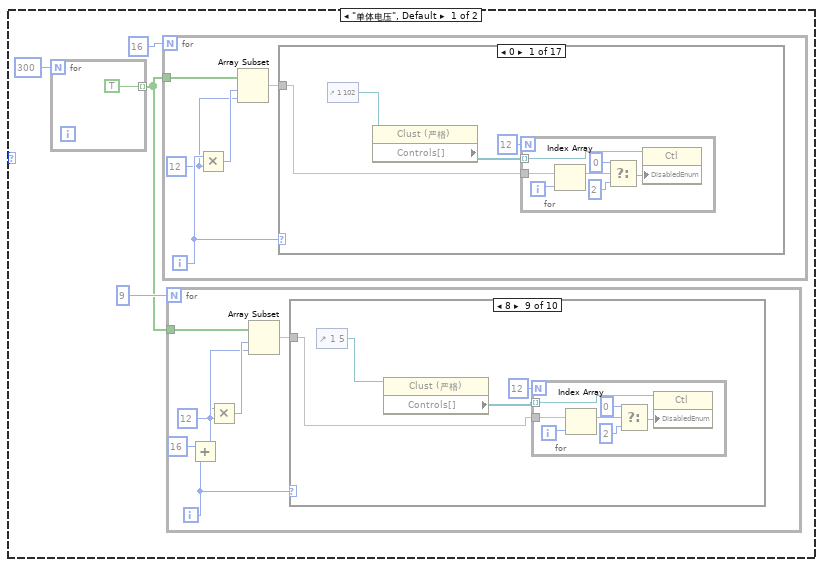
[diagram p4: hidden frame]
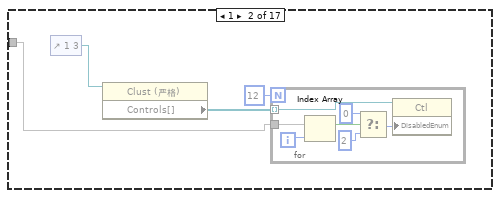
[diagram p5: hidden frame]
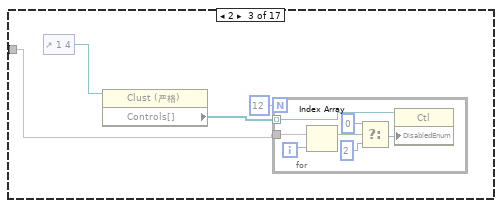
[diagram p6: hidden frame]
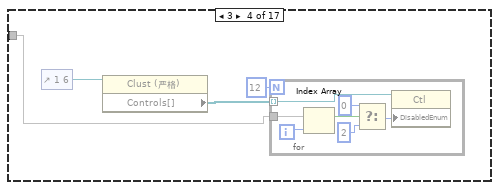
[diagram p7: hidden frame]
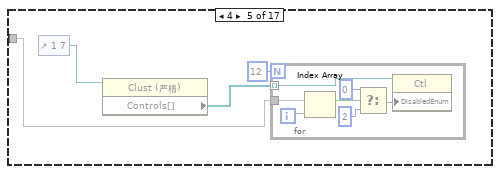
[diagram p8: hidden frame]
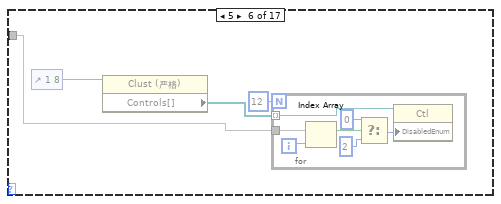
[diagram p9: hidden frame]
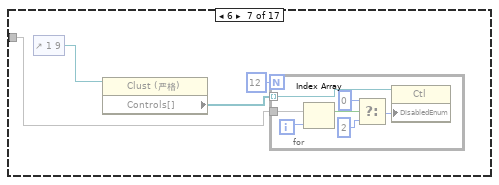
[diagram p10: hidden frame]
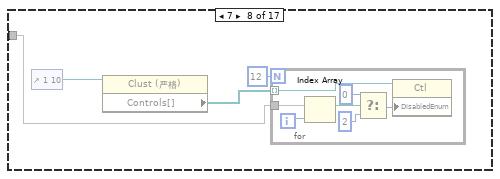
[diagram p11: hidden frame]
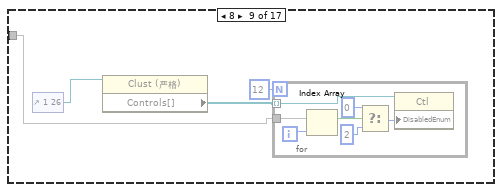
[diagram p12: hidden frame]
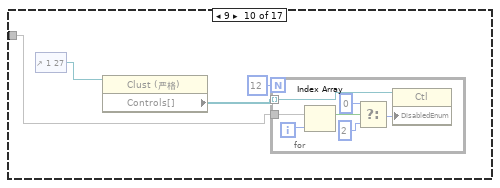
[diagram p13: hidden frame]
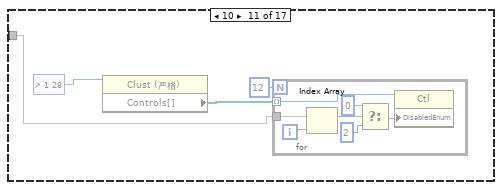
[diagram p14: hidden frame]
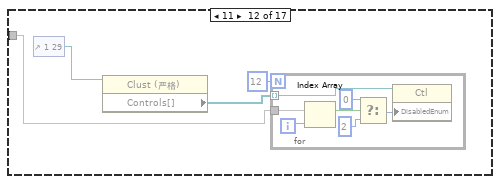
[diagram p15: hidden frame]
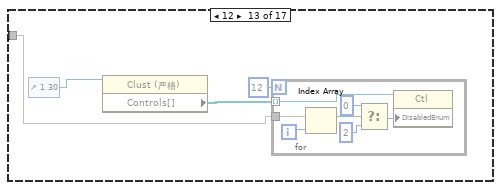
[diagram p16: hidden frame]
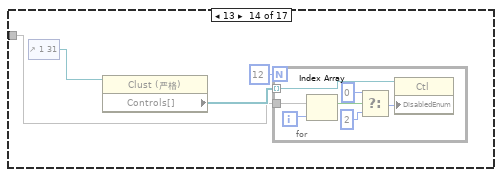
[diagram p17: hidden frame]
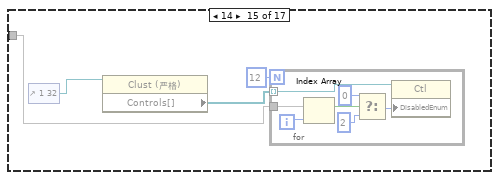
[diagram p18: hidden frame]
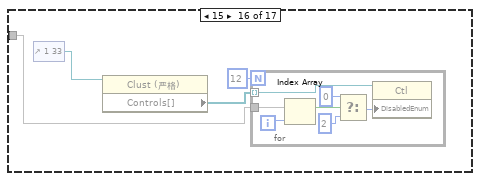
[diagram p19: hidden frame]
diagram:
  w1 = 0.0 ("life")
  (unwired) bool[] [FALSE, FALSE, FALSE, FALSE, FALSE, FALSE, FALSE, FALSE, FALSE, FALSE, FALSE, FALSE, FALSE]
  n1 = disable-structure shown="禁用" {
    frame Disabled {
      n2 = global read "中英文全局.vi" "中英文选择"() -> (w36:enum32{"中文", "English"})
      n3 = case shown="\"English\"" w36 {
        tunnel: ["单体电压" "CellV"] -> w35
        tunnel: ["单体温度" "Temp"] -> w34
        tunnel: [w125 w141] -> w33
        tunnel: [w124 w140] -> w32
        tunnel: [w123 w139] -> w31
        tunnel: [w122 w138] -> w30
        tunnel: [w121 w137] -> w29
        tunnel: [w120 w136] -> w28
        tunnel: [w119 w135] -> w27
        tunnel: ["等待均衡" "Wait_Bal"] -> w26
        tunnel: ["放电均衡" "Dch_Bal"] -> w25
        tunnel: ["充电均衡" "Chg_Bal"] -> w24
        tunnel: [w129 w145] -> w22
        tunnel: [w128 w144] -> w21
        tunnel: [w129 w145] -> w19
        tunnel: [w128 w144] -> w20
        tunnel: ["刷新" "Refresh"] -> w17
        tunnel: ["退出" "Exit"] -> w16
        tunnel: [w125 w141] -> w15
        tunnel: [w124 w140] -> w14
        tunnel: [w123 w139] -> w13
        tunnel: [w122 w138] -> w12
        tunnel: [w121 w137] -> w11
        tunnel: [w120 w136] -> w10
        tunnel: [w119 w135] -> w9
        frame "中文", Default {
          w128 = "串"
          w129 = "第"
          w119 = "判定"
          w120 = "偏差"
          w121 = "基准"
          w122 = "289串-300串"
          w123 = "193串-288串"
          w124 = "97串-192串"
          w125 = "1串-96串"
        }
        frame "English" {
          w144 = ""
          w145 = ""
          w135 = "Judge"
          w136 = "Offset"
          w137 = "Reference"
          w138 = "289-300"
          w139 = "193-288"
          w140 = "97-192"
          w141 = "1-96"
        }
      }
      n4 = property on="基准" class="DigNum (严格)"("Caption.Text"=w11) -> ()  [unwired: 2 in, 2 out]
      n5 = property on="刷新" class="Bool (严格)"("BoolText.Text"=w17) -> ()  [unwired: 2 in, 2 out]
      n6 = property on="停止" class="Bool (严格)"("BoolText.Text"=w16) -> ()  [unwired: 2 in, 2 out]
      n7 = property on="单选选项2 3" class="Bool (严格)"("BoolText.Text"=w12) -> ()  [unwired: 2 in, 2 out]
      n8 = property on="偏差" class="DigNum (严格)"("Caption.Text"=w10) -> ()  [unwired: 2 in, 2 out]
      n9 = property on="基准" class="DigNum (严格)"("Caption.Text"=w29) -> ()  [unwired: 2 in, 2 out]
      n10 = property on="偏差" class="DigNum (严格)"("Caption.Text"=w28) -> ()  [unwired: 2 in, 2 out]
      n11 = property on="布尔" class="Bool (严格)"("Caption.Text"=w27) -> ()  [unwired: 2 in, 2 out]
      n12 = property on="等待均衡" class="ColBox"("Caption.Text"=w26) -> ()  [unwired: 2 in, 2 out]
      n13 = property on="放电均衡" class="ColBox"("Caption.Text"=w25) -> ()  [unwired: 2 in, 2 out]
      n14 = property on="充电均衡" class="ColBox"("Caption.Text"=w24) -> ()  [unwired: 2 in, 2 out]
      n15 = property on="单选选项2" class="Bool (严格)"("BoolText.Text"=w14) -> ()  [unwired: 2 in, 2 out]
      n16 = property on="单选选项2 5" class="Bool (严格)"("BoolText.Text"=w35) -> ()  [unwired: 2 in, 2 out]
      n17 = property on="单选选项2 6" class="Bool (严格)"("BoolText.Text"=w34) -> ()  [unwired: 2 in, 2 out]
      n18 = property on="单选选项1" class="Bool (严格)"("BoolText.Text"=w33) -> ()  [unwired: 2 in, 2 out]
      n19 = property on="单选选项2" class="Bool (严格)"("BoolText.Text"=w32) -> ()  [unwired: 2 in, 2 out]
      n20 = property on="单选选项2 2" class="Bool (严格)"("BoolText.Text"=w31) -> ()  [unwired: 2 in, 2 out]
      n21 = property on="单选选项2 3" class="Bool (严格)"("BoolText.Text"=w30) -> ()  [unwired: 2 in, 2 out]
      n22 = property on="单选选项2 2" class="Bool (严格)"("BoolText.Text"=w13) -> ()  [unwired: 2 in, 2 out]
      n23 = property on="布尔 2" class="Bool (严格)"("Caption.Text"=w9) -> ()  [unwired: 2 in, 2 out]
      n24 = property on="单选选项1" class="Bool (严格)"("BoolText.Text"=w15) -> ()  [unwired: 2 in, 2 out]
      n25 = for {
        N: 25 -> [_]
        tunnel: w22 -> [w79]
        tunnel: w21 -> [w78]
        i -> [w80]
        w83 = 12
        n26 = for {
          N: w83 -> [_]
          tunnel: [w117] -> w81 mode=indexing
          tunnel: w80 -> [w114]
          tunnel: w83 -> [w113]
          tunnel: w79 -> [w110]
          tunnel: w78 -> [w109]
          i -> [w116]
          n27 = Multiply(x=w114, y=w113) -> (x*y=w115:i32)
          n28 = Compound Arithmetic op=ADD(w116, w115, 1 ("值")) -> (w111:i32)
          n29 = Number To Decimal String(number=w111) -> (decimal integer string=w118:string)  [unwired: 1 in]
          n30 = Concatenate Strings(w110, w118, w109) -> (w117:string)
        }
        n31 = case shown="21" w80 {
          tunnel: [w84 w85 w86 w87 w88 w89 w90 w91 w92 w93 w94 w95 w96 w97 w98 w99 w100 w101 w102 w103 w104 w105 w106 w107 w108] -> w82
          frame 0, Default {
            n32 = control-ref of="1 102"() -> (w84:refnum<vi>)
          }
          frame 1 {
            n33 = control-ref of="1 3"() -> (w85:refnum<vi>)
          }
          frame 2 {
            n34 = control-ref of="1 4"() -> (w86:refnum<vi>)
          }
          frame 3 {
            n35 = control-ref of="1 6"() -> (w87:refnum<vi>)
          }
          frame 4 {
            n36 = control-ref of="1 7"() -> (w88:refnum<vi>)
          }
          frame 5 {
            n37 = control-ref of="1 8"() -> (w89:refnum<vi>)
          }
          frame 6 {
            n38 = control-ref of="1 9"() -> (w90:refnum<vi>)
          }
          frame 7 {
            n39 = control-ref of="1 10"() -> (w91:refnum<vi>)
          }
          frame 8 {
            n40 = control-ref of="1 26"() -> (w92:refnum<vi>)
          }
          frame 9 {
            n41 = control-ref of="1 27"() -> (w93:refnum<vi>)
          }
          frame 10 {
            n42 = control-ref of="1 28"() -> (w94:refnum<vi>)
          }
          frame 11 {
            n43 = control-ref of="1 29"() -> (w95:refnum<vi>)
          }
          frame 12 {
            n44 = control-ref of="1 30"() -> (w96:refnum<vi>)
          }
          frame 13 {
            n45 = control-ref of="1 31"() -> (w97:refnum<vi>)
          }
          frame 14 {
            n46 = control-ref of="1 32"() -> (w98:refnum<vi>)
          }
          frame 15 {
            n47 = control-ref of="1 33"() -> (w99:refnum<vi>)
          }
          frame 16 {
            n48 = control-ref of="1 18"() -> (w100:refnum<vi>)
          }
          frame 17 {
            n49 = control-ref of="1 19"() -> (w101:refnum<vi>)
          }
          frame 18 {
            n50 = control-ref of="1 20"() -> (w102:refnum<vi>)
          }
          frame 19 {
            n51 = control-ref of="1 21"() -> (w103:refnum<vi>)
          }
          frame 20 {
            n52 = control-ref of="1 22"() -> (w104:refnum<vi>)
          }
          frame 21 {
            n53 = control-ref of="1 23"() -> (w105:refnum<vi>)
          }
          frame 22 {
            n54 = control-ref of="1 24"() -> (w106:refnum<vi>)
          }
          frame 23 {
            n55 = control-ref of="1 25"() -> (w107:refnum<vi>)
          }
          frame 24 {
            n56 = control-ref of="1 5"() -> (w108:refnum<vi>)
          }
        }
        n57 = call "簇名称修改.vi"("输入名称"=w81, "簇引用"=w82) -> ()  [unwired: 10 in]
      }
      n58 = for {
        N: 25 -> [_]
        tunnel: w19 -> [w38]
        tunnel: w20 -> [w37]
        i -> [w39]
        w42 = 12
        n59 = for {
          N: w42 -> [_]
          tunnel: [w76] -> w40 mode=indexing
          tunnel: w39 -> [w73]
          tunnel: w42 -> [w72]
          tunnel: w38 -> [w69]
          tunnel: w37 -> [w68]
          i -> [w75]
          n60 = Multiply(x=w73, y=w72) -> (x*y=w74:i32)
          n61 = Compound Arithmetic op=ADD(w75, w74, 1 ("值")) -> (w70:i32)
          n62 = Number To Decimal String(number=w70) -> (decimal integer string=w77:string)  [unwired: 1 in]
          n63 = Concatenate Strings(w69, w77, w68) -> (w76:string)
        }
        n64 = case shown="21" w39 {
          tunnel: [w43 w44 w45 w46 w47 w48 w49 w50 w51 w52 w53 w54 w55 w56 w57 w58 w59 w60 w61 w62 w63 w64 w65 w66 w67] -> w41
          frame 0, Default {
            n65 = control-ref of="1 102"() -> (w43:refnum<vi>)
          }
          frame 1 {
            n66 = control-ref of="1 3"() -> (w44:refnum<vi>)
          }
          frame 2 {
            n67 = control-ref of="1 4"() -> (w45:refnum<vi>)
          }
          frame 3 {
            n68 = control-ref of="1 6"() -> (w46:refnum<vi>)
          }
          frame 4 {
            n69 = control-ref of="1 7"() -> (w47:refnum<vi>)
          }
          frame 5 {
            n70 = control-ref of="1 8"() -> (w48:refnum<vi>)
          }
          frame 6 {
            n71 = control-ref of="1 9"() -> (w49:refnum<vi>)
          }
          frame 7 {
            n72 = control-ref of="1 10"() -> (w50:refnum<vi>)
          }
          frame 8 {
            n73 = control-ref of="1 26"() -> (w51:refnum<vi>)
          }
          frame 9 {
            n74 = control-ref of="1 27"() -> (w52:refnum<vi>)
          }
          frame 10 {
            n75 = control-ref of="1 28"() -> (w53:refnum<vi>)
          }
          frame 11 {
            n76 = control-ref of="1 29"() -> (w54:refnum<vi>)
          }
          frame 12 {
            n77 = control-ref of="1 30"() -> (w55:refnum<vi>)
          }
          frame 13 {
            n78 = control-ref of="1 31"() -> (w56:refnum<vi>)
          }
          frame 14 {
            n79 = control-ref of="1 32"() -> (w57:refnum<vi>)
          }
          frame 15 {
            n80 = control-ref of="1 33"() -> (w58:refnum<vi>)
          }
          frame 16 {
            n81 = control-ref of="1 18"() -> (w59:refnum<vi>)
          }
          frame 17 {
            n82 = control-ref of="1 19"() -> (w60:refnum<vi>)
          }
          frame 18 {
            n83 = control-ref of="1 20"() -> (w61:refnum<vi>)
          }
          frame 19 {
            n84 = control-ref of="1 21"() -> (w62:refnum<vi>)
          }
          frame 20 {
            n85 = control-ref of="1 22"() -> (w63:refnum<vi>)
          }
          frame 21 {
            n86 = control-ref of="1 23"() -> (w64:refnum<vi>)
          }
          frame 22 {
            n87 = control-ref of="1 24"() -> (w65:refnum<vi>)
          }
          frame 23 {
            n88 = control-ref of="1 25"() -> (w66:refnum<vi>)
          }
          frame 24 {
            n89 = control-ref of="1 6"() -> (w67:refnum<vi>)
          }
        }
        n90 = call "簇名称修改.vi"("输入名称"=w40, "簇引用"=w41) -> ()  [unwired: 10 in]
      }
    }
    frame Enabled {
    }
  }
  n91 = disable-structure shown="禁用" {
    frame Disabled {
      n92 = Obtain Queue(element data type="VCI_Receive") -> (queue out=w156:refnum<queue>, error out=w155:errorcluster)  [unwired: 4 in, 1 out]
      n93 = while {
        tunnel: w156 -> [w167]
        tunnel: w155 -> [w166]
        tunnel: [w165] -> w154
        tunnel: [w164] -> w153
        stop <- "停止" stop-if-true
        n94 = local read "选项卡控件"() -> (w168:enum32{"单体电压", "单体温度", "单体内阻", "单体SOC"})
        n95 = case shown="\"单体SOC\"" w168 {
          tunnel: "VIC_Receive" -> [w172 w196 w220 w244]
          tunnel: w167 -> [w176 w200 w224 w248]
          tunnel: w166 -> [w175 w199 w223 w247]
          tunnel: [w174 w198 w222 w246] -> w165
          tunnel: [w173 w197 w221 w245] -> w164
          frame "单体电压", Default {
            n96 = Not A Number/Path/Refnum?(number/path/refnum=w172) -> (NaN/Path/Refnum?=w171:bool)
            n97 = case shown="假" w171 {
              tunnel: w176 -> [w183 w194]
              tunnel: w175 -> [w182 w193]
              tunnel: [w180 w194] -> w174
              tunnel: [w179 w193] -> w173
              tunnel: w172 -> [w178 _]
              frame False {
                n98 = property class="Clust (严格)"(reference=w178) -> ("Value"=w181:T1)  [unwired: 1 in, 2 out]
                n99 = Unbundle By Name(w181) -> ("ID"=w184:u32)
                n100 = call "ID解析.vi"("ID"=w184) -> ("PDU(1)"=w177:i32)  [unwired: 10 out]
                n101 = case shown="8" w177 {
                  tunnel: w183 -> [w186 w192]
                  tunnel: w182 -> [w185 w191]
                  tunnel: w181 -> [_ w190]
                  tunnel: [w186 w189] -> w180
                  tunnel: [w185 w188] -> w179
                  frame 0, Default {
                  }
                  frame 8 {
                    n102 = local write "状态"(FALSE ("状态")) -> ()
                    n103 = Enqueue Element(queue=w192, element=w190, error in (no error)=w191) -> (queue out=w189:refnum<queue>, error out=w188:errorcluster)  [unwired: 2 out]
                  }
                }
              }
              frame True {
              }
            }
          }
          frame "单体温度" {
            n104 = Not A Number/Path/Refnum?(number/path/refnum=w196) -> (NaN/Path/Refnum?=w195:bool)
            n105 = case shown="假" w195 {
              tunnel: w200 -> [w207 w218]
              tunnel: w199 -> [w206 w217]
              tunnel: [w205 w218] -> w198
              tunnel: [w204 w217] -> w197
              tunnel: w196 -> [w203 _]
              frame False {
                n106 = property class="Clust (严格)"(reference=w203) -> ("Value"=w201:T1)  [unwired: 1 in, 2 out]
                n107 = Unbundle By Name(w201) -> ("ID"=w208:u32)
                n108 = call "ID解析.vi"("ID"=w208) -> ("PDU(1)"=w202:i32)  [unwired: 10 out]
                n109 = case shown="10" w202 {
                  tunnel: w207 -> [w210 w216]
                  tunnel: w206 -> [w209 w215]
                  tunnel: w201 -> [_ w214]
                  tunnel: [w210 w213] -> w205
                  tunnel: [w209 w212] -> w204
                  frame 0, Default {
                  }
                  frame 16 {
                    n110 = local write "状态"(FALSE ("状态")) -> ()
                    n111 = Enqueue Element(queue=w216, element=w214, error in (no error)=w215) -> (queue out=w213:refnum<queue>, error out=w212:errorcluster)  [unwired: 2 out]
                  }
                }
              }
              frame True {
              }
            }
          }
          frame "单体内阻" {
            n112 = Not A Number/Path/Refnum?(number/path/refnum=w220) -> (NaN/Path/Refnum?=w219:bool)
            n113 = case shown="假" w219 {
              tunnel: w224 -> [w231 w242]
              tunnel: w223 -> [w230 w241]
              tunnel: [w228 w242] -> w222
              tunnel: [w227 w241] -> w221
              tunnel: w220 -> [w226 _]
              frame False {
                n114 = property class="Clust (严格)"(reference=w226) -> ("Value"=w229:T1)  [unwired: 1 in, 2 out]
                n115 = Unbundle By Name(w229) -> ("ID"=w232:u32)
                n116 = call "ID解析.vi"("ID"=w232) -> ("PDU(1)"=w225:i32)  [unwired: 10 out]
                n117 = case shown="C" w225 {
                  tunnel: w231 -> [w234 w240]
                  tunnel: w230 -> [w233 w239]
                  tunnel: w229 -> [_ w238]
                  tunnel: [w234 w237] -> w228
                  tunnel: [w233 w236] -> w227
                  frame 0, Default {
                  }
                  frame 12 {
                    n118 = local write "状态"(FALSE ("状态")) -> ()
                    n119 = Enqueue Element(queue=w240, element=w238, error in (no error)=w239) -> (queue out=w237:refnum<queue>, error out=w236:errorcluster)  [unwired: 2 out]
                  }
                }
              }
              frame True {
              }
            }
          }
          frame "单体SOC" {
            n120 = Not A Number/Path/Refnum?(number/path/refnum=w244) -> (NaN/Path/Refnum?=w243:bool)
            n121 = case shown="假" w243 {
              tunnel: w248 -> [w255 w266]
              tunnel: w247 -> [w254 w265]
              tunnel: [w252 w266] -> w246
              tunnel: [w251 w265] -> w245
              tunnel: w244 -> [w250 _]
              frame False {
                n122 = property class="Clust (严格)"(reference=w250) -> ("Value"=w253:T1)  [unwired: 1 in, 2 out]
                n123 = Unbundle By Name(w253) -> ("ID"=w256:u32)
                n124 = call "ID解析.vi"("ID"=w256) -> ("PDU(1)"=w249:i32)  [unwired: 10 out]
                n125 = case shown="14" w249 {
                  tunnel: w255 -> [w258 w264]
                  tunnel: w254 -> [w257 w263]
                  tunnel: w253 -> [_ w262]
                  tunnel: [w258 w261] -> w252
                  tunnel: [w257 w260] -> w251
                  frame 0, Default {
                  }
                  frame 20 {
                    n126 = local write "状态"(FALSE ("状态")) -> ()
                    n127 = Enqueue Element(queue=w264, element=w262, error in (no error)=w263) -> (queue out=w261:refnum<queue>, error out=w260:errorcluster)  [unwired: 2 out]
                  }
                }
              }
              frame True {
              }
            }
          }
        }
      }
      n128 = while {
        tunnel: w156 -> [w160]
        tunnel: w155 -> [w159]
        stop <- w161 stop-if-true
        n129 = Dequeue Element(queue=w160, error in (no error)=w159) -> (element=w158:T1, error out=w161:errorcluster)  [unwired: 3 out]
        n130 = case shown="无错误" w161 {
          tunnel: w158 -> [w162 _]
          frame No Error {
            n131 = local write "状态"(TRUE ("状态")) -> ()
            "VCI_Receive 2" <- w162
          }
          frame Error {
          }
        }
      }
      n132 = Release Queue(queue=w154, force destroy? (F)=TRUE ("强制销毁？(F)"), error in (no error)=w153) -> (error out=w152:errorcluster)  [unwired: 2 out]
      n133 = call <vilib>:"Clear Errors.vi"("error in (no error)"=w152) -> ()  [unwired: 7 out]
    }
    frame Enabled {
    }
  }
  n134 = while {
    shift-right: [w270] -> _
    shift-left: w1 -> [w269]
    shift-left: w1 -> [w268]
    stop <- w271 stop-if-true
    n135 = event shown="[1] \"刷新\": 值改变" {
      selector: _ -> [_ _ _ _]
      dyn-events: _ -> [_ _ _ _]
      timeout: 100 -> [_ _ _ _]
      tunnel: [_ _ w462 w468] -> w271
      tunnel: [w276 _ _ _] -> w270
      tunnel: w269 -> [w275 _ _ _]
      tunnel: w268 -> [w274 _ _ _]
      event Timeout {
        n136 = event-data() -> ()  [unwired: 3 out]
        n137 = local read "选项卡控件"() -> (w278:enum32{"单体电压", "单体温度", "单体内阻", "单体SOC"})
        n138 = local read "主界面选项"() -> (w288:T3)
        n139 = case shown="\"单体电压\", 默认" w278 {
          frame "单体电压", Default {
            n140 = control-ref of="单选选项2 3"() -> (w290:refnum<vi>)
            n141 = control-ref of="单选选项2 2"() -> (w291:refnum<vi>)
            n142 = control-ref of="单选选项2"() -> (w292:refnum<vi>)
            n143 = control-ref of="单选选项1"() -> (w289:refnum<vi>)
            n144 = local read "故障信息选择按键 2"() -> (w293:enum32{"单选选项2", "单选选项2 2", "单选选项2 3", "单选选项1"})
            n145 = Build Array(w292, w291, w290, w289) -> (w298:refnum<vi>[])
            n146 = case shown="\"单选选项2\"" w293 {
              selector: w293 -> [w305 w310 w315 w320]
              tunnel: [w304 w309 w314 w319] -> w295
              tunnel: [w303 w308 w313 w318] -> w297
              tunnel: w298 -> [w306 w311 w316 w321]
              tunnel: [enum32{"1-96", "97-192", "193-288", "289-300"}."1-96" ("电压选择") enum32{"1-96", "97-192", "193-288", "289-300"}."289-300" ("电压选择") enum32{"1-96", "97-192", "193-288", "289-300"}."193-288" ("电压选择") enum32{"1-96", "97-192", "193-288", "289-300"}."97-192" ("电压选择")] -> w294
              frame "单选选项1", Default {
                n147 = Delete From Array(array=w306, index=w305) -> (deleted portion=w303:refnum<vi>, array with subset deleted=w304:refnum<vi>[])  [unwired: 1 in]
              }
              frame "单选选项2 3" {
                n148 = Delete From Array(array=w311, index=w310) -> (deleted portion=w308:refnum<vi>, array with subset deleted=w309:refnum<vi>[])  [unwired: 1 in]
              }
              frame "单选选项2 2" {
                n149 = Delete From Array(array=w316, index=w315) -> (deleted portion=w313:refnum<vi>, array with subset deleted=w314:refnum<vi>[])  [unwired: 1 in]
              }
              frame "单选选项2" {
                n150 = Delete From Array(array=w321, index=w320) -> (deleted portion=w318:refnum<vi>, array with subset deleted=w319:refnum<vi>[])  [unwired: 1 in]
              }
            }
            n151 = local write "电压选择"(w294) -> ()
            n152 = for {
              tunnel: u32 87470 -> [w301]
              tunnel: w295 -> [w300] mode=indexing
              n153 = property class="Bool (严格)"(reference=w300, "BoolText.TextColor"=w301) -> ()  [unwired: 1 in, 2 out]
            }
            n154 = property class="Bool (严格)"(reference=w297, "BoolText.TextColor"=u32 16777215) -> ()  [unwired: 1 in, 2 out]
          }
          frame "单体温度" {
            n155 = control-ref of="单选选项1"() -> (w326:refnum<vi>)
            n156 = control-ref of="单选选项2"() -> (w324:refnum<vi>)
            n157 = control-ref of="单选选项2 3"() -> (w327:refnum<vi>)
            n158 = control-ref of="单选选项2 2"() -> (w325:refnum<vi>)
            n159 = local read "故障信息选择按键 3"() -> (w323:enum32{"单选选项2", "单选选项2 2", "单选选项2 3", "单选选项1"})
            n160 = Build Array(w324, w325, w327, w326) -> (w331:refnum<vi>[])
            n161 = case shown="\"单选选项2\"" w323 {
              selector: w323 -> [w338 w343 w348 w353]
              tunnel: [w337 w342 w347 w352] -> w328
              tunnel: [w336 w341 w346 w351] -> w330
              tunnel: w331 -> [w339 w344 w349 w354]
              tunnel: [enum32{"1-96", "97-192", "193-288", "289-300"}."1-96" ("电压选择") enum32{"1-96", "97-192", "193-288", "289-300"}."289-300" ("电压选择") enum32{"1-96", "97-192", "193-288", "289-300"}."193-288" ("电压选择") enum32{"1-96", "97-192", "193-288", "289-300"}."97-192" ("电压选择")] -> w322
              frame "单选选项1", Default {
                n162 = Delete From Array(array=w339, index=w338) -> (deleted portion=w336:refnum<vi>, array with subset deleted=w337:refnum<vi>[])  [unwired: 1 in]
              }
              frame "单选选项2 3" {
                n163 = Delete From Array(array=w344, index=w343) -> (deleted portion=w341:refnum<vi>, array with subset deleted=w342:refnum<vi>[])  [unwired: 1 in]
              }
              frame "单选选项2 2" {
                n164 = Delete From Array(array=w349, index=w348) -> (deleted portion=w346:refnum<vi>, array with subset deleted=w347:refnum<vi>[])  [unwired: 1 in]
              }
              frame "单选选项2" {
                n165 = Delete From Array(array=w354, index=w353) -> (deleted portion=w351:refnum<vi>, array with subset deleted=w352:refnum<vi>[])  [unwired: 1 in]
              }
            }
            n166 = local write "电压选择 2"(w322) -> ()
            n167 = for {
              tunnel: u32 87470 -> [w334]
              tunnel: w328 -> [w333] mode=indexing
              n168 = property class="Bool (严格)"(reference=w333, "BoolText.TextColor"=w334) -> ()  [unwired: 1 in, 2 out]
            }
            n169 = property class="Bool (严格)"(reference=w330, "BoolText.TextColor"=u32 16777215) -> ()  [unwired: 1 in, 2 out]
          }
          frame "单体内阻" {
            n170 = control-ref of="单选选项2 3"() -> (w360:refnum<vi>)
            n171 = control-ref of="单选选项2"() -> (w357:refnum<vi>)
            n172 = control-ref of="单选选项2 2"() -> (w358:refnum<vi>)
            n173 = control-ref of="单选选项1"() -> (w359:refnum<vi>)
            n174 = local read "故障信息选择按键 4"() -> (w356:enum32{"单选选项2", "单选选项2 2", "单选选项2 3", "单选选项1"})
            n175 = Build Array(w357, w358, w360, w359) -> (w364:refnum<vi>[])
            n176 = case shown="\"单选选项2\"" w356 {
              selector: w356 -> [w371 w376 w381 w386]
              tunnel: [w370 w375 w380 w385] -> w361
              tunnel: [w369 w374 w379 w384] -> w363
              tunnel: w364 -> [w372 w377 w382 w387]
              tunnel: [enum32{"1-96", "97-192", "193-288", "289-300"}."1-96" ("电压选择") enum32{"1-96", "97-192", "193-288", "289-300"}."289-300" ("电压选择") enum32{"1-96", "97-192", "193-288", "289-300"}."193-288" ("电压选择") enum32{"1-96", "97-192", "193-288", "289-300"}."97-192" ("电压选择")] -> w355
              frame "单选选项1", Default {
                n177 = Delete From Array(array=w372, index=w371) -> (deleted portion=w369:refnum<vi>, array with subset deleted=w370:refnum<vi>[])  [unwired: 1 in]
              }
              frame "单选选项2 3" {
                n178 = Delete From Array(array=w377, index=w376) -> (deleted portion=w374:refnum<vi>, array with subset deleted=w375:refnum<vi>[])  [unwired: 1 in]
              }
              frame "单选选项2 2" {
                n179 = Delete From Array(array=w382, index=w381) -> (deleted portion=w379:refnum<vi>, array with subset deleted=w380:refnum<vi>[])  [unwired: 1 in]
              }
              frame "单选选项2" {
                n180 = Delete From Array(array=w387, index=w386) -> (deleted portion=w384:refnum<vi>, array with subset deleted=w385:refnum<vi>[])  [unwired: 1 in]
              }
            }
            n181 = local write "电压选择 3"(w355) -> ()
            n182 = for {
              tunnel: u32 87470 -> [w367]
              tunnel: w361 -> [w366] mode=indexing
              n183 = property class="Bool (严格)"(reference=w366, "BoolText.TextColor"=w367) -> ()  [unwired: 1 in, 2 out]
            }
            n184 = property class="Bool (严格)"(reference=w363, "BoolText.TextColor"=u32 16777215) -> ()  [unwired: 1 in, 2 out]
          }
          frame "单体SOC" {
            n185 = control-ref of="单选选项1"() -> (w393:refnum<vi>)
            n186 = control-ref of="单选选项2 2"() -> (w391:refnum<vi>)
            n187 = control-ref of="单选选项2 3"() -> (w392:refnum<vi>)
            n188 = control-ref of="单选选项2"() -> (w390:refnum<vi>)
            n189 = local read "故障信息选择按键 5"() -> (w389:enum32{"单选选项2", "单选选项2 2", "单选选项2 3", "单选选项1"})
            n190 = Build Array(w390, w391, w392, w393) -> (w397:refnum<vi>[])
            n191 = case shown="\"单选选项2\"" w389 {
              selector: w389 -> [w404 w409 w414 w419]
              tunnel: [w403 w408 w413 w418] -> w394
              tunnel: [w402 w407 w412 w417] -> w396
              tunnel: w397 -> [w405 w410 w415 w420]
              tunnel: [enum32{"1-96", "97-192", "193-288", "289-300"}."1-96" ("电压选择") enum32{"1-96", "97-192", "193-288", "289-300"}."289-300" ("电压选择") enum32{"1-96", "97-192", "193-288", "289-300"}."193-288" ("电压选择") enum32{"1-96", "97-192", "193-288", "289-300"}."97-192" ("电压选择")] -> w388
              frame "单选选项1", Default {
                n192 = Delete From Array(array=w405, index=w404) -> (deleted portion=w402:refnum<vi>, array with subset deleted=w403:refnum<vi>[])  [unwired: 1 in]
              }
              frame "单选选项2 3" {
                n193 = Delete From Array(array=w410, index=w409) -> (deleted portion=w407:refnum<vi>, array with subset deleted=w408:refnum<vi>[])  [unwired: 1 in]
              }
              frame "单选选项2 2" {
                n194 = Delete From Array(array=w415, index=w414) -> (deleted portion=w412:refnum<vi>, array with subset deleted=w413:refnum<vi>[])  [unwired: 1 in]
              }
              frame "单选选项2" {
                n195 = Delete From Array(array=w420, index=w419) -> (deleted portion=w417:refnum<vi>, array with subset deleted=w418:refnum<vi>[])  [unwired: 1 in]
              }
            }
            n196 = local write "电压选择 4"(w388) -> ()
            n197 = for {
              tunnel: u32 87470 -> [w400]
              tunnel: w394 -> [w399] mode=indexing
              n198 = property class="Bool (严格)"(reference=w399, "BoolText.TextColor"=w400) -> ()  [unwired: 1 in, 2 out]
            }
            n199 = property class="Bool (严格)"(reference=w396, "BoolText.TextColor"=u32 16777215) -> ()  [unwired: 1 in, 2 out]
          }
        }
        n200 = Not Equal?(x=w275, y=w274) -> (x != y?=→"状态":bool)
        n201 = control-ref of="单选选项2 5"() -> (w282:refnum<vi>)
        n202 = control-ref of="单选选项2 6"() -> (w281:refnum<vi>)
        n203 = control-ref of="单选选项2 7"() -> (w280:refnum<vi>)
        n204 = control-ref of="单选选项2 8"() -> (w279:refnum<vi>)
        n205 = Build Array(w282, w281, w280, w279) -> (w283:refnum<vi>[])
        n206 = case shown="\"单选选项2 8\"" w288 {
          selector: w288 -> [w427 w432 w437 w442]
          tunnel: [w426 w431 w436 w441] -> w285
          tunnel: [w425 w430 w435 w440] -> w284
          tunnel: w283 -> [w424 w429 w434 w439]
          tunnel: [enum32{"单体电压", "单体温度", "单体内阻", "单体SOC"}."单体电压" ("选项卡控件") enum32{"单体电压", "单体温度", "单体内阻", "单体SOC"}."单体温度" ("选项卡控件") enum32{"单体电压", "单体温度", "单体内阻", "单体SOC"}."单体内阻" ("选项卡控件") enum32{"单体电压", "单体温度", "单体内阻", "单体SOC"}."单体SOC" ("选项卡控件")] -> w277
          frame "单选选项2 5" {
            n207 = Delete From Array(array=w424, index=w427) -> (deleted portion=w425:refnum<vi>, array with subset deleted=w426:refnum<vi>[])  [unwired: 1 in]
          }
          frame "单选选项2 6" {
            n208 = Delete From Array(array=w429, index=w432) -> (deleted portion=w430:refnum<vi>, array with subset deleted=w431:refnum<vi>[])  [unwired: 1 in]
          }
          frame "单选选项2 7" {
            n209 = Delete From Array(array=w434, index=w437) -> (deleted portion=w435:refnum<vi>, array with subset deleted=w436:refnum<vi>[])  [unwired: 1 in]
          }
          frame "单选选项2 8" {
            n210 = Delete From Array(array=w439, index=w442) -> (deleted portion=w440:refnum<vi>, array with subset deleted=w441:refnum<vi>[])  [unwired: 1 in]
          }
        }
        n211 = global read "EV05全局变量1.vi" "life"() -> (w276:dbl)
        "Life:" <- w276
        n212 = for {
          tunnel: w285 -> [w422] mode=indexing
          tunnel: u32 16777215 -> [w421]
          n213 = property class="Bool (严格)"(reference=w422, "BoolText.TextColor"=w421) -> ()  [unwired: 1 in, 2 out]
        }
        n214 = property class="Bool (严格)"(reference=w284, "BoolText.TextColor"=u32 8977151) -> ()  [unwired: 1 in, 2 out]
        n215 = local write "选项卡控件"(w277) -> ()
      }
      event "刷新": Value Change {
        n216 = event-data() -> ("NewVal"=w443:bool)  [unwired: 6 out]
        n217 = case shown="真" w443 {
          frame False {
          }
          frame True {
            n218 = local read "选项卡控件"() -> (w445:enum32{"单体电压", "单体温度", "单体内阻", "单体SOC"})
            n219 = case shown="\"单体电压\", 默认" w445 {
              frame "单体电压", Default {
                n220 = Initialize Array(0.0 ("(hi.lo)"), 300 ("维数大小")) -> (w447:dbl[])
                n221 = Initialize Array(0 ("(hi.lo)"), 300 ("维数大小")) -> (w446:i32[])
                n222 = global write "单体信息全局.vi" "SOC位置"(w446) -> ()
                n223 = global write "单体信息全局.vi" "数据"(w447) -> ()
                n224 = global write "单体信息全局.vi" "充电均衡"(w447) -> ()
                n225 = global write "单体信息全局.vi" "放电均衡"(w447) -> ()
                n226 = global write "单体信息全局.vi" "位置"(w446) -> ()
                n227 = local write "1 5"(T7 {"第289串"=0.0, "第290串"=0.0, "第291串"=0.0, "第292串"=0.0, "第293串"=0.0, "第294串"=0.0, "第295串"=0.0, "第296串"=0.0, "第297串"=0.0, "第298串"=0.0, "第299串"=0.0, "第300串"=0.0, "第一串 2"=0.0, "第一串 4"=0.0, "第一串 6"=0.0, "第一串 8"=0.0, "第一串 10"=0.0, "第一串 12"=0.0, "第一串 14"=0.0, "第一串 16"=0.0, "第一串 18"=0.0, "第一串 20"=0.0, "第一串 22"=0.0, "第一串 24"=0.0} ("1 5")) -> ()
              }
              frame "单体温度" {
                w460 = T13 {"1 3"={"第13串"=0.0, "第14串"=0.0, "第15串"=0.0, "第16串"=0.0, "第17串"=0.0, "第18串"=0.0, "第19串"=0.0, "第20串"=0.0, "第21串"=0.0, "第22串"=0.0, "第23串"=0.0, "第24串"=0.0, "第一串 2"=0.0, "第一串 4"=0.0, "第一串 6"=0.0, "第一串 8"=0.0, "第一串 10"=0.0, "第一串 12"=0.0, "第一串 14"=0.0, "第一串 16"=0.0, "第一串 18"=0.0, "第一串 20"=0.0, "第一串 22"=0.0, "第一串 24"=0.0}, "1 4"={"第25串"=0.0, "第26串"=0.0, "第27串"=0.0, "第28串"=0.0, "第29串"=0.0, "第30串"=0.0, "第31串"=0.0, "第32串"=0.0, "第33串"=0.0, "第34串"=0.0, "第35串"=0.0, "第36串"=0.0, "第一串 2"=0.0, "第一串 4"=0.0, "第一串 6"=0.0, "第一串 8"=0.0, "第一串 10"=0.0, "第一串 12"=0.0, "第一串 14"=0.0, "第一串 16"=0.0, "第一串 18"=0.0, "第一串 20"=0.0, "第一串 22"=0.0, "第一串 24"=0.0}, "1 6"={"第37串"=0.0, "第38串"=0.0, "第39串"=0.0, "第40串"=0.0, "第41串"=0.0, "第42串"=0.0, "第43串"=0.0, "第44串"=0.0, "第45串"=0.0, "第46串"=0.0, "第47串"=0.0, "第48串"=0.0, "第一串 2"=0.0, "第一串 4"=0.0, "第一串 6"=0.0, "第一串 8"=0.0, "第一串 10"=0.0, "第一串 12"=0.0, "第一串 14"=0.0, "第一串 16"=0.0, "第一串 18"=0.0, "第一串 20"=0.0, "第一串 22"=0.0, "第一串 24"=0.0}, "1 7"={"第49串"=0.0, "第50串"=0.0, "第51串"=0.0, "第52串"=0.0, "第53串"=0.0, "第54串"=0.0, "第55串"=0.0, "第56串"=0.0, "第57串"=0.0, "第58串"=0.0, "第59串"=0.0, "第60串"=0.0, "第一串 2"=0.0, "第一串 4"=0.0, "第一串 6"=0.0, "第一串 8"=0.0, "第一串 10"=0.0, "第一串 12"=0.0, "第一串 14"=0.0, "第一串 16"=0.0, "第一串 18"=0.0, "第一串 20"=0.0, "第一串 22"=0.0, "第一串 24"=0.0}, "1 8"={"第61串"=0.0, "第62串"=0.0, "第63串"=0.0, "第64串"=0.0, "第65串"=0.0, "第66串"=0.0, "第67串"=0.0, "第68串"=0.0, "第69串"=0.0, "第70串"=0.0, "第71串"=0.0, "第72串"=0.0, "第一串 2"=0.0, "第一串 4"=0.0, "第一串 6"=0.0, "第一串 8"=0.0, "第一串 10"=0.0, "第一串 12"=0.0, "第一串 14"=0.0, "第一串 16"=0.0, "第一串 18"=0.0, "第一串 20"=0.0, "第一串 22"=0.0, "第一串 24"=0.0}, "1 9"={"第73串"=0.0, "第74串"=0.0, "第75串"=0.0, "第76串"=0.0, "第77串"=0.0, "第78串"=0.0, "第79串"=0.0, "第80串"=0.0, "第81串"=0.0, "第82串"=0.0, "第83串"=0.0, "第84串"=0.0, "第一串 2"=0.0, "第一串 4"=0.0, "第一串 6"=0.0, "第一串 8"=0.0, "第一串 10"=0.0, "第一串 12"=0.0, "第一串 14"=0.0, "第一串 16"=0.0, "第一串 18"=0.0, "第一串 20"=0.0, "第一串 22"=0.0, "第一串 24"=0.0}, "1 10"={"第85串"=0.0, "第86串"=0.0, "第87串"=0.0, "第88串"=0.0, "第89串"=0.0, "第90串"=0.0, "第91串"=0.0, "第92串"=0.0, "第93串"=0.0, "第94串"=0.0, "第95串"=0.0, "第96串"=0.0, "第一串 2"=0.0, "第一串 4"=0.0, "第一串 6"=0.0, "第一串 8"=0.0, "第一串 10"=0.0, "第一串 12"=0.0, "第一串 14"=0.0, "第一串 16"=0.0, "第一串 18"=0.0, "第一串 20"=0.0, "第一串 22"=0.0, "第一串 24"=0.0}, "1 102"={"第1串"=0.0, "第2串"=0.0, "第3串"=0.0, "第4串"=0.0, "第5串"=0.0, "第6串"=0.0, "第7串"=0.0, "第8串"=0.0, "第9串"=0.0, "第10串"=0.0, "第11串"=0.0, "第12串"=0.0, "第一串 2"=0.0, "第一串 4"=0.0, "第一串 6"=0.0, "第一串 8"=0.0, "第一串 10"=0.0, "第一串 12"=0.0, "第一串 14"=0.0, "第一串 16"=0.0, "第一串 18"=0.0, "第一串 20"=0.0, "第一串 22"=0.0, "第一串 24"=0.0}} ("1 108")
                n228 = Initialize Array(0.0 ("(hi.lo)"), 300 ("维数大小")) -> (w456:dbl[])
                n229 = Initialize Array(0 ("(hi.lo)"), 300 ("维数大小")) -> (w453:i32[])
                n230 = global write "单体信息全局.vi" "数据 2"(w456) -> ()
                n231 = global write "单体信息全局.vi" "位置 2"(w453) -> ()
                n232 = local write "1 6"(T7 {"第289串"=0.0, "第290串"=0.0, "第291串"=0.0, "第292串"=0.0, "第293串"=0.0, "第294串"=0.0, "第295串"=0.0, "第296串"=0.0, "第297串"=0.0, "第298串"=0.0, "第299串"=0.0, "第300串"=0.0, "第一串 2"=0.0, "第一串 4"=0.0, "第一串 6"=0.0, "第一串 8"=0.0, "第一串 10"=0.0, "第一串 12"=0.0, "第一串 14"=0.0, "第一串 16"=0.0, "第一串 18"=0.0, "第一串 20"=0.0, "第一串 22"=0.0, "第一串 24"=0.0} ("1 5")) -> ()
                n233 = local write "4"(w460) -> ()
                n234 = local write "5"(w460) -> ()
                n235 = local write "6"(w460) -> ()
              }
            }
            n236 = local write "213"(TRUE ("213")) -> ()
          }
        }
      }
      event "停止": Value Change {
        n237 = event-data() -> ("NewVal"=w462:bool)  [unwired: 6 out]
        n238 = disable-structure shown="启用" {
          disable-tunnel: w462 -> [_ w467]
          frame Enabled {
            n239 = property class="VI"("FP.State"=T14."Hidden" ("前面板窗口:状态")) -> (reference out=w464:refnum<vi>, error out=w463:errorcluster)  [unwired: 2 in]
            n240 = property class="VI"(reference=w464, error in=w463, "Front Panel.Open"=FALSE ("前面板窗口:打开")) -> ()  [unwired: 2 out]
          }
          frame Disabled {
            n241 = Stop(stop? (T)=w467) -> ()
          }
        }
        n242 = local write "停止"(TRUE ("停止")) -> ()
      }
      event Panel Close? {
        w468 = TRUE ("停止")
        n243 = event-data() -> ()  [unwired: 5 out]
        n244 = disable-structure shown="启用" {
          disable-tunnel: w468 -> [_ w474]
          frame Enabled {
            n245 = property class="VI"("FP.State"=T14."Hidden" ("前面板窗口:状态")) -> (reference out=w471:refnum<vi>, error out=w470:errorcluster)  [unwired: 2 in]
            n246 = property class="VI"(reference=w471, error in=w470, "Front Panel.Open"=FALSE ("前面板窗口:打开")) -> ()  [unwired: 2 out]
          }
          frame Disabled {
            n247 = Stop(stop? (T)=w474) -> ()
          }
        }
        n248 = local write "停止"(w468) -> ()
        n249 = event-data("Discard?"=FALSE ("放弃？")) -> ()  [unwired: 1 in, 1 out]
      }
    }
    n250 = local write "状态"(FALSE ("状态")) -> ()
  }
  n251 = while {
    stop <- w475 stop-if-true
    n252 = local read "停止"() -> (w475:bool)
    n253 = local read "选项卡控件"() -> (w477:enum32{"单体电压", "单体温度", "单体内阻", "单体SOC"})
    n254 = Wait Until Next ms Multiple(millisecond multiple=u32 500 ("毫秒倍数")) -> ()  [unwired: 1 out]
    n255 = case shown="\"单体温度\"" w477 {
      frame "单体电压", Default {
        w487 = 0.0 ("新元素/子数组")
        n256 = global read "从板全局变量.vi" "电池节数"() -> (w484:u8[])
        n257 = global read "单体信息全局.vi" "单体数据"() -> (w486:dbl[][])
        n258 = for {
          tunnel: w484 -> [w618] mode=indexing
          tunnel: w486 -> [w621]
          shift-right: [w616] -> w480
          shift-left: dbl[] [] -> [w617]
          tunnel: w484 -> [w615]
          shift-right: [w613] -> w482
          shift-left: u16[] [] -> [w614]
          i -> [w620]
          n259 = Greater Than 0?(x=w618) -> (x > 0?=w619:bool)
          n260 = case shown="真" w619 {
            tunnel: w621 -> [_ w637]
            tunnel: w620 -> [_ w626]
            tunnel: w618 -> [_ w625]
            tunnel: w617 -> [w623 w634]
            tunnel: [w623 w635] -> w616
            tunnel: w615 -> [_ w632]
            tunnel: w614 -> [w622 w629]
            tunnel: [w622 w628] -> w613
            frame False {
            }
            frame True {
              n261 = Index Array(array=w637, index (row)=w626) -> (element=w636:dbl[])  [unwired: 1 in]
              n262 = Increment(x=w626) -> (x+1=w630:i32)
              n263 = Initialize Array(w630, w625) -> (w624:i32[])
              n264 = Array Subset(array=w636, length=w625) -> (w633:dbl[])  [unwired: 1 in]
              n265 = Array Subset(array=w632, length=w626) -> (w631:u8[])  [unwired: 1 in]
              n266 = Add Array Elements(numeric array=w631) -> (sum=w627:u8)
              n267 = Insert Into Array(array=w634, index=w627, new element=w633) -> (w635:dbl[])
              n268 = Insert Into Array(array=w629, index=w627, new element=w624) -> (w628:u16[])
            }
          }
        }
        n269 = global read "单体信息全局.vi" "位置"() -> (w493:i32[])
        n270 = global read "单体信息全局.vi" "充电均衡"() -> (w575:dbl[])
        n271 = global read "单体信息全局.vi" "放电均衡"() -> (w548:dbl[])
        n272 = global read "从板全局变量.vi" "均衡标记"() -> (w489:dbl[])
        n273 = global read "单体信息全局.vi" "均衡故障"() -> (w522:dbl[])
        n274 = Insert Into Array(array=w489, index=w487, new element=w487) -> (w488:dbl[])
        n275 = for {
          N: 25 -> [_]
          tunnel: w548 -> [w652]
          tunnel: [w648] -> w547 mode=indexing
          tunnel: w488 -> [w644]
          tunnel: w493 -> [w645]
          i -> [w647]
          w651 = 12 ("y")
          n276 = Multiply(x=w647, y=w651) -> (x*y=w646:i32)
          n277 = Array Subset(array=w652, index=w646, length=w651) -> (w650:dbl[])
          n278 = for {
            tunnel: w650 -> [w661] mode=indexing
            tunnel: [w662] -> w649 mode=indexing
            tunnel: w646 -> [w660]
            tunnel: w645 -> [w658]
            tunnel: w644 -> [w656]
            i -> [w659]
            n279 = Add(x=w660, y=w659) -> (x+y=w657:i32)
            n280 = Equal To 0?(x=w661) -> (x = 0?=w653:bool)
            n281 = Index Array(array=w658, index=w657) -> (element=w655:i32)
            n282 = Index Array(array=w656, index=w655) -> (element=w654:dbl)
            n283 = case shown="假" w653 {
              tunnel: w653 -> [w673 _]
              tunnel: [w672 u32 13816530] -> w662
              tunnel: w654 -> [w663 _]
              frame False {
                n284 = Equal To 0?(x=w663) -> (x = 0?=w671:bool)
                n285 = Equal To 0?(x=w663) -> (x = 0?=w667:bool)
                n286 = Select(t=u32 13816530, s=w671, f=u32 16776770) -> (s? t:f=w668:u32)
                n287 = Select(t=u32 16776770, s=w667, f=u32 6618880) -> (s? t:f=w665:u32)
                n288 = Select(t=w668, s=w673, f=w665) -> (s? t:f=w672:u32)
              }
              frame True {
              }
            }
          }
          n289 = Array To Cluster(array=w649) -> (cluster=w648:T15)
        }
        n290 = for {
          N: 25 -> [_]
          tunnel: w575 -> [w683]
          tunnel: [w679] -> w574 mode=indexing
          tunnel: w488 -> [w675]
          tunnel: w493 -> [w676]
          i -> [w678]
          w682 = 12 ("y")
          n291 = Multiply(x=w678, y=w682) -> (x*y=w677:i32)
          n292 = Array Subset(array=w683, index=w677, length=w682) -> (w681:dbl[])
          n293 = for {
            tunnel: w681 -> [w692] mode=indexing
            tunnel: [w693] -> w680 mode=indexing
            tunnel: w677 -> [w691]
            tunnel: w676 -> [w688]
            tunnel: w675 -> [w685]
            i -> [w690]
            n294 = Add(x=w691, y=w690) -> (x+y=w689:i32)
            n295 = Equal To 0?(x=w692) -> (x = 0?=w684:bool)
            n296 = Index Array(array=w688, index=w689) -> (element=w687:i32)
            n297 = Index Array(array=w685, index=w687) -> (element=w686:dbl)
            n298 = case shown="假" w684 {
              tunnel: w684 -> [w704 _]
              tunnel: [w703 u32 13816530] -> w693
              tunnel: w686 -> [w694 _]
              frame False {
                n299 = Equal To 0?(x=w694) -> (x = 0?=w702:bool)
                n300 = Equal To 0?(x=w694) -> (x = 0?=w699:bool)
                n301 = Select(t=u32 13816530, s=w699, f=u32 16776770) -> (s? t:f=w697:u32)
                n302 = Select(t=u32 16776770, s=w702, f=u32 16860) -> (s? t:f=w701:u32)
                n303 = Select(t=w697, s=w704, f=w701) -> (s? t:f=w703:u32)
              }
              frame True {
              }
            }
          }
          n304 = Array To Cluster(array=w680) -> (cluster=w679:T15)
        }
        n305 = Add Array Elements(numeric array=w484) -> (sum=w481:u8)
        n306 = global write "单体信息全局.vi" "PF"(w481) -> ()
        n307 = for {
          N: 25 -> [_]
          tunnel: w522 -> [w643]
          tunnel: [w639] -> w521 mode=indexing
          i -> [w642]
          w640 = 12 ("y")
          n308 = Multiply(x=w642, y=w640) -> (x*y=w641:i32)
          n309 = Array Subset(array=w643, index=w641, length=w640) -> (w638:dbl[])
          n310 = Array To Cluster(array=w638) -> (cluster=w639:T16)
        }
        n311 = Quotient & Remainder(x=w481, y=12) -> (x-y*floor(x/y)=w579:i32, floor(x/y)=w577:i32)
        n312 = Insert Into Array(array=w480, new element=dbl[] [0.0, 0.0, 0.0, 0.0, 0.0, 0.0, 0.0, 0.0, 8.0]) -> (w478:dbl[])  [unwired: 1 in]
        n313 = global write "单体信息全局.vi" "数据"(w478) -> ()
        n314 = Equal To 0?(x=w579) -> (x = 0?=w578:bool)
        n315 = Increment(x=w577) -> (x+1=w576:i32)
        n316 = Select(t=w577, s=w578, f=w576) -> (s? t:f=w492:i32)
        n317 = for {
          N: w492 -> [_]
          tunnel: w478 -> [w714]
          tunnel: w482 -> [w706]
          tunnel: [w707] -> w611 mode=indexing
          i -> [w713]
          w711 = 12 ("y")
          n318 = Multiply(x=w713, y=w711) -> (x*y=w712:i32)
          n319 = Array Subset(array=w706, index=w712, length=w711) -> (w709:u16[])
          n320 = Array Subset(array=w714, index=w712, length=w711) -> (w710:dbl[])
          n321 = Insert Into Array(array=w710, new element=w709) -> (w708:dbl[])  [unwired: 1 in]
          n322 = Array To Cluster(array=w708) -> (cluster=w707:T17)
        }
        n323 = Index Array(array=w521) -> (element #1=w520:T16, element #2=w519:T16, element #3=w518:T16, element #4=w517:T16, element #5=w516:T16, element #6=w515:T16, element #7=w514:T16, element #8=w513:T16, element #9=w512:T16, element #10=w511:T16, element #11=w510:T16, element #12=w509:T16, element #13=w508:T16, element #14=w507:T16, element #15=w506:T16, element #16=w505:T16, element #17=w504:T16, element #18=w503:T16, element #19=w502:T16, element #20=w501:T16, element #21=w500:T16, element #22=w499:T16, element #23=w498:T16, element #24=w497:T16, element #25=w496:T16)  [unwired: 25 in]
        n324 = Index Array(array=w547) -> (element #1=w546:T15, element #2=w545:T15, element #3=w544:T15, element #4=w543:T15, element #5=w542:T15, element #6=w541:T15, element #7=w540:T15, element #8=w539:T15, element #9=w538:T15, element #10=w537:T15, element #11=w536:T15, element #12=w535:T15, element #13=w534:T15, element #14=w533:T15, element #15=w532:T15, element #16=w531:T15, element #17=w530:T15, element #18=w529:T15, element #19=w528:T15, element #20=w527:T15, element #21=w526:T15, element #22=w525:T15, element #23=w524:T15, element #24=w523:T15, element #25=w495:T15)  [unwired: 25 in]
        n325 = Index Array(array=w574) -> (element #1=w573:T15, element #2=w572:T15, element #3=w571:T15, element #4=w570:T15, element #5=w569:T15, element #6=w568:T15, element #7=w567:T15, element #8=w566:T15, element #9=w565:T15, element #10=w564:T15, element #11=w563:T15, element #12=w562:T15, element #13=w561:T15, element #14=w560:T15, element #15=w559:T15, element #16=w558:T15, element #17=w557:T15, element #18=w556:T15, element #19=w555:T15, element #20=w554:T15, element #21=w553:T15, element #22=w552:T15, element #23=w551:T15, element #24=w550:T15, element #25=w549:T15)  [unwired: 25 in]
        n326 = local write "1 13"(w496) -> ()
        n327 = local write "放电均衡"(w495) -> ()
        n328 = local write "充电均衡"(w549) -> ()
        n329 = Index Array(array=w611) -> (element #1=w610:T17, element #2=w609:T17, element #3=w608:T17, element #4=w607:T17, element #5=w606:T17, element #6=w605:T17, element #7=w604:T17, element #8=w603:T17, element #9=w599:T17, element #10=w598:T17, element #11=w597:T17, element #12=w596:T17, element #13=w595:T17, element #14=w594:T17, element #15=w593:T17, element #16=w592:T17, element #17=w589:T17, element #18=w588:T17, element #19=w587:T17, element #20=w586:T17, element #21=w585:T17, element #22=w584:T17, element #23=w583:T17, element #24=w582:T17, element #25=w581:T17)  [unwired: 25 in]
        n330 = local read "1"() -> (w612:T4)
        n331 = local write "1 5"(w581) -> ()
        n332 = Bundle(cluster=w612, "1 102"=w610, "1 3"=w609, "1 4"=w608, "1 6"=w607, "1 7"=w606, "1 8"=w605, "1 9"=w604, "1 10"=w603, "1 12"=w573, "1 28"=w572, "1 25"=w571, "1 31"=w570, "1 16"=w569, "1 19"=w568, "1 22"=w567, "1 34"=w566, "1 11"=w546, "1 27"=w545, "1 24"=w544, "1 30"=w543, "1 15"=w542, "1 18"=w541, "1 21"=w540, "1 33"=w539, "1 13"=w520, "1 26"=w519, "1 23"=w518, "1 29"=w517, "1 14"=w516, "1 17"=w515, "1 20"=w514, "1 32"=w513) -> (w602:T4)
        n333 = local read "2"() -> (w601:T5)
        n334 = Bundle(cluster=w601, "1 26"=w599, "1 27"=w598, "1 28"=w597, "1 29"=w596, "1 30"=w595, "1 31"=w594, "1 32"=w593, "1 33"=w592, "1 16"=w565, "1 44"=w564, "1 36"=w563, "1 47"=w562, "1 19"=w561, "1 38"=w560, "1 41"=w559, "1 50"=w558, "1 15"=w538, "1 43"=w537, "1 35"=w536, "1 46"=w535, "1 18"=w534, "1 37"=w533, "1 40"=w532, "1 49"=w531, "1 14"=w512, "1 42"=w511, "1 34"=w510, "1 45"=w509, "1 17"=w508, "1 20"=w507, "1 39"=w506, "1 48"=w505) -> (w600:T5)
        n335 = local write "1"(w602) -> ()
        n336 = local write "2"(w600) -> ()
        n337 = local read "3"() -> (w590:T6)
        n338 = Bundle(cluster=w590, "1 18"=w589, "1 19"=w588, "1 20"=w587, "1 21"=w586, "1 22"=w585, "1 23"=w584, "1 24"=w583, "1 25"=w582, "1 12"=w557, "1 39"=w556, "1 28"=w555, "1 42"=w554, "1 16"=w553, "1 30"=w552, "1 33"=w551, "1 36"=w550, "1 11"=w530, "1 38"=w529, "1 27"=w528, "1 41"=w527, "1 15"=w526, "1 29"=w525, "1 32"=w524, "1 35"=w523, "1 13"=w504, "1 37"=w503, "1 26"=w502, "1 40"=w501, "1 14"=w500, "1 17"=w499, "1 31"=w498, "1 34"=w497) -> (w591:T6)
        n339 = local write "3"(w591) -> ()
      }
      frame "单体温度" {
        (unwired) 12 ("y")
        n340 = global read "从板全局变量.vi" "温度个数"() -> (w722:u8[])
        n341 = global read "单体信息全局.vi" "温度数据"() -> (w720:u8[][])
        n342 = Add Array Elements(numeric array=w722) -> (sum=w719:u8)
        n343 = Wait Until Next ms Multiple(millisecond multiple=u32 500 ("毫秒倍数")) -> ()  [unwired: 1 out]
        n344 = for {
          tunnel: w722 -> [w768] mode=indexing
          tunnel: w720 -> [w771]
          shift-right: [w766] -> w717
          shift-left: dbl[] [] -> [w767]
          tunnel: w722 -> [w765]
          shift-right: [w763] -> w718
          shift-left: u16[] [] -> [w764]
          i -> [w770]
          n345 = Greater Than 0?(x=w768) -> (x > 0?=w769:bool)
          n346 = case shown="真" w769 {
            tunnel: w771 -> [_ w787]
            tunnel: w770 -> [_ w776]
            tunnel: w768 -> [_ w775]
            tunnel: w767 -> [w773 w784]
            tunnel: [w773 w785] -> w766
            tunnel: w765 -> [_ w782]
            tunnel: w764 -> [w772 w779]
            tunnel: [w772 w778] -> w763
            frame False {
            }
            frame True {
              n347 = Index Array(array=w787, index (row)=w776) -> (element=w786:u8[])  [unwired: 1 in]
              n348 = Increment(x=w776) -> (x+1=w780:i32)
              n349 = Initialize Array(w780, w775) -> (w774:i32[])
              n350 = Array Subset(array=w786, length=w775) -> (w783:u8[])  [unwired: 1 in]
              n351 = Array Subset(array=w782, length=w776) -> (w781:u8[])  [unwired: 1 in]
              n352 = Add Array Elements(numeric array=w781) -> (sum=w777:u8)
              n353 = Insert Into Array(array=w784, index=w777, new element=w783) -> (w785:dbl[])
              n354 = Insert Into Array(array=w779, index=w777, new element=w774) -> (w778:u16[])
            }
          }
        }
        n355 = Quotient & Remainder(x=w719, y=12) -> (x-y*floor(x/y)=w729:i32, floor(x/y)=w727:i32)
        n356 = Equal To 0?(x=w729) -> (x = 0?=w728:bool)
        n357 = Increment(x=w727) -> (x+1=w726:i32)
        n358 = Select(t=w727, s=w728, f=w726) -> (s? t:f=w725:i32)
        n359 = Insert Into Array(array=w717, new element=dbl[] [0.0, 0.0, 0.0, 0.0, 0.0, 0.0, 0.0, 0.0, 0.0]) -> (w715:dbl[])  [unwired: 1 in]
        n360 = for {
          N: w725 -> [w791]
          tunnel: w715 -> [w799]
          tunnel: w718 -> [w792]
          tunnel: [w793] -> w761 mode=indexing
          i -> [w790]
          w797 = 12 ("y")
          n361 = Increment(x=w790) -> (x+1=w789:i32)
          n362 = Equal?(x=w791, y=w789) -> ()  [unwired: 1 out]
          n363 = Multiply(x=w790, y=w797) -> (x*y=w798:i32)
          n364 = Array Subset(array=w792, index=w798, length=w797) -> (w795:u16[])
          n365 = Array Subset(array=w799, index=w798, length=w797) -> (w796:dbl[])
          n366 = Insert Into Array(array=w796, index=12 ("索引"), new element=w795) -> (w794:dbl[])
          n367 = Array To Cluster(array=w794) -> (cluster=w793:T17)
        }
        n368 = global write "单体信息全局.vi" "数据 2"(w715) -> ()
        n369 = Index Array(array=w761) -> (element #1=w760:T17, element #2=w759:T17, element #3=w758:T17, element #4=w757:T17, element #5=w756:T17, element #6=w755:T17, element #7=w754:T17, element #8=w753:T17, element #9=w749:T17, element #10=w748:T17, element #11=w747:T17, element #12=w746:T17, element #13=w745:T17, element #14=w744:T17, element #15=w743:T17, element #16=w742:T17, element #17=w739:T17, element #18=w738:T17, element #19=w737:T17, element #20=w736:T17, element #21=w735:T17, element #22=w734:T17, element #23=w733:T17, element #24=w732:T17, element #25=w731:T17)  [unwired: 25 in]
        n370 = local read "6"() -> (w740:T12)
        n371 = local read "5"() -> (w751:T11)
        n372 = Bundle(cluster=w751, "1 26"=w749, "1 27"=w748, "1 28"=w747, "1 29"=w746, "1 30"=w745, "1 31"=w744, "1 32"=w743, "1 33"=w742) -> (w750:T11)
        n373 = Bundle(cluster=w740, "1 18"=w739, "1 19"=w738, "1 20"=w737, "1 21"=w736, "1 22"=w735, "1 23"=w734, "1 24"=w733, "1 25"=w732) -> (w741:T12)
        n374 = local write "1 6"(w731) -> ()
        n375 = local write "5"(w750) -> ()
        n376 = local read "4"() -> (w762:T10)
        n377 = local write "6"(w741) -> ()
        n378 = Bundle(cluster=w762, "1 102"=w760, "1 3"=w759, "1 4"=w758, "1 6"=w757, "1 7"=w756, "1 8"=w755, "1 9"=w754, "1 10"=w753) -> (w752:T10)
        n379 = local write "4"(w752) -> ()
      }
    }
    n380 = disable-structure shown="禁用" {
      frame Disabled {
        n381 = global read "单体信息全局.vi" "PF"() -> ()  [unwired: 1 out]
        n382 = global read "单体信息全局.vi" "数据"() -> ()  [unwired: 1 out]
      }
      frame Enabled {
      }
    }
  }
  n383 = disable-structure shown="启用" {
    frame Disabled {
      n384 = while {
        stop <- w801 stop-if-true
        n385 = local read "停止"() -> (w801:bool)
        n386 = Wait Until Next ms Multiple(millisecond multiple=u32 500 ("毫秒倍数")) -> ()  [unwired: 1 out]
        n387 = case shown="真" "213" {
          frame False {
          }
          frame True {
            n388 = local read "选项卡控件"() -> (w804:enum32{"单体电压", "单体温度", "单体内阻", "单体SOC"})
            n389 = local write "213"(FALSE ("213")) -> ()
            n390 = case shown="\"单体温度\"" w804 {
              frame "单体电压", Default {
                n391 = for {
                  N: 300 -> [_]
                  tunnel: [TRUE] -> w806 mode=indexing
                }
                n392 = for {
                  N: 16 -> [_]
                  tunnel: w806 -> [w813]
                  i -> [w814]
                  w811 = 12 ("y")
                  n393 = Multiply(x=w814, y=w811) -> (x*y=w812:i32)
                  n394 = Array Subset(array=w813, index=w812, length=w811) -> (w810:bool[])
                  n395 = case shown="0" w814 {
                    tunnel: w810 -> [w816 w826 w837 w848 w859 w870 w881 w892 w903 w914 w925 w936 w947 w958 w969 w980 _]
                    frame 0 {
                      n396 = control-ref of="1 102"() -> (w818:refnum<vi>)
                      n397 = property class="Clust (严格)"(reference=w818) -> ("Controls[]"=w817:refnum<vi>[])  [unwired: 1 in, 2 out]
                      n398 = for {
                        N: 12 -> [_]
                        tunnel: w817 -> [w824] mode=indexing
                        tunnel: w816 -> [w825]
                        i -> [w822]
                        n399 = Index Array(array=w825, index=w822) -> (element=w823:bool)
                        n400 = Select(t=0, s=w823, f=2) -> (s? t:f=w821:i32)
                        n401 = property class="Ctl"(reference=w824, "DisabledEnum"=w821) -> ()  [unwired: 1 in, 2 out]
                      }
                    }
                    frame 1 {
                      n402 = control-ref of="1 3"() -> (w829:refnum<vi>)
                      n403 = property class="Clust (严格)"(reference=w829) -> ("Controls[]"=w827:refnum<vi>[])  [unwired: 1 in, 2 out]
                      n404 = for {
                        N: 12 -> [_]
                        tunnel: w827 -> [w835] mode=indexing
                        tunnel: w826 -> [w836]
                        i -> [w833]
                        n405 = Index Array(array=w836, index=w833) -> (element=w834:bool)
                        n406 = Select(t=0, s=w834, f=2) -> (s? t:f=w832:i32)
                        n407 = property class="Ctl"(reference=w835, "DisabledEnum"=w832) -> ()  [unwired: 1 in, 2 out]
                      }
                    }
                    frame 2 {
                      n408 = control-ref of="1 4"() -> (w840:refnum<vi>)
                      n409 = property class="Clust (严格)"(reference=w840) -> ("Controls[]"=w838:refnum<vi>[])  [unwired: 1 in, 2 out]
                      n410 = for {
                        N: 12 -> [_]
                        tunnel: w838 -> [w846] mode=indexing
                        tunnel: w837 -> [w847]
                        i -> [w844]
                        n411 = Index Array(array=w847, index=w844) -> (element=w845:bool)
                        n412 = Select(t=0, s=w845, f=2) -> (s? t:f=w843:i32)
                        n413 = property class="Ctl"(reference=w846, "DisabledEnum"=w843) -> ()  [unwired: 1 in, 2 out]
                      }
                    }
                    frame 3 {
                      n414 = control-ref of="1 6"() -> (w851:refnum<vi>)
                      n415 = property class="Clust (严格)"(reference=w851) -> ("Controls[]"=w849:refnum<vi>[])  [unwired: 1 in, 2 out]
                      n416 = for {
                        N: 12 -> [_]
                        tunnel: w849 -> [w857] mode=indexing
                        tunnel: w848 -> [w858]
                        i -> [w855]
                        n417 = Index Array(array=w858, index=w855) -> (element=w856:bool)
                        n418 = Select(t=0, s=w856, f=2) -> (s? t:f=w854:i32)
                        n419 = property class="Ctl"(reference=w857, "DisabledEnum"=w854) -> ()  [unwired: 1 in, 2 out]
                      }
                    }
                    frame 4 {
                      n420 = control-ref of="1 7"() -> (w862:refnum<vi>)
                      n421 = property class="Clust (严格)"(reference=w862) -> ("Controls[]"=w860:refnum<vi>[])  [unwired: 1 in, 2 out]
                      n422 = for {
                        N: 12 -> [_]
                        tunnel: w860 -> [w868] mode=indexing
                        tunnel: w859 -> [w869]
                        i -> [w866]
                        n423 = Index Array(array=w869, index=w866) -> (element=w867:bool)
                        n424 = Select(t=0, s=w867, f=2) -> (s? t:f=w865:i32)
                        n425 = property class="Ctl"(reference=w868, "DisabledEnum"=w865) -> ()  [unwired: 1 in, 2 out]
                      }
                    }
                    frame 5 {
                      n426 = control-ref of="1 8"() -> (w873:refnum<vi>)
                      n427 = property class="Clust (严格)"(reference=w873) -> ("Controls[]"=w871:refnum<vi>[])  [unwired: 1 in, 2 out]
                      n428 = for {
                        N: 12 -> [_]
                        tunnel: w871 -> [w879] mode=indexing
                        tunnel: w870 -> [w880]
                        i -> [w877]
                        n429 = Index Array(array=w880, index=w877) -> (element=w878:bool)
                        n430 = Select(t=0, s=w878, f=2) -> (s? t:f=w876:i32)
                        n431 = property class="Ctl"(reference=w879, "DisabledEnum"=w876) -> ()  [unwired: 1 in, 2 out]
                      }
                    }
                    frame 6 {
                      n432 = control-ref of="1 9"() -> (w884:refnum<vi>)
                      n433 = property class="Clust (严格)"(reference=w884) -> ("Controls[]"=w882:refnum<vi>[])  [unwired: 1 in, 2 out]
                      n434 = for {
                        N: 12 -> [_]
                        tunnel: w882 -> [w890] mode=indexing
                        tunnel: w881 -> [w891]
                        i -> [w888]
                        n435 = Index Array(array=w891, index=w888) -> (element=w889:bool)
                        n436 = Select(t=0, s=w889, f=2) -> (s? t:f=w887:i32)
                        n437 = property class="Ctl"(reference=w890, "DisabledEnum"=w887) -> ()  [unwired: 1 in, 2 out]
                      }
                    }
                    frame 7 {
                      n438 = control-ref of="1 10"() -> (w895:refnum<vi>)
                      n439 = property class="Clust (严格)"(reference=w895) -> ("Controls[]"=w893:refnum<vi>[])  [unwired: 1 in, 2 out]
                      n440 = for {
                        N: 12 -> [_]
                        tunnel: w893 -> [w901] mode=indexing
                        tunnel: w892 -> [w902]
                        i -> [w899]
                        n441 = Index Array(array=w902, index=w899) -> (element=w900:bool)
                        n442 = Select(t=0, s=w900, f=2) -> (s? t:f=w898:i32)
                        n443 = property class="Ctl"(reference=w901, "DisabledEnum"=w898) -> ()  [unwired: 1 in, 2 out]
                      }
                    }
                    frame 8 {
                      n444 = control-ref of="1 26"() -> (w906:refnum<vi>)
                      n445 = property class="Clust (严格)"(reference=w906) -> ("Controls[]"=w904:refnum<vi>[])  [unwired: 1 in, 2 out]
                      n446 = for {
                        N: 12 -> [_]
                        tunnel: w904 -> [w912] mode=indexing
                        tunnel: w903 -> [w913]
                        i -> [w910]
                        n447 = Index Array(array=w913, index=w910) -> (element=w911:bool)
                        n448 = Select(t=0, s=w911, f=2) -> (s? t:f=w909:i32)
                        n449 = property class="Ctl"(reference=w912, "DisabledEnum"=w909) -> ()  [unwired: 1 in, 2 out]
                      }
                    }
                    frame 9 {
                      n450 = control-ref of="1 27"() -> (w917:refnum<vi>)
                      n451 = property class="Clust (严格)"(reference=w917) -> ("Controls[]"=w915:refnum<vi>[])  [unwired: 1 in, 2 out]
                      n452 = for {
                        N: 12 -> [_]
                        tunnel: w915 -> [w923] mode=indexing
                        tunnel: w914 -> [w924]
                        i -> [w921]
                        n453 = Index Array(array=w924, index=w921) -> (element=w922:bool)
                        n454 = Select(t=0, s=w922, f=2) -> (s? t:f=w920:i32)
                        n455 = property class="Ctl"(reference=w923, "DisabledEnum"=w920) -> ()  [unwired: 1 in, 2 out]
                      }
                    }
                    frame 10 {
                      n456 = control-ref of="1 28"() -> (w928:refnum<vi>)
                      n457 = property class="Clust (严格)"(reference=w928) -> ("Controls[]"=w926:refnum<vi>[])  [unwired: 1 in, 2 out]
                      n458 = for {
                        N: 12 -> [_]
                        tunnel: w926 -> [w934] mode=indexing
                        tunnel: w925 -> [w935]
                        i -> [w932]
                        n459 = Index Array(array=w935, index=w932) -> (element=w933:bool)
                        n460 = Select(t=0, s=w933, f=2) -> (s? t:f=w931:i32)
                        n461 = property class="Ctl"(reference=w934, "DisabledEnum"=w931) -> ()  [unwired: 1 in, 2 out]
                      }
                    }
                    frame 11 {
                      n462 = control-ref of="1 29"() -> (w939:refnum<vi>)
                      n463 = property class="Clust (严格)"(reference=w939) -> ("Controls[]"=w937:refnum<vi>[])  [unwired: 1 in, 2 out]
                      n464 = for {
                        N: 12 -> [_]
                        tunnel: w937 -> [w945] mode=indexing
                        tunnel: w936 -> [w946]
                        i -> [w943]
                        n465 = Index Array(array=w946, index=w943) -> (element=w944:bool)
                        n466 = Select(t=0, s=w944, f=2) -> (s? t:f=w942:i32)
                        n467 = property class="Ctl"(reference=w945, "DisabledEnum"=w942) -> ()  [unwired: 1 in, 2 out]
                      }
                    }
                    frame 12 {
                      n468 = control-ref of="1 30"() -> (w950:refnum<vi>)
                      n469 = property class="Clust (严格)"(reference=w950) -> ("Controls[]"=w948:refnum<vi>[])  [unwired: 1 in, 2 out]
                      n470 = for {
                        N: 12 -> [_]
                        tunnel: w948 -> [w956] mode=indexing
                        tunnel: w947 -> [w957]
                        i -> [w954]
                        n471 = Index Array(array=w957, index=w954) -> (element=w955:bool)
                        n472 = Select(t=0, s=w955, f=2) -> (s? t:f=w953:i32)
                        n473 = property class="Ctl"(reference=w956, "DisabledEnum"=w953) -> ()  [unwired: 1 in, 2 out]
                      }
                    }
                    frame 13 {
                      n474 = control-ref of="1 31"() -> (w961:refnum<vi>)
                      n475 = property class="Clust (严格)"(reference=w961) -> ("Controls[]"=w959:refnum<vi>[])  [unwired: 1 in, 2 out]
                      n476 = for {
                        N: 12 -> [_]
                        tunnel: w959 -> [w967] mode=indexing
                        tunnel: w958 -> [w968]
                        i -> [w965]
                        n477 = Index Array(array=w968, index=w965) -> (element=w966:bool)
                        n478 = Select(t=0, s=w966, f=2) -> (s? t:f=w964:i32)
                        n479 = property class="Ctl"(reference=w967, "DisabledEnum"=w964) -> ()  [unwired: 1 in, 2 out]
                      }
                    }
                    frame 14 {
                      n480 = control-ref of="1 32"() -> (w972:refnum<vi>)
                      n481 = property class="Clust (严格)"(reference=w972) -> ("Controls[]"=w970:refnum<vi>[])  [unwired: 1 in, 2 out]
                      n482 = for {
                        N: 12 -> [_]
                        tunnel: w970 -> [w978] mode=indexing
                        tunnel: w969 -> [w979]
                        i -> [w976]
                        n483 = Index Array(array=w979, index=w976) -> (element=w977:bool)
                        n484 = Select(t=0, s=w977, f=2) -> (s? t:f=w975:i32)
                        n485 = property class="Ctl"(reference=w978, "DisabledEnum"=w975) -> ()  [unwired: 1 in, 2 out]
                      }
                    }
                    frame 15 {
                      n486 = control-ref of="1 33"() -> (w983:refnum<vi>)
                      n487 = property class="Clust (严格)"(reference=w983) -> ("Controls[]"=w981:refnum<vi>[])  [unwired: 1 in, 2 out]
                      n488 = for {
                        N: 12 -> [_]
                        tunnel: w981 -> [w989] mode=indexing
                        tunnel: w980 -> [w990]
                        i -> [w987]
                        n489 = Index Array(array=w990, index=w987) -> (element=w988:bool)
                        n490 = Select(t=0, s=w988, f=2) -> (s? t:f=w986:i32)
                        n491 = property class="Ctl"(reference=w989, "DisabledEnum"=w986) -> ()  [unwired: 1 in, 2 out]
                      }
                    }
                    frame 99, Default {
                    }
                  }
                }
                n492 = for {
                  N: 9 -> [_]
                  tunnel: w806 -> [w996]
                  i -> [w997]
                  w994 = 12 ("y")
                  n493 = Add(x=16, y=w997) -> (x+y=w992:i32)
                  n494 = Multiply(x=w992, y=w994) -> (x*y=w995:i32)
                  n495 = Array Subset(array=w996, index=w995, length=w994) -> (w993:bool[])
                  n496 = case shown="8" w997 {
                    tunnel: w993 -> [w998 w1009 w1020 w1031 w1042 w1053 w1064 w1075 w1086 _]
                    frame 0 {
                      n497 = control-ref of="1 18"() -> (w1001:refnum<vi>)
                      n498 = property class="Clust (严格)"(reference=w1001) -> ("Controls[]"=w999:refnum<vi>[])  [unwired: 1 in, 2 out]
                      n499 = for {
                        N: 12 -> [_]
                        tunnel: w999 -> [w1007] mode=indexing
                        tunnel: w998 -> [w1008]
                        i -> [w1005]
                        n500 = Index Array(array=w1008, index=w1005) -> (element=w1006:bool)
                        n501 = Select(t=0, s=w1006, f=2) -> (s? t:f=w1004:i32)
                        n502 = property class="Ctl"(reference=w1007, "DisabledEnum"=w1004) -> ()  [unwired: 1 in, 2 out]
                      }
                    }
                    frame 1 {
                      n503 = control-ref of="1 19"() -> (w1012:refnum<vi>)
                      n504 = property class="Clust (严格)"(reference=w1012) -> ("Controls[]"=w1010:refnum<vi>[])  [unwired: 1 in, 2 out]
                      n505 = for {
                        N: 12 -> [_]
                        tunnel: w1010 -> [w1018] mode=indexing
                        tunnel: w1009 -> [w1019]
                        i -> [w1016]
                        n506 = Index Array(array=w1019, index=w1016) -> (element=w1017:bool)
                        n507 = Select(t=0, s=w1017, f=2) -> (s? t:f=w1015:i32)
                        n508 = property class="Ctl"(reference=w1018, "DisabledEnum"=w1015) -> ()  [unwired: 1 in, 2 out]
                      }
                    }
                    frame 2 {
                      n509 = control-ref of="1 20"() -> (w1023:refnum<vi>)
                      n510 = property class="Clust (严格)"(reference=w1023) -> ("Controls[]"=w1021:refnum<vi>[])  [unwired: 1 in, 2 out]
                      n511 = for {
                        N: 12 -> [_]
                        tunnel: w1021 -> [w1029] mode=indexing
                        tunnel: w1020 -> [w1030]
                        i -> [w1027]
                        n512 = Index Array(array=w1030, index=w1027) -> (element=w1028:bool)
                        n513 = Select(t=0, s=w1028, f=2) -> (s? t:f=w1026:i32)
                        n514 = property class="Ctl"(reference=w1029, "DisabledEnum"=w1026) -> ()  [unwired: 1 in, 2 out]
                      }
                    }
                    frame 3 {
                      n515 = control-ref of="1 21"() -> (w1034:refnum<vi>)
                      n516 = property class="Clust (严格)"(reference=w1034) -> ("Controls[]"=w1032:refnum<vi>[])  [unwired: 1 in, 2 out]
                      n517 = for {
                        N: 12 -> [_]
                        tunnel: w1032 -> [w1040] mode=indexing
                        tunnel: w1031 -> [w1041]
                        i -> [w1038]
                        n518 = Index Array(array=w1041, index=w1038) -> (element=w1039:bool)
                        n519 = Select(t=0, s=w1039, f=2) -> (s? t:f=w1037:i32)
                        n520 = property class="Ctl"(reference=w1040, "DisabledEnum"=w1037) -> ()  [unwired: 1 in, 2 out]
                      }
                    }
                    frame 4 {
                      n521 = control-ref of="1 22"() -> (w1045:refnum<vi>)
                      n522 = property class="Clust (严格)"(reference=w1045) -> ("Controls[]"=w1043:refnum<vi>[])  [unwired: 1 in, 2 out]
                      n523 = for {
                        N: 12 -> [_]
                        tunnel: w1043 -> [w1051] mode=indexing
                        tunnel: w1042 -> [w1052]
                        i -> [w1049]
                        n524 = Index Array(array=w1052, index=w1049) -> (element=w1050:bool)
                        n525 = Select(t=0, s=w1050, f=2) -> (s? t:f=w1048:i32)
                        n526 = property class="Ctl"(reference=w1051, "DisabledEnum"=w1048) -> ()  [unwired: 1 in, 2 out]
                      }
                    }
                    frame 5 {
                      n527 = control-ref of="1 23"() -> (w1056:refnum<vi>)
                      n528 = property class="Clust (严格)"(reference=w1056) -> ("Controls[]"=w1054:refnum<vi>[])  [unwired: 1 in, 2 out]
                      n529 = for {
                        N: 12 -> [_]
                        tunnel: w1054 -> [w1062] mode=indexing
                        tunnel: w1053 -> [w1063]
                        i -> [w1060]
                        n530 = Index Array(array=w1063, index=w1060) -> (element=w1061:bool)
                        n531 = Select(t=0, s=w1061, f=2) -> (s? t:f=w1059:i32)
                        n532 = property class="Ctl"(reference=w1062, "DisabledEnum"=w1059) -> ()  [unwired: 1 in, 2 out]
                      }
                    }
                    frame 6 {
                      n533 = control-ref of="1 24"() -> (w1067:refnum<vi>)
                      n534 = property class="Clust (严格)"(reference=w1067) -> ("Controls[]"=w1065:refnum<vi>[])  [unwired: 1 in, 2 out]
                      n535 = for {
                        N: 12 -> [_]
                        tunnel: w1065 -> [w1073] mode=indexing
                        tunnel: w1064 -> [w1074]
                        i -> [w1071]
                        n536 = Index Array(array=w1074, index=w1071) -> (element=w1072:bool)
                        n537 = Select(t=0, s=w1072, f=2) -> (s? t:f=w1070:i32)
                        n538 = property class="Ctl"(reference=w1073, "DisabledEnum"=w1070) -> ()  [unwired: 1 in, 2 out]
                      }
                    }
                    frame 7 {
                      n539 = control-ref of="1 25"() -> (w1078:refnum<vi>)
                      n540 = property class="Clust (严格)"(reference=w1078) -> ("Controls[]"=w1076:refnum<vi>[])  [unwired: 1 in, 2 out]
                      n541 = for {
                        N: 12 -> [_]
                        tunnel: w1076 -> [w1084] mode=indexing
                        tunnel: w1075 -> [w1085]
                        i -> [w1082]
                        n542 = Index Array(array=w1085, index=w1082) -> (element=w1083:bool)
                        n543 = Select(t=0, s=w1083, f=2) -> (s? t:f=w1081:i32)
                        n544 = property class="Ctl"(reference=w1084, "DisabledEnum"=w1081) -> ()  [unwired: 1 in, 2 out]
                      }
                    }
                    frame 8 {
                      n545 = control-ref of="1 5"() -> (w1089:refnum<vi>)
                      n546 = property class="Clust (严格)"(reference=w1089) -> ("Controls[]"=w1087:refnum<vi>[])  [unwired: 1 in, 2 out]
                      n547 = for {
                        N: 12 -> [_]
                        tunnel: w1087 -> [w1095] mode=indexing
                        tunnel: w1086 -> [w1096]
                        i -> [w1093]
                        n548 = Index Array(array=w1096, index=w1093) -> (element=w1094:bool)
                        n549 = Select(t=0, s=w1094, f=2) -> (s? t:f=w1092:i32)
                        n550 = property class="Ctl"(reference=w1095, "DisabledEnum"=w1092) -> ()  [unwired: 1 in, 2 out]
                      }
                    }
                    frame 99, Default {
                    }
                  }
                }
              }
              frame "单体温度" {
                n551 = for {
                  N: 300 -> [_]
                  tunnel: [TRUE] -> w1098 mode=indexing
                }
                n552 = for {
                  N: 9 -> [_]
                  tunnel: w1098 -> [w1288]
                  i -> [w1289]
                  w1286 = 12 ("y")
                  n553 = Add(x=16, y=w1289) -> (x+y=w1284:i32)
                  n554 = Multiply(x=w1284, y=w1286) -> (x*y=w1287:i32)
                  n555 = Array Subset(array=w1288, index=w1287, length=w1286) -> (w1285:bool[])
                  n556 = case shown="0" w1289 {
                    tunnel: w1285 -> [w1290 w1301 w1312 w1323 w1334 w1345 w1356 w1367 w1378 _]
                    frame 0 {
                      n557 = control-ref of="1 18"() -> (w1293:refnum<vi>)
                      n558 = property class="Clust (严格)"(reference=w1293) -> ("Controls[]"=w1291:refnum<vi>[])  [unwired: 1 in, 2 out]
                      n559 = for {
                        N: 12 -> [_]
                        tunnel: w1291 -> [w1299] mode=indexing
                        tunnel: w1290 -> [w1300]
                        i -> [w1297]
                        n560 = Index Array(array=w1300, index=w1297) -> (element=w1298:bool)
                        n561 = Select(t=0, s=w1298, f=2) -> (s? t:f=w1296:i32)
                        n562 = property class="Ctl"(reference=w1299, "DisabledEnum"=w1296) -> ()  [unwired: 1 in, 2 out]
                      }
                    }
                    frame 1 {
                      n563 = control-ref of="1 19"() -> (w1304:refnum<vi>)
                      n564 = property class="Clust (严格)"(reference=w1304) -> ("Controls[]"=w1302:refnum<vi>[])  [unwired: 1 in, 2 out]
                      n565 = for {
                        N: 12 -> [_]
                        tunnel: w1302 -> [w1310] mode=indexing
                        tunnel: w1301 -> [w1311]
                        i -> [w1308]
                        n566 = Index Array(array=w1311, index=w1308) -> (element=w1309:bool)
                        n567 = Select(t=0, s=w1309, f=2) -> (s? t:f=w1307:i32)
                        n568 = property class="Ctl"(reference=w1310, "DisabledEnum"=w1307) -> ()  [unwired: 1 in, 2 out]
                      }
                    }
                    frame 2 {
                      n569 = control-ref of="1 20"() -> (w1315:refnum<vi>)
                      n570 = property class="Clust (严格)"(reference=w1315) -> ("Controls[]"=w1313:refnum<vi>[])  [unwired: 1 in, 2 out]
                      n571 = for {
                        N: 12 -> [_]
                        tunnel: w1313 -> [w1321] mode=indexing
                        tunnel: w1312 -> [w1322]
                        i -> [w1319]
                        n572 = Index Array(array=w1322, index=w1319) -> (element=w1320:bool)
                        n573 = Select(t=0, s=w1320, f=2) -> (s? t:f=w1318:i32)
                        n574 = property class="Ctl"(reference=w1321, "DisabledEnum"=w1318) -> ()  [unwired: 1 in, 2 out]
                      }
                    }
                    frame 3 {
                      n575 = control-ref of="1 21"() -> (w1326:refnum<vi>)
                      n576 = property class="Clust (严格)"(reference=w1326) -> ("Controls[]"=w1324:refnum<vi>[])  [unwired: 1 in, 2 out]
                      n577 = for {
                        N: 12 -> [_]
                        tunnel: w1324 -> [w1332] mode=indexing
                        tunnel: w1323 -> [w1333]
                        i -> [w1330]
                        n578 = Index Array(array=w1333, index=w1330) -> (element=w1331:bool)
                        n579 = Select(t=0, s=w1331, f=2) -> (s? t:f=w1329:i32)
                        n580 = property class="Ctl"(reference=w1332, "DisabledEnum"=w1329) -> ()  [unwired: 1 in, 2 out]
                      }
                    }
                    frame 4 {
                      n581 = control-ref of="1 22"() -> (w1337:refnum<vi>)
                      n582 = property class="Clust (严格)"(reference=w1337) -> ("Controls[]"=w1335:refnum<vi>[])  [unwired: 1 in, 2 out]
                      n583 = for {
                        N: 12 -> [_]
                        tunnel: w1335 -> [w1343] mode=indexing
                        tunnel: w1334 -> [w1344]
                        i -> [w1341]
                        n584 = Index Array(array=w1344, index=w1341) -> (element=w1342:bool)
                        n585 = Select(t=0, s=w1342, f=2) -> (s? t:f=w1340:i32)
                        n586 = property class="Ctl"(reference=w1343, "DisabledEnum"=w1340) -> ()  [unwired: 1 in, 2 out]
                      }
                    }
                    frame 5 {
                      n587 = control-ref of="1 23"() -> (w1348:refnum<vi>)
                      n588 = property class="Clust (严格)"(reference=w1348) -> ("Controls[]"=w1346:refnum<vi>[])  [unwired: 1 in, 2 out]
                      n589 = for {
                        N: 12 -> [_]
                        tunnel: w1346 -> [w1354] mode=indexing
                        tunnel: w1345 -> [w1355]
                        i -> [w1352]
                        n590 = Index Array(array=w1355, index=w1352) -> (element=w1353:bool)
                        n591 = Select(t=0, s=w1353, f=2) -> (s? t:f=w1351:i32)
                        n592 = property class="Ctl"(reference=w1354, "DisabledEnum"=w1351) -> ()  [unwired: 1 in, 2 out]
                      }
                    }
                    frame 6 {
                      n593 = control-ref of="1 24"() -> (w1359:refnum<vi>)
                      n594 = property class="Clust (严格)"(reference=w1359) -> ("Controls[]"=w1357:refnum<vi>[])  [unwired: 1 in, 2 out]
                      n595 = for {
                        N: 12 -> [_]
                        tunnel: w1357 -> [w1365] mode=indexing
                        tunnel: w1356 -> [w1366]
                        i -> [w1363]
                        n596 = Index Array(array=w1366, index=w1363) -> (element=w1364:bool)
                        n597 = Select(t=0, s=w1364, f=2) -> (s? t:f=w1362:i32)
                        n598 = property class="Ctl"(reference=w1365, "DisabledEnum"=w1362) -> ()  [unwired: 1 in, 2 out]
                      }
                    }
                    frame 7 {
                      n599 = control-ref of="1 25"() -> (w1370:refnum<vi>)
                      n600 = property class="Clust (严格)"(reference=w1370) -> ("Controls[]"=w1368:refnum<vi>[])  [unwired: 1 in, 2 out]
                      n601 = for {
                        N: 12 -> [_]
                        tunnel: w1368 -> [w1376] mode=indexing
                        tunnel: w1367 -> [w1377]
                        i -> [w1374]
                        n602 = Index Array(array=w1377, index=w1374) -> (element=w1375:bool)
                        n603 = Select(t=0, s=w1375, f=2) -> (s? t:f=w1373:i32)
                        n604 = property class="Ctl"(reference=w1376, "DisabledEnum"=w1373) -> ()  [unwired: 1 in, 2 out]
                      }
                    }
                    frame 8 {
                      n605 = control-ref of="1 6"() -> (w1381:refnum<vi>)
                      n606 = property class="Clust (严格)"(reference=w1381) -> ("Controls[]"=w1379:refnum<vi>[])  [unwired: 1 in, 2 out]
                      n607 = for {
                        N: 12 -> [_]
                        tunnel: w1379 -> [w1387] mode=indexing
                        tunnel: w1378 -> [w1388]
                        i -> [w1385]
                        n608 = Index Array(array=w1388, index=w1385) -> (element=w1386:bool)
                        n609 = Select(t=0, s=w1386, f=2) -> (s? t:f=w1384:i32)
                        n610 = property class="Ctl"(reference=w1387, "DisabledEnum"=w1384) -> ()  [unwired: 1 in, 2 out]
                      }
                    }
                    frame 99, Default {
                    }
                  }
                }
                n611 = for {
                  N: 16 -> [_]
                  tunnel: w1098 -> [w1105]
                  i -> [w1106]
                  w1103 = 12 ("y")
                  n612 = Multiply(x=w1106, y=w1103) -> (x*y=w1104:i32)
                  n613 = Array Subset(array=w1105, index=w1104, length=w1103) -> (w1102:bool[])
                  n614 = case shown="15" w1106 {
                    tunnel: w1102 -> [w1107 w1118 w1129 w1140 w1151 w1162 w1173 w1184 w1195 w1206 w1217 w1228 w1239 w1250 w1261 w1272 _]
                    frame 0 {
                      n615 = control-ref of="1 102"() -> (w1110:refnum<vi>)
                      n616 = property class="Clust (严格)"(reference=w1110) -> ("Controls[]"=w1108:refnum<vi>[])  [unwired: 1 in, 2 out]
                      n617 = for {
                        N: 12 -> [_]
                        tunnel: w1108 -> [w1116] mode=indexing
                        tunnel: w1107 -> [w1117]
                        i -> [w1114]
                        n618 = Index Array(array=w1117, index=w1114) -> (element=w1115:bool)
                        n619 = Select(t=0, s=w1115, f=2) -> (s? t:f=w1113:i32)
                        n620 = property class="Ctl"(reference=w1116, "DisabledEnum"=w1113) -> ()  [unwired: 1 in, 2 out]
                      }
                    }
                    frame 1 {
                      n621 = control-ref of="1 3"() -> (w1121:refnum<vi>)
                      n622 = property class="Clust (严格)"(reference=w1121) -> ("Controls[]"=w1119:refnum<vi>[])  [unwired: 1 in, 2 out]
                      n623 = for {
                        N: 12 -> [_]
                        tunnel: w1119 -> [w1127] mode=indexing
                        tunnel: w1118 -> [w1128]
                        i -> [w1125]
                        n624 = Index Array(array=w1128, index=w1125) -> (element=w1126:bool)
                        n625 = Select(t=0, s=w1126, f=2) -> (s? t:f=w1124:i32)
                        n626 = property class="Ctl"(reference=w1127, "DisabledEnum"=w1124) -> ()  [unwired: 1 in, 2 out]
                      }
                    }
                    frame 2 {
                      n627 = control-ref of="1 4"() -> (w1132:refnum<vi>)
                      n628 = property class="Clust (严格)"(reference=w1132) -> ("Controls[]"=w1130:refnum<vi>[])  [unwired: 1 in, 2 out]
                      n629 = for {
                        N: 12 -> [_]
                        tunnel: w1130 -> [w1138] mode=indexing
                        tunnel: w1129 -> [w1139]
                        i -> [w1136]
                        n630 = Index Array(array=w1139, index=w1136) -> (element=w1137:bool)
                        n631 = Select(t=0, s=w1137, f=2) -> (s? t:f=w1135:i32)
                        n632 = property class="Ctl"(reference=w1138, "DisabledEnum"=w1135) -> ()  [unwired: 1 in, 2 out]
                      }
                    }
                    frame 3 {
                      n633 = control-ref of="1 6"() -> (w1143:refnum<vi>)
                      n634 = property class="Clust (严格)"(reference=w1143) -> ("Controls[]"=w1141:refnum<vi>[])  [unwired: 1 in, 2 out]
                      n635 = for {
                        N: 12 -> [_]
                        tunnel: w1141 -> [w1149] mode=indexing
                        tunnel: w1140 -> [w1150]
                        i -> [w1147]
                        n636 = Index Array(array=w1150, index=w1147) -> (element=w1148:bool)
                        n637 = Select(t=0, s=w1148, f=2) -> (s? t:f=w1146:i32)
                        n638 = property class="Ctl"(reference=w1149, "DisabledEnum"=w1146) -> ()  [unwired: 1 in, 2 out]
                      }
                    }
                    frame 4 {
                      n639 = control-ref of="1 7"() -> (w1154:refnum<vi>)
                      n640 = property class="Clust (严格)"(reference=w1154) -> ("Controls[]"=w1152:refnum<vi>[])  [unwired: 1 in, 2 out]
                      n641 = for {
                        N: 12 -> [_]
                        tunnel: w1152 -> [w1160] mode=indexing
                        tunnel: w1151 -> [w1161]
                        i -> [w1158]
                        n642 = Index Array(array=w1161, index=w1158) -> (element=w1159:bool)
                        n643 = Select(t=0, s=w1159, f=2) -> (s? t:f=w1157:i32)
                        n644 = property class="Ctl"(reference=w1160, "DisabledEnum"=w1157) -> ()  [unwired: 1 in, 2 out]
                      }
                    }
                    frame 5 {
                      n645 = control-ref of="1 8"() -> (w1165:refnum<vi>)
                      n646 = property class="Clust (严格)"(reference=w1165) -> ("Controls[]"=w1163:refnum<vi>[])  [unwired: 1 in, 2 out]
                      n647 = for {
                        N: 12 -> [_]
                        tunnel: w1163 -> [w1171] mode=indexing
                        tunnel: w1162 -> [w1172]
                        i -> [w1169]
                        n648 = Index Array(array=w1172, index=w1169) -> (element=w1170:bool)
                        n649 = Select(t=0, s=w1170, f=2) -> (s? t:f=w1168:i32)
                        n650 = property class="Ctl"(reference=w1171, "DisabledEnum"=w1168) -> ()  [unwired: 1 in, 2 out]
                      }
                    }
                    frame 6 {
                      n651 = control-ref of="1 9"() -> (w1176:refnum<vi>)
                      n652 = property class="Clust (严格)"(reference=w1176) -> ("Controls[]"=w1174:refnum<vi>[])  [unwired: 1 in, 2 out]
                      n653 = for {
                        N: 12 -> [_]
                        tunnel: w1174 -> [w1182] mode=indexing
                        tunnel: w1173 -> [w1183]
                        i -> [w1180]
                        n654 = Index Array(array=w1183, index=w1180) -> (element=w1181:bool)
                        n655 = Select(t=0, s=w1181, f=2) -> (s? t:f=w1179:i32)
                        n656 = property class="Ctl"(reference=w1182, "DisabledEnum"=w1179) -> ()  [unwired: 1 in, 2 out]
                      }
                    }
                    frame 7 {
                      n657 = control-ref of="1 10"() -> (w1187:refnum<vi>)
                      n658 = property class="Clust (严格)"(reference=w1187) -> ("Controls[]"=w1185:refnum<vi>[])  [unwired: 1 in, 2 out]
                      n659 = for {
                        N: 12 -> [_]
                        tunnel: w1185 -> [w1193] mode=indexing
                        tunnel: w1184 -> [w1194]
                        i -> [w1191]
                        n660 = Index Array(array=w1194, index=w1191) -> (element=w1192:bool)
                        n661 = Select(t=0, s=w1192, f=2) -> (s? t:f=w1190:i32)
                        n662 = property class="Ctl"(reference=w1193, "DisabledEnum"=w1190) -> ()  [unwired: 1 in, 2 out]
                      }
                    }
                    frame 8 {
                      n663 = control-ref of="1 26"() -> (w1198:refnum<vi>)
                      n664 = property class="Clust (严格)"(reference=w1198) -> ("Controls[]"=w1196:refnum<vi>[])  [unwired: 1 in, 2 out]
                      n665 = for {
                        N: 12 -> [_]
                        tunnel: w1196 -> [w1204] mode=indexing
                        tunnel: w1195 -> [w1205]
                        i -> [w1202]
                        n666 = Index Array(array=w1205, index=w1202) -> (element=w1203:bool)
                        n667 = Select(t=0, s=w1203, f=2) -> (s? t:f=w1201:i32)
                        n668 = property class="Ctl"(reference=w1204, "DisabledEnum"=w1201) -> ()  [unwired: 1 in, 2 out]
                      }
                    }
                    frame 9 {
                      n669 = control-ref of="1 27"() -> (w1209:refnum<vi>)
                      n670 = property class="Clust (严格)"(reference=w1209) -> ("Controls[]"=w1207:refnum<vi>[])  [unwired: 1 in, 2 out]
                      n671 = for {
                        N: 12 -> [_]
                        tunnel: w1207 -> [w1215] mode=indexing
                        tunnel: w1206 -> [w1216]
                        i -> [w1213]
                        n672 = Index Array(array=w1216, index=w1213) -> (element=w1214:bool)
                        n673 = Select(t=0, s=w1214, f=2) -> (s? t:f=w1212:i32)
                        n674 = property class="Ctl"(reference=w1215, "DisabledEnum"=w1212) -> ()  [unwired: 1 in, 2 out]
                      }
                    }
                    frame 10 {
                      n675 = control-ref of="1 28"() -> (w1220:refnum<vi>)
                      n676 = property class="Clust (严格)"(reference=w1220) -> ("Controls[]"=w1218:refnum<vi>[])  [unwired: 1 in, 2 out]
                      n677 = for {
                        N: 12 -> [_]
                        tunnel: w1218 -> [w1226] mode=indexing
                        tunnel: w1217 -> [w1227]
                        i -> [w1224]
                        n678 = Index Array(array=w1227, index=w1224) -> (element=w1225:bool)
                        n679 = Select(t=0, s=w1225, f=2) -> (s? t:f=w1223:i32)
                        n680 = property class="Ctl"(reference=w1226, "DisabledEnum"=w1223) -> ()  [unwired: 1 in, 2 out]
                      }
                    }
                    frame 11 {
                      n681 = control-ref of="1 29"() -> (w1231:refnum<vi>)
                      n682 = property class="Clust (严格)"(reference=w1231) -> ("Controls[]"=w1229:refnum<vi>[])  [unwired: 1 in, 2 out]
                      n683 = for {
                        N: 12 -> [_]
                        tunnel: w1229 -> [w1237] mode=indexing
                        tunnel: w1228 -> [w1238]
                        i -> [w1235]
                        n684 = Index Array(array=w1238, index=w1235) -> (element=w1236:bool)
                        n685 = Select(t=0, s=w1236, f=2) -> (s? t:f=w1234:i32)
                        n686 = property class="Ctl"(reference=w1237, "DisabledEnum"=w1234) -> ()  [unwired: 1 in, 2 out]
                      }
                    }
                    frame 12 {
                      n687 = control-ref of="1 30"() -> (w1242:refnum<vi>)
                      n688 = property class="Clust (严格)"(reference=w1242) -> ("Controls[]"=w1240:refnum<vi>[])  [unwired: 1 in, 2 out]
                      n689 = for {
                        N: 12 -> [_]
                        tunnel: w1240 -> [w1248] mode=indexing
                        tunnel: w1239 -> [w1249]
                        i -> [w1246]
                        n690 = Index Array(array=w1249, index=w1246) -> (element=w1247:bool)
                        n691 = Select(t=0, s=w1247, f=2) -> (s? t:f=w1245:i32)
                        n692 = property class="Ctl"(reference=w1248, "DisabledEnum"=w1245) -> ()  [unwired: 1 in, 2 out]
                      }
                    }
                    frame 13 {
                      n693 = control-ref of="1 31"() -> (w1253:refnum<vi>)
                      n694 = property class="Clust (严格)"(reference=w1253) -> ("Controls[]"=w1251:refnum<vi>[])  [unwired: 1 in, 2 out]
                      n695 = for {
                        N: 12 -> [_]
                        tunnel: w1251 -> [w1259] mode=indexing
                        tunnel: w1250 -> [w1260]
                        i -> [w1257]
                        n696 = Index Array(array=w1260, index=w1257) -> (element=w1258:bool)
                        n697 = Select(t=0, s=w1258, f=2) -> (s? t:f=w1256:i32)
                        n698 = property class="Ctl"(reference=w1259, "DisabledEnum"=w1256) -> ()  [unwired: 1 in, 2 out]
                      }
                    }
                    frame 14 {
                      n699 = control-ref of="1 32"() -> (w1264:refnum<vi>)
                      n700 = property class="Clust (严格)"(reference=w1264) -> ("Controls[]"=w1262:refnum<vi>[])  [unwired: 1 in, 2 out]
                      n701 = for {
                        N: 12 -> [_]
                        tunnel: w1262 -> [w1270] mode=indexing
                        tunnel: w1261 -> [w1271]
                        i -> [w1268]
                        n702 = Index Array(array=w1271, index=w1268) -> (element=w1269:bool)
                        n703 = Select(t=0, s=w1269, f=2) -> (s? t:f=w1267:i32)
                        n704 = property class="Ctl"(reference=w1270, "DisabledEnum"=w1267) -> ()  [unwired: 1 in, 2 out]
                      }
                    }
                    frame 15 {
                      n705 = control-ref of="1 33"() -> (w1275:refnum<vi>)
                      n706 = property class="Clust (严格)"(reference=w1275) -> ("Controls[]"=w1273:refnum<vi>[])  [unwired: 1 in, 2 out]
                      n707 = for {
                        N: 12 -> [_]
                        tunnel: w1273 -> [w1281] mode=indexing
                        tunnel: w1272 -> [w1282]
                        i -> [w1279]
                        n708 = Index Array(array=w1282, index=w1279) -> (element=w1280:bool)
                        n709 = Select(t=0, s=w1280, f=2) -> (s? t:f=w1278:i32)
                        n710 = property class="Ctl"(reference=w1281, "DisabledEnum"=w1278) -> ()  [unwired: 1 in, 2 out]
                      }
                    }
                    frame 99, Default {
                    }
                  }
                }
              }
            }
          }
        }
      }
    }
    frame Enabled {
    }
  }
  n711 = disable-structure shown="启用" {
    frame Enabled {
      n712 = while {
        stop <- w1393 stop-if-true
        n713 = local read "选项卡控件"() -> (w1392:enum32{"单体电压", "单体温度", "单体内阻", "单体SOC"})
        n714 = local read "停止"() -> (w1393:bool)
        n715 = Wait Until Next ms Multiple(millisecond multiple=u32 500 ("毫秒倍数")) -> ()  [unwired: 1 out]
        n716 = Or(x="布尔", y="布尔 2") -> (x .or. y?=w1391:bool)
        n717 = case shown="真" w1391 {
          tunnel: w1392 -> [w1395 w1662]
          frame False {
            n718 = case shown="真" "一次置位" {
              tunnel: w1395 -> [_ w1397]
              frame False {
              }
              frame True {
                n719 = case shown="\"单体温度\"" w1397 {
                  frame "单体电压", Default {
                    n720 = for {
                      N: 9 -> [_]
                      i -> [w1483]
                      n721 = case shown="0" w1483 {
                        tunnel: bool[] [FALSE, FALSE, FALSE, FALSE, FALSE, FALSE, FALSE, FALSE, FALSE, FALSE, FALSE, FALSE, FALSE] -> [w1486 w1491 w1496 w1501 w1506 w1511 w1516 w1521 w1526 _]
                        frame 0 {
                          n722 = control-ref of="1 18"() -> (w1485:refnum<vi>)
                          n723 = property class="Clust (严格)"(reference=w1485) -> ("Controls[]"=w1487:refnum<vi>[])  [unwired: 1 in, 2 out]
                          n724 = for {
                            tunnel: w1487 -> [w1488] mode=indexing
                            tunnel: w1486 -> [w1489] mode=indexing
                            n725 = property class="Ctl"(reference=w1488, "Blinking"=w1489) -> ()  [unwired: 1 in, 2 out]
                          }
                        }
                        frame 1 {
                          n726 = control-ref of="1 19"() -> (w1490:refnum<vi>)
                          n727 = property class="Clust (严格)"(reference=w1490) -> ("Controls[]"=w1492:refnum<vi>[])  [unwired: 1 in, 2 out]
                          n728 = for {
                            tunnel: w1492 -> [w1493] mode=indexing
                            tunnel: w1491 -> [w1494] mode=indexing
                            n729 = property class="Ctl"(reference=w1493, "Blinking"=w1494) -> ()  [unwired: 1 in, 2 out]
                          }
                        }
                        frame 2 {
                          n730 = control-ref of="1 20"() -> (w1495:refnum<vi>)
                          n731 = property class="Clust (严格)"(reference=w1495) -> ("Controls[]"=w1497:refnum<vi>[])  [unwired: 1 in, 2 out]
                          n732 = for {
                            tunnel: w1497 -> [w1498] mode=indexing
                            tunnel: w1496 -> [w1499] mode=indexing
                            n733 = property class="Ctl"(reference=w1498, "Blinking"=w1499) -> ()  [unwired: 1 in, 2 out]
                          }
                        }
                        frame 3 {
                          n734 = control-ref of="1 21"() -> (w1500:refnum<vi>)
                          n735 = property class="Clust (严格)"(reference=w1500) -> ("Controls[]"=w1502:refnum<vi>[])  [unwired: 1 in, 2 out]
                          n736 = for {
                            tunnel: w1502 -> [w1503] mode=indexing
                            tunnel: w1501 -> [w1504] mode=indexing
                            n737 = property class="Ctl"(reference=w1503, "Blinking"=w1504) -> ()  [unwired: 1 in, 2 out]
                          }
                        }
                        frame 4 {
                          n738 = control-ref of="1 22"() -> (w1505:refnum<vi>)
                          n739 = property class="Clust (严格)"(reference=w1505) -> ("Controls[]"=w1507:refnum<vi>[])  [unwired: 1 in, 2 out]
                          n740 = for {
                            tunnel: w1507 -> [w1508] mode=indexing
                            tunnel: w1506 -> [w1509] mode=indexing
                            n741 = property class="Ctl"(reference=w1508, "Blinking"=w1509) -> ()  [unwired: 1 in, 2 out]
                          }
                        }
                        frame 5 {
                          n742 = control-ref of="1 23"() -> (w1510:refnum<vi>)
                          n743 = property class="Clust (严格)"(reference=w1510) -> ("Controls[]"=w1512:refnum<vi>[])  [unwired: 1 in, 2 out]
                          n744 = for {
                            tunnel: w1512 -> [w1513] mode=indexing
                            tunnel: w1511 -> [w1514] mode=indexing
                            n745 = property class="Ctl"(reference=w1513, "Blinking"=w1514) -> ()  [unwired: 1 in, 2 out]
                          }
                        }
                        frame 6 {
                          n746 = control-ref of="1 24"() -> (w1515:refnum<vi>)
                          n747 = property class="Clust (严格)"(reference=w1515) -> ("Controls[]"=w1517:refnum<vi>[])  [unwired: 1 in, 2 out]
                          n748 = for {
                            tunnel: w1517 -> [w1518] mode=indexing
                            tunnel: w1516 -> [w1519] mode=indexing
                            n749 = property class="Ctl"(reference=w1518, "Blinking"=w1519) -> ()  [unwired: 1 in, 2 out]
                          }
                        }
                        frame 7 {
                          n750 = control-ref of="1 25"() -> (w1520:refnum<vi>)
                          n751 = property class="Clust (严格)"(reference=w1520) -> ("Controls[]"=w1522:refnum<vi>[])  [unwired: 1 in, 2 out]
                          n752 = for {
                            tunnel: w1522 -> [w1523] mode=indexing
                            tunnel: w1521 -> [w1524] mode=indexing
                            n753 = property class="Ctl"(reference=w1523, "Blinking"=w1524) -> ()  [unwired: 1 in, 2 out]
                          }
                        }
                        frame 8 {
                          n754 = control-ref of="1 5"() -> (w1525:refnum<vi>)
                          n755 = property class="Clust (严格)"(reference=w1525) -> ("Controls[]"=w1527:refnum<vi>[])  [unwired: 1 in, 2 out]
                          n756 = for {
                            tunnel: w1527 -> [w1528] mode=indexing
                            tunnel: w1526 -> [w1529] mode=indexing
                            n757 = property class="Ctl"(reference=w1528, "Blinking"=w1529) -> ()  [unwired: 1 in, 2 out]
                          }
                        }
                        frame 99, Default {
                        }
                      }
                    }
                    n758 = for {
                      N: 16 -> [_]
                      i -> [w1402]
                      n759 = case shown="6" w1402 {
                        tunnel: bool[] [FALSE, FALSE, FALSE, FALSE, FALSE, FALSE, FALSE, FALSE, FALSE, FALSE, FALSE, FALSE, FALSE] -> [w1403 w1409 w1414 w1419 w1424 w1429 w1434 w1439 w1444 w1449 w1454 w1459 w1464 w1469 w1474 w1479 _]
                        frame 0 {
                          n760 = control-ref of="1 102"() -> (w1405:refnum<vi>)
                          n761 = property class="Clust (严格)"(reference=w1405) -> ("Controls[]"=w1404:refnum<vi>[])  [unwired: 1 in, 2 out]
                          n762 = for {
                            tunnel: w1404 -> [w1406] mode=indexing
                            tunnel: w1403 -> [w1407] mode=indexing
                            n763 = property class="Ctl"(reference=w1406, "Blinking"=w1407) -> ()  [unwired: 1 in, 2 out]
                          }
                        }
                        frame 1 {
                          n764 = control-ref of="1 3"() -> (w1408:refnum<vi>)
                          n765 = property class="Clust (严格)"(reference=w1408) -> ("Controls[]"=w1410:refnum<vi>[])  [unwired: 1 in, 2 out]
                          n766 = for {
                            tunnel: w1410 -> [w1411] mode=indexing
                            tunnel: w1409 -> [w1412] mode=indexing
                            n767 = property class="Ctl"(reference=w1411, "Blinking"=w1412) -> ()  [unwired: 1 in, 2 out]
                          }
                        }
                        frame 2 {
                          n768 = control-ref of="1 4"() -> (w1413:refnum<vi>)
                          n769 = property class="Clust (严格)"(reference=w1413) -> ("Controls[]"=w1415:refnum<vi>[])  [unwired: 1 in, 2 out]
                          n770 = for {
                            tunnel: w1415 -> [w1416] mode=indexing
                            tunnel: w1414 -> [w1417] mode=indexing
                            n771 = property class="Ctl"(reference=w1416, "Blinking"=w1417) -> ()  [unwired: 1 in, 2 out]
                          }
                        }
                        frame 3 {
                          n772 = control-ref of="1 6"() -> (w1418:refnum<vi>)
                          n773 = property class="Clust (严格)"(reference=w1418) -> ("Controls[]"=w1420:refnum<vi>[])  [unwired: 1 in, 2 out]
                          n774 = for {
                            tunnel: w1420 -> [w1421] mode=indexing
                            tunnel: w1419 -> [w1422] mode=indexing
                            n775 = property class="Ctl"(reference=w1421, "Blinking"=w1422) -> ()  [unwired: 1 in, 2 out]
                          }
                        }
                        frame 4 {
                          n776 = control-ref of="1 7"() -> (w1423:refnum<vi>)
                          n777 = property class="Clust (严格)"(reference=w1423) -> ("Controls[]"=w1425:refnum<vi>[])  [unwired: 1 in, 2 out]
                          n778 = for {
                            tunnel: w1425 -> [w1426] mode=indexing
                            tunnel: w1424 -> [w1427] mode=indexing
                            n779 = property class="Ctl"(reference=w1426, "Blinking"=w1427) -> ()  [unwired: 1 in, 2 out]
                          }
                        }
                        frame 5 {
                          n780 = control-ref of="1 8"() -> (w1428:refnum<vi>)
                          n781 = property class="Clust (严格)"(reference=w1428) -> ("Controls[]"=w1430:refnum<vi>[])  [unwired: 1 in, 2 out]
                          n782 = for {
                            tunnel: w1430 -> [w1431] mode=indexing
                            tunnel: w1429 -> [w1432] mode=indexing
                            n783 = property class="Ctl"(reference=w1431, "Blinking"=w1432) -> ()  [unwired: 1 in, 2 out]
                          }
                        }
                        frame 6 {
                          n784 = control-ref of="1 9"() -> (w1433:refnum<vi>)
                          n785 = property class="Clust (严格)"(reference=w1433) -> ("Controls[]"=w1435:refnum<vi>[])  [unwired: 1 in, 2 out]
                          n786 = for {
                            tunnel: w1435 -> [w1436] mode=indexing
                            tunnel: w1434 -> [w1437] mode=indexing
                            n787 = property class="Ctl"(reference=w1436, "Blinking"=w1437) -> ()  [unwired: 1 in, 2 out]
                          }
                        }
                        frame 7 {
                          n788 = control-ref of="1 10"() -> (w1438:refnum<vi>)
                          n789 = property class="Clust (严格)"(reference=w1438) -> ("Controls[]"=w1440:refnum<vi>[])  [unwired: 1 in, 2 out]
                          n790 = for {
                            tunnel: w1440 -> [w1441] mode=indexing
                            tunnel: w1439 -> [w1442] mode=indexing
                            n791 = property class="Ctl"(reference=w1441, "Blinking"=w1442) -> ()  [unwired: 1 in, 2 out]
                          }
                        }
                        frame 8 {
                          n792 = control-ref of="1 26"() -> (w1443:refnum<vi>)
                          n793 = property class="Clust (严格)"(reference=w1443) -> ("Controls[]"=w1445:refnum<vi>[])  [unwired: 1 in, 2 out]
                          n794 = for {
                            tunnel: w1445 -> [w1446] mode=indexing
                            tunnel: w1444 -> [w1447] mode=indexing
                            n795 = property class="Ctl"(reference=w1446, "Blinking"=w1447) -> ()  [unwired: 1 in, 2 out]
                          }
                        }
                        frame 9 {
                          n796 = control-ref of="1 27"() -> (w1448:refnum<vi>)
                          n797 = property class="Clust (严格)"(reference=w1448) -> ("Controls[]"=w1450:refnum<vi>[])  [unwired: 1 in, 2 out]
                          n798 = for {
                            tunnel: w1450 -> [w1451] mode=indexing
                            tunnel: w1449 -> [w1452] mode=indexing
                            n799 = property class="Ctl"(reference=w1451, "Blinking"=w1452) -> ()  [unwired: 1 in, 2 out]
                          }
                        }
                        frame 10 {
                          n800 = control-ref of="1 28"() -> (w1453:refnum<vi>)
                          n801 = property class="Clust (严格)"(reference=w1453) -> ("Controls[]"=w1455:refnum<vi>[])  [unwired: 1 in, 2 out]
                          n802 = for {
                            tunnel: w1455 -> [w1456] mode=indexing
                            tunnel: w1454 -> [w1457] mode=indexing
                            n803 = property class="Ctl"(reference=w1456, "Blinking"=w1457) -> ()  [unwired: 1 in, 2 out]
                          }
                        }
                        frame 11 {
                          n804 = control-ref of="1 29"() -> (w1458:refnum<vi>)
                          n805 = property class="Clust (严格)"(reference=w1458) -> ("Controls[]"=w1460:refnum<vi>[])  [unwired: 1 in, 2 out]
                          n806 = for {
                            tunnel: w1460 -> [w1461] mode=indexing
                            tunnel: w1459 -> [w1462] mode=indexing
                            n807 = property class="Ctl"(reference=w1461, "Blinking"=w1462) -> ()  [unwired: 1 in, 2 out]
                          }
                        }
                        frame 12 {
                          n808 = control-ref of="1 30"() -> (w1463:refnum<vi>)
                          n809 = property class="Clust (严格)"(reference=w1463) -> ("Controls[]"=w1465:refnum<vi>[])  [unwired: 1 in, 2 out]
                          n810 = for {
                            tunnel: w1465 -> [w1466] mode=indexing
                            tunnel: w1464 -> [w1467] mode=indexing
                            n811 = property class="Ctl"(reference=w1466, "Blinking"=w1467) -> ()  [unwired: 1 in, 2 out]
                          }
                        }
                        frame 13 {
                          n812 = control-ref of="1 31"() -> (w1468:refnum<vi>)
                          n813 = property class="Clust (严格)"(reference=w1468) -> ("Controls[]"=w1470:refnum<vi>[])  [unwired: 1 in, 2 out]
                          n814 = for {
                            tunnel: w1470 -> [w1471] mode=indexing
                            tunnel: w1469 -> [w1472] mode=indexing
                            n815 = property class="Ctl"(reference=w1471, "Blinking"=w1472) -> ()  [unwired: 1 in, 2 out]
                          }
                        }
                        frame 14 {
                          n816 = control-ref of="1 32"() -> (w1473:refnum<vi>)
                          n817 = property class="Clust (严格)"(reference=w1473) -> ("Controls[]"=w1475:refnum<vi>[])  [unwired: 1 in, 2 out]
                          n818 = for {
                            tunnel: w1475 -> [w1476] mode=indexing
                            tunnel: w1474 -> [w1477] mode=indexing
                            n819 = property class="Ctl"(reference=w1476, "Blinking"=w1477) -> ()  [unwired: 1 in, 2 out]
                          }
                        }
                        frame 15 {
                          n820 = control-ref of="1 33"() -> (w1478:refnum<vi>)
                          n821 = property class="Clust (严格)"(reference=w1478) -> ("Controls[]"=w1480:refnum<vi>[])  [unwired: 1 in, 2 out]
                          n822 = for {
                            tunnel: w1480 -> [w1481] mode=indexing
                            tunnel: w1479 -> [w1482] mode=indexing
                            n823 = property class="Ctl"(reference=w1481, "Blinking"=w1482) -> ()  [unwired: 1 in, 2 out]
                          }
                        }
                        frame 99, Default {
                        }
                      }
                    }
                  }
                  frame "单体温度" {
                    n824 = for {
                      N: 16 -> [_]
                      i -> [w1533]
                      n825 = case shown="4" w1533 {
                        tunnel: bool[] [FALSE, FALSE, FALSE, FALSE, FALSE, FALSE, FALSE, FALSE, FALSE, FALSE, FALSE, FALSE, FALSE] -> [w1535 w1540 w1545 w1550 w1555 w1560 w1565 w1570 w1575 w1580 w1585 w1590 w1595 w1600 w1605 w1610 _]
                        frame 0 {
                          n826 = control-ref of="1 102"() -> (w1534:refnum<vi>)
                          n827 = property class="Clust (严格)"(reference=w1534) -> ("Controls[]"=w1536:refnum<vi>[])  [unwired: 1 in, 2 out]
                          n828 = for {
                            tunnel: w1536 -> [w1537] mode=indexing
                            tunnel: w1535 -> [w1538] mode=indexing
                            n829 = property class="Ctl"(reference=w1537, "Blinking"=w1538) -> ()  [unwired: 1 in, 2 out]
                          }
                        }
                        frame 1 {
                          n830 = control-ref of="1 3"() -> (w1539:refnum<vi>)
                          n831 = property class="Clust (严格)"(reference=w1539) -> ("Controls[]"=w1541:refnum<vi>[])  [unwired: 1 in, 2 out]
                          n832 = for {
                            tunnel: w1541 -> [w1542] mode=indexing
                            tunnel: w1540 -> [w1543] mode=indexing
                            n833 = property class="Ctl"(reference=w1542, "Blinking"=w1543) -> ()  [unwired: 1 in, 2 out]
                          }
                        }
                        frame 2 {
                          n834 = control-ref of="1 4"() -> (w1544:refnum<vi>)
                          n835 = property class="Clust (严格)"(reference=w1544) -> ("Controls[]"=w1546:refnum<vi>[])  [unwired: 1 in, 2 out]
                          n836 = for {
                            tunnel: w1546 -> [w1547] mode=indexing
                            tunnel: w1545 -> [w1548] mode=indexing
                            n837 = property class="Ctl"(reference=w1547, "Blinking"=w1548) -> ()  [unwired: 1 in, 2 out]
                          }
                        }
                        frame 3 {
                          n838 = control-ref of="1 6"() -> (w1549:refnum<vi>)
                          n839 = property class="Clust (严格)"(reference=w1549) -> ("Controls[]"=w1551:refnum<vi>[])  [unwired: 1 in, 2 out]
                          n840 = for {
                            tunnel: w1551 -> [w1552] mode=indexing
                            tunnel: w1550 -> [w1553] mode=indexing
                            n841 = property class="Ctl"(reference=w1552, "Blinking"=w1553) -> ()  [unwired: 1 in, 2 out]
                          }
                        }
                        frame 4 {
                          n842 = control-ref of="1 7"() -> (w1554:refnum<vi>)
                          n843 = property class="Clust (严格)"(reference=w1554) -> ("Controls[]"=w1556:refnum<vi>[])  [unwired: 1 in, 2 out]
                          n844 = for {
                            tunnel: w1556 -> [w1557] mode=indexing
                            tunnel: w1555 -> [w1558] mode=indexing
                            n845 = property class="Ctl"(reference=w1557, "Blinking"=w1558) -> ()  [unwired: 1 in, 2 out]
                          }
                        }
                        frame 5 {
                          n846 = control-ref of="1 8"() -> (w1559:refnum<vi>)
                          n847 = property class="Clust (严格)"(reference=w1559) -> ("Controls[]"=w1561:refnum<vi>[])  [unwired: 1 in, 2 out]
                          n848 = for {
                            tunnel: w1561 -> [w1562] mode=indexing
                            tunnel: w1560 -> [w1563] mode=indexing
                            n849 = property class="Ctl"(reference=w1562, "Blinking"=w1563) -> ()  [unwired: 1 in, 2 out]
                          }
                        }
                        frame 6 {
                          n850 = control-ref of="1 9"() -> (w1564:refnum<vi>)
                          n851 = property class="Clust (严格)"(reference=w1564) -> ("Controls[]"=w1566:refnum<vi>[])  [unwired: 1 in, 2 out]
                          n852 = for {
                            tunnel: w1566 -> [w1567] mode=indexing
                            tunnel: w1565 -> [w1568] mode=indexing
                            n853 = property class="Ctl"(reference=w1567, "Blinking"=w1568) -> ()  [unwired: 1 in, 2 out]
                          }
                        }
                        frame 7 {
                          n854 = control-ref of="1 10"() -> (w1569:refnum<vi>)
                          n855 = property class="Clust (严格)"(reference=w1569) -> ("Controls[]"=w1571:refnum<vi>[])  [unwired: 1 in, 2 out]
                          n856 = for {
                            tunnel: w1571 -> [w1572] mode=indexing
                            tunnel: w1570 -> [w1573] mode=indexing
                            n857 = property class="Ctl"(reference=w1572, "Blinking"=w1573) -> ()  [unwired: 1 in, 2 out]
                          }
                        }
                        frame 8 {
                          n858 = control-ref of="1 26"() -> (w1574:refnum<vi>)
                          n859 = property class="Clust (严格)"(reference=w1574) -> ("Controls[]"=w1576:refnum<vi>[])  [unwired: 1 in, 2 out]
                          n860 = for {
                            tunnel: w1576 -> [w1577] mode=indexing
                            tunnel: w1575 -> [w1578] mode=indexing
                            n861 = property class="Ctl"(reference=w1577, "Blinking"=w1578) -> ()  [unwired: 1 in, 2 out]
                          }
                        }
                        frame 9 {
                          n862 = control-ref of="1 27"() -> (w1579:refnum<vi>)
                          n863 = property class="Clust (严格)"(reference=w1579) -> ("Controls[]"=w1581:refnum<vi>[])  [unwired: 1 in, 2 out]
                          n864 = for {
                            tunnel: w1581 -> [w1582] mode=indexing
                            tunnel: w1580 -> [w1583] mode=indexing
                            n865 = property class="Ctl"(reference=w1582, "Blinking"=w1583) -> ()  [unwired: 1 in, 2 out]
                          }
                        }
                        frame 10 {
                          n866 = control-ref of="1 28"() -> (w1584:refnum<vi>)
                          n867 = property class="Clust (严格)"(reference=w1584) -> ("Controls[]"=w1586:refnum<vi>[])  [unwired: 1 in, 2 out]
                          n868 = for {
                            tunnel: w1586 -> [w1587] mode=indexing
                            tunnel: w1585 -> [w1588] mode=indexing
                            n869 = property class="Ctl"(reference=w1587, "Blinking"=w1588) -> ()  [unwired: 1 in, 2 out]
                          }
                        }
                        frame 11 {
                          n870 = control-ref of="1 29"() -> (w1589:refnum<vi>)
                          n871 = property class="Clust (严格)"(reference=w1589) -> ("Controls[]"=w1591:refnum<vi>[])  [unwired: 1 in, 2 out]
                          n872 = for {
                            tunnel: w1591 -> [w1592] mode=indexing
                            tunnel: w1590 -> [w1593] mode=indexing
                            n873 = property class="Ctl"(reference=w1592, "Blinking"=w1593) -> ()  [unwired: 1 in, 2 out]
                          }
                        }
                        frame 12 {
                          n874 = control-ref of="1 30"() -> (w1594:refnum<vi>)
                          n875 = property class="Clust (严格)"(reference=w1594) -> ("Controls[]"=w1596:refnum<vi>[])  [unwired: 1 in, 2 out]
                          n876 = for {
                            tunnel: w1596 -> [w1597] mode=indexing
                            tunnel: w1595 -> [w1598] mode=indexing
                            n877 = property class="Ctl"(reference=w1597, "Blinking"=w1598) -> ()  [unwired: 1 in, 2 out]
                          }
                        }
                        frame 13 {
                          n878 = control-ref of="1 31"() -> (w1599:refnum<vi>)
                          n879 = property class="Clust (严格)"(reference=w1599) -> ("Controls[]"=w1601:refnum<vi>[])  [unwired: 1 in, 2 out]
                          n880 = for {
                            tunnel: w1601 -> [w1602] mode=indexing
                            tunnel: w1600 -> [w1603] mode=indexing
                            n881 = property class="Ctl"(reference=w1602, "Blinking"=w1603) -> ()  [unwired: 1 in, 2 out]
                          }
                        }
                        frame 14 {
                          n882 = control-ref of="1 32"() -> (w1604:refnum<vi>)
                          n883 = property class="Clust (严格)"(reference=w1604) -> ("Controls[]"=w1606:refnum<vi>[])  [unwired: 1 in, 2 out]
                          n884 = for {
                            tunnel: w1606 -> [w1607] mode=indexing
                            tunnel: w1605 -> [w1608] mode=indexing
                            n885 = property class="Ctl"(reference=w1607, "Blinking"=w1608) -> ()  [unwired: 1 in, 2 out]
                          }
                        }
                        frame 15 {
                          n886 = control-ref of="1 33"() -> (w1609:refnum<vi>)
                          n887 = property class="Clust (严格)"(reference=w1609) -> ("Controls[]"=w1611:refnum<vi>[])  [unwired: 1 in, 2 out]
                          n888 = for {
                            tunnel: w1611 -> [w1612] mode=indexing
                            tunnel: w1610 -> [w1613] mode=indexing
                            n889 = property class="Ctl"(reference=w1612, "Blinking"=w1613) -> ()  [unwired: 1 in, 2 out]
                          }
                        }
                        frame 99, Default {
                        }
                      }
                    }
                    n890 = for {
                      N: 9 -> [_]
                      i -> [w1615]
                      n891 = case shown="8" w1615 {
                        tunnel: bool[] [FALSE, FALSE, FALSE, FALSE, FALSE, FALSE, FALSE, FALSE, FALSE, FALSE, FALSE, FALSE, FALSE] -> [w1617 w1622 w1627 w1632 w1637 w1642 w1647 w1652 w1657 _]
                        frame 0 {
                          n892 = control-ref of="1 18"() -> (w1616:refnum<vi>)
                          n893 = property class="Clust (严格)"(reference=w1616) -> ("Controls[]"=w1618:refnum<vi>[])  [unwired: 1 in, 2 out]
                          n894 = for {
                            tunnel: w1618 -> [w1619] mode=indexing
                            tunnel: w1617 -> [w1620] mode=indexing
                            n895 = property class="Ctl"(reference=w1619, "Blinking"=w1620) -> ()  [unwired: 1 in, 2 out]
                          }
                        }
                        frame 1 {
                          n896 = control-ref of="1 19"() -> (w1621:refnum<vi>)
                          n897 = property class="Clust (严格)"(reference=w1621) -> ("Controls[]"=w1623:refnum<vi>[])  [unwired: 1 in, 2 out]
                          n898 = for {
                            tunnel: w1623 -> [w1624] mode=indexing
                            tunnel: w1622 -> [w1625] mode=indexing
                            n899 = property class="Ctl"(reference=w1624, "Blinking"=w1625) -> ()  [unwired: 1 in, 2 out]
                          }
                        }
                        frame 2 {
                          n900 = control-ref of="1 20"() -> (w1626:refnum<vi>)
                          n901 = property class="Clust (严格)"(reference=w1626) -> ("Controls[]"=w1628:refnum<vi>[])  [unwired: 1 in, 2 out]
                          n902 = for {
                            tunnel: w1628 -> [w1629] mode=indexing
                            tunnel: w1627 -> [w1630] mode=indexing
                            n903 = property class="Ctl"(reference=w1629, "Blinking"=w1630) -> ()  [unwired: 1 in, 2 out]
                          }
                        }
                        frame 3 {
                          n904 = control-ref of="1 21"() -> (w1631:refnum<vi>)
                          n905 = property class="Clust (严格)"(reference=w1631) -> ("Controls[]"=w1633:refnum<vi>[])  [unwired: 1 in, 2 out]
                          n906 = for {
                            tunnel: w1633 -> [w1634] mode=indexing
                            tunnel: w1632 -> [w1635] mode=indexing
                            n907 = property class="Ctl"(reference=w1634, "Blinking"=w1635) -> ()  [unwired: 1 in, 2 out]
                          }
                        }
                        frame 4 {
                          n908 = control-ref of="1 22"() -> (w1636:refnum<vi>)
                          n909 = property class="Clust (严格)"(reference=w1636) -> ("Controls[]"=w1638:refnum<vi>[])  [unwired: 1 in, 2 out]
                          n910 = for {
                            tunnel: w1638 -> [w1639] mode=indexing
                            tunnel: w1637 -> [w1640] mode=indexing
                            n911 = property class="Ctl"(reference=w1639, "Blinking"=w1640) -> ()  [unwired: 1 in, 2 out]
                          }
                        }
                        frame 5 {
                          n912 = control-ref of="1 23"() -> (w1641:refnum<vi>)
                          n913 = property class="Clust (严格)"(reference=w1641) -> ("Controls[]"=w1643:refnum<vi>[])  [unwired: 1 in, 2 out]
                          n914 = for {
                            tunnel: w1643 -> [w1644] mode=indexing
                            tunnel: w1642 -> [w1645] mode=indexing
                            n915 = property class="Ctl"(reference=w1644, "Blinking"=w1645) -> ()  [unwired: 1 in, 2 out]
                          }
                        }
                        frame 6 {
                          n916 = control-ref of="1 24"() -> (w1646:refnum<vi>)
                          n917 = property class="Clust (严格)"(reference=w1646) -> ("Controls[]"=w1648:refnum<vi>[])  [unwired: 1 in, 2 out]
                          n918 = for {
                            tunnel: w1648 -> [w1649] mode=indexing
                            tunnel: w1647 -> [w1650] mode=indexing
                            n919 = property class="Ctl"(reference=w1649, "Blinking"=w1650) -> ()  [unwired: 1 in, 2 out]
                          }
                        }
                        frame 7 {
                          n920 = control-ref of="1 25"() -> (w1651:refnum<vi>)
                          n921 = property class="Clust (严格)"(reference=w1651) -> ("Controls[]"=w1653:refnum<vi>[])  [unwired: 1 in, 2 out]
                          n922 = for {
                            tunnel: w1653 -> [w1654] mode=indexing
                            tunnel: w1652 -> [w1655] mode=indexing
                            n923 = property class="Ctl"(reference=w1654, "Blinking"=w1655) -> ()  [unwired: 1 in, 2 out]
                          }
                        }
                        frame 8 {
                          n924 = control-ref of="1 6"() -> (w1656:refnum<vi>)
                          n925 = property class="Clust (严格)"(reference=w1656) -> ("Controls[]"=w1658:refnum<vi>[])  [unwired: 1 in, 2 out]
                          n926 = for {
                            tunnel: w1658 -> [w1659] mode=indexing
                            tunnel: w1657 -> [w1660] mode=indexing
                            n927 = property class="Ctl"(reference=w1659, "Blinking"=w1660) -> ()  [unwired: 1 in, 2 out]
                          }
                        }
                        frame 99, Default {
                        }
                      }
                    }
                  }
                }
                n928 = local write "一次置位"(FALSE ("一次置位")) -> ()
              }
            }
          }
          frame True {
            n929 = case shown="\"单体温度\"" w1662 {
              frame "单体电压", Default {
                w1666 = 17 ("y")
                n930 = global read "单体信息全局.vi" "数据"() -> (w1679:dbl[])
                n931 = global read "单体信息全局.vi" "PF"() -> (w1665:i32)
                n932 = Array Subset(array=w1679, length=w1665) -> (w1678:dbl[])  [unwired: 1 in]
                n933 = Subtract(x="基准", y="偏差") -> (x-y=w1675:dbl)
                n934 = Quotient & Remainder(x=w1665, y=12) -> (x-y*floor(x/y)=w1671:i32, floor(x/y)=w1669:i32)
                n935 = Add(x="基准", y="偏差") -> (x+y=w1674:dbl)
                n936 = Equal To 0?(x=w1671) -> (x = 0?=w1670:bool)
                n937 = In Range and Coerce(upper limit=w1674, x=w1678, lower limit=w1675) -> (In Range?=w1673:bool[])  [unwired: 1 out]
                n938 = Increment(x=w1669) -> (x+1=w1668:i32)
                n939 = Select(t=w1669, s=w1670, f=w1668) -> (s? t:f=w1664:i32)
                n940 = Not(x=w1673) -> (.not. x?=w1663:bool[])
                n941 = Greater Or Equal?(x=w1664, y=w1666) -> (x >= y?=w1667:bool)
                n942 = case shown="真" w1667 {
                  tunnel: w1664 -> [w1769 _]
                  tunnel: w1666 -> [w1766 _]
                  tunnel: w1663 -> [w1767 _]
                  frame True {
                    n943 = Decrement(x=w1766) -> (x-1=w1765:i32)
                    n944 = Subtract(x=w1769, y=w1765) -> (x-y=w1768:i32)
                    n945 = for {
                      N: w1768 -> [_]
                      tunnel: w1767 -> [w1775]
                      tunnel: w1765 -> [w1770]
                      i -> [w1776]
                      w1773 = 12 ("y")
                      n946 = Add(x=w1770, y=w1776) -> (x+y=w1771:i32)
                      n947 = Multiply(x=w1771, y=w1773) -> (x*y=w1774:i32)
                      n948 = Array Subset(array=w1775, index=w1774, length=w1773) -> (w1772:bool[])
                      n949 = case shown="0" w1776 {
                        tunnel: w1772 -> [w1778 w1783 w1788 w1793 w1798 w1803 w1808 w1813 w1818 _]
                        frame 0 {
                          n950 = control-ref of="1 18"() -> (w1777:refnum<vi>)
                          n951 = property class="Clust (严格)"(reference=w1777) -> ("Controls[]"=w1779:refnum<vi>[])  [unwired: 1 in, 2 out]
                          n952 = for {
                            tunnel: w1779 -> [w1780] mode=indexing
                            tunnel: w1778 -> [w1781] mode=indexing
                            n953 = property class="Ctl"(reference=w1780, "Blinking"=w1781) -> ()  [unwired: 1 in, 2 out]
                          }
                        }
                        frame 1 {
                          n954 = control-ref of="1 19"() -> (w1782:refnum<vi>)
                          n955 = property class="Clust (严格)"(reference=w1782) -> ("Controls[]"=w1784:refnum<vi>[])  [unwired: 1 in, 2 out]
                          n956 = for {
                            tunnel: w1784 -> [w1785] mode=indexing
                            tunnel: w1783 -> [w1786] mode=indexing
                            n957 = property class="Ctl"(reference=w1785, "Blinking"=w1786) -> ()  [unwired: 1 in, 2 out]
                          }
                        }
                        frame 2 {
                          n958 = control-ref of="1 20"() -> (w1787:refnum<vi>)
                          n959 = property class="Clust (严格)"(reference=w1787) -> ("Controls[]"=w1789:refnum<vi>[])  [unwired: 1 in, 2 out]
                          n960 = for {
                            tunnel: w1789 -> [w1790] mode=indexing
                            tunnel: w1788 -> [w1791] mode=indexing
                            n961 = property class="Ctl"(reference=w1790, "Blinking"=w1791) -> ()  [unwired: 1 in, 2 out]
                          }
                        }
                        frame 3 {
                          n962 = control-ref of="1 21"() -> (w1792:refnum<vi>)
                          n963 = property class="Clust (严格)"(reference=w1792) -> ("Controls[]"=w1794:refnum<vi>[])  [unwired: 1 in, 2 out]
                          n964 = for {
                            tunnel: w1794 -> [w1795] mode=indexing
                            tunnel: w1793 -> [w1796] mode=indexing
                            n965 = property class="Ctl"(reference=w1795, "Blinking"=w1796) -> ()  [unwired: 1 in, 2 out]
                          }
                        }
                        frame 4 {
                          n966 = control-ref of="1 22"() -> (w1797:refnum<vi>)
                          n967 = property class="Clust (严格)"(reference=w1797) -> ("Controls[]"=w1799:refnum<vi>[])  [unwired: 1 in, 2 out]
                          n968 = for {
                            tunnel: w1799 -> [w1800] mode=indexing
                            tunnel: w1798 -> [w1801] mode=indexing
                            n969 = property class="Ctl"(reference=w1800, "Blinking"=w1801) -> ()  [unwired: 1 in, 2 out]
                          }
                        }
                        frame 5 {
                          n970 = control-ref of="1 23"() -> (w1802:refnum<vi>)
                          n971 = property class="Clust (严格)"(reference=w1802) -> ("Controls[]"=w1804:refnum<vi>[])  [unwired: 1 in, 2 out]
                          n972 = for {
                            tunnel: w1804 -> [w1805] mode=indexing
                            tunnel: w1803 -> [w1806] mode=indexing
                            n973 = property class="Ctl"(reference=w1805, "Blinking"=w1806) -> ()  [unwired: 1 in, 2 out]
                          }
                        }
                        frame 6 {
                          n974 = control-ref of="1 24"() -> (w1807:refnum<vi>)
                          n975 = property class="Clust (严格)"(reference=w1807) -> ("Controls[]"=w1809:refnum<vi>[])  [unwired: 1 in, 2 out]
                          n976 = for {
                            tunnel: w1809 -> [w1810] mode=indexing
                            tunnel: w1808 -> [w1811] mode=indexing
                            n977 = property class="Ctl"(reference=w1810, "Blinking"=w1811) -> ()  [unwired: 1 in, 2 out]
                          }
                        }
                        frame 7 {
                          n978 = control-ref of="1 25"() -> (w1812:refnum<vi>)
                          n979 = property class="Clust (严格)"(reference=w1812) -> ("Controls[]"=w1814:refnum<vi>[])  [unwired: 1 in, 2 out]
                          n980 = for {
                            tunnel: w1814 -> [w1815] mode=indexing
                            tunnel: w1813 -> [w1816] mode=indexing
                            n981 = property class="Ctl"(reference=w1815, "Blinking"=w1816) -> ()  [unwired: 1 in, 2 out]
                          }
                        }
                        frame 8 {
                          n982 = control-ref of="1 5"() -> (w1817:refnum<vi>)
                          n983 = property class="Clust (严格)"(reference=w1817) -> ("Controls[]"=w1819:refnum<vi>[])  [unwired: 1 in, 2 out]
                          n984 = for {
                            tunnel: w1819 -> [w1820] mode=indexing
                            tunnel: w1818 -> [w1821] mode=indexing
                            n985 = property class="Ctl"(reference=w1820, "Blinking"=w1821) -> ()  [unwired: 1 in, 2 out]
                          }
                        }
                        frame 99, Default {
                        }
                      }
                    }
                  }
                  frame False {
                  }
                }
                n986 = for {
                  N: w1664 -> [_]
                  tunnel: w1663 -> [w1683]
                  i -> [w1684]
                  w1681 = 12 ("y")
                  n987 = Multiply(x=w1684, y=w1681) -> (x*y=w1682:i32)
                  n988 = Array Subset(array=w1683, index=w1682, length=w1681) -> (w1680:bool[])
                  n989 = case shown="7" w1684 {
                    tunnel: w1680 -> [w1685 w1691 w1696 w1701 w1706 w1711 w1716 w1721 w1726 w1731 w1736 w1741 w1746 w1751 w1756 w1761 _]
                    frame 0 {
                      n990 = control-ref of="1 102"() -> (w1687:refnum<vi>)
                      n991 = property class="Clust (严格)"(reference=w1687) -> ("Controls[]"=w1686:refnum<vi>[])  [unwired: 1 in, 2 out]
                      n992 = for {
                        tunnel: w1686 -> [w1688] mode=indexing
                        tunnel: w1685 -> [w1689] mode=indexing
                        n993 = property class="Ctl"(reference=w1688, "Blinking"=w1689) -> ()  [unwired: 1 in, 2 out]
                      }
                    }
                    frame 1 {
                      n994 = control-ref of="1 3"() -> (w1690:refnum<vi>)
                      n995 = property class="Clust (严格)"(reference=w1690) -> ("Controls[]"=w1692:refnum<vi>[])  [unwired: 1 in, 2 out]
                      n996 = for {
                        tunnel: w1692 -> [w1693] mode=indexing
                        tunnel: w1691 -> [w1694] mode=indexing
                        n997 = property class="Ctl"(reference=w1693, "Blinking"=w1694) -> ()  [unwired: 1 in, 2 out]
                      }
                    }
                    frame 2 {
                      n998 = control-ref of="1 4"() -> (w1695:refnum<vi>)
                      n999 = property class="Clust (严格)"(reference=w1695) -> ("Controls[]"=w1697:refnum<vi>[])  [unwired: 1 in, 2 out]
                      n1000 = for {
                        tunnel: w1697 -> [w1698] mode=indexing
                        tunnel: w1696 -> [w1699] mode=indexing
                        n1001 = property class="Ctl"(reference=w1698, "Blinking"=w1699) -> ()  [unwired: 1 in, 2 out]
                      }
                    }
                    frame 3 {
                      n1002 = control-ref of="1 6"() -> (w1700:refnum<vi>)
                      n1003 = property class="Clust (严格)"(reference=w1700) -> ("Controls[]"=w1702:refnum<vi>[])  [unwired: 1 in, 2 out]
                      n1004 = for {
                        tunnel: w1702 -> [w1703] mode=indexing
                        tunnel: w1701 -> [w1704] mode=indexing
                        n1005 = property class="Ctl"(reference=w1703, "Blinking"=w1704) -> ()  [unwired: 1 in, 2 out]
                      }
                    }
                    frame 4 {
                      n1006 = control-ref of="1 7"() -> (w1705:refnum<vi>)
                      n1007 = property class="Clust (严格)"(reference=w1705) -> ("Controls[]"=w1707:refnum<vi>[])  [unwired: 1 in, 2 out]
                      n1008 = for {
                        tunnel: w1707 -> [w1708] mode=indexing
                        tunnel: w1706 -> [w1709] mode=indexing
                        n1009 = property class="Ctl"(reference=w1708, "Blinking"=w1709) -> ()  [unwired: 1 in, 2 out]
                      }
                    }
                    frame 5 {
                      n1010 = control-ref of="1 8"() -> (w1710:refnum<vi>)
                      n1011 = property class="Clust (严格)"(reference=w1710) -> ("Controls[]"=w1712:refnum<vi>[])  [unwired: 1 in, 2 out]
                      n1012 = for {
                        tunnel: w1712 -> [w1713] mode=indexing
                        tunnel: w1711 -> [w1714] mode=indexing
                        n1013 = property class="Ctl"(reference=w1713, "Blinking"=w1714) -> ()  [unwired: 1 in, 2 out]
                      }
                    }
                    frame 6 {
                      n1014 = control-ref of="1 9"() -> (w1715:refnum<vi>)
                      n1015 = property class="Clust (严格)"(reference=w1715) -> ("Controls[]"=w1717:refnum<vi>[])  [unwired: 1 in, 2 out]
                      n1016 = for {
                        tunnel: w1717 -> [w1718] mode=indexing
                        tunnel: w1716 -> [w1719] mode=indexing
                        n1017 = property class="Ctl"(reference=w1718, "Blinking"=w1719) -> ()  [unwired: 1 in, 2 out]
                      }
                    }
                    frame 7 {
                      n1018 = control-ref of="1 10"() -> (w1720:refnum<vi>)
                      n1019 = property class="Clust (严格)"(reference=w1720) -> ("Controls[]"=w1722:refnum<vi>[])  [unwired: 1 in, 2 out]
                      n1020 = for {
                        tunnel: w1722 -> [w1723] mode=indexing
                        tunnel: w1721 -> [w1724] mode=indexing
                        n1021 = property class="Ctl"(reference=w1723, "Blinking"=w1724) -> ()  [unwired: 1 in, 2 out]
                      }
                    }
                    frame 8 {
                      n1022 = control-ref of="1 26"() -> (w1725:refnum<vi>)
                      n1023 = property class="Clust (严格)"(reference=w1725) -> ("Controls[]"=w1727:refnum<vi>[])  [unwired: 1 in, 2 out]
                      n1024 = for {
                        tunnel: w1727 -> [w1728] mode=indexing
                        tunnel: w1726 -> [w1729] mode=indexing
                        n1025 = property class="Ctl"(reference=w1728, "Blinking"=w1729) -> ()  [unwired: 1 in, 2 out]
                      }
                    }
                    frame 9 {
                      n1026 = control-ref of="1 27"() -> (w1730:refnum<vi>)
                      n1027 = property class="Clust (严格)"(reference=w1730) -> ("Controls[]"=w1732:refnum<vi>[])  [unwired: 1 in, 2 out]
                      n1028 = for {
                        tunnel: w1732 -> [w1733] mode=indexing
                        tunnel: w1731 -> [w1734] mode=indexing
                        n1029 = property class="Ctl"(reference=w1733, "Blinking"=w1734) -> ()  [unwired: 1 in, 2 out]
                      }
                    }
                    frame 10 {
                      n1030 = control-ref of="1 28"() -> (w1735:refnum<vi>)
                      n1031 = property class="Clust (严格)"(reference=w1735) -> ("Controls[]"=w1737:refnum<vi>[])  [unwired: 1 in, 2 out]
                      n1032 = for {
                        tunnel: w1737 -> [w1738] mode=indexing
                        tunnel: w1736 -> [w1739] mode=indexing
                        n1033 = property class="Ctl"(reference=w1738, "Blinking"=w1739) -> ()  [unwired: 1 in, 2 out]
                      }
                    }
                    frame 11 {
                      n1034 = control-ref of="1 29"() -> (w1740:refnum<vi>)
                      n1035 = property class="Clust (严格)"(reference=w1740) -> ("Controls[]"=w1742:refnum<vi>[])  [unwired: 1 in, 2 out]
                      n1036 = for {
                        tunnel: w1742 -> [w1743] mode=indexing
                        tunnel: w1741 -> [w1744] mode=indexing
                        n1037 = property class="Ctl"(reference=w1743, "Blinking"=w1744) -> ()  [unwired: 1 in, 2 out]
                      }
                    }
                    frame 12 {
                      n1038 = control-ref of="1 30"() -> (w1745:refnum<vi>)
                      n1039 = property class="Clust (严格)"(reference=w1745) -> ("Controls[]"=w1747:refnum<vi>[])  [unwired: 1 in, 2 out]
                      n1040 = for {
                        tunnel: w1747 -> [w1748] mode=indexing
                        tunnel: w1746 -> [w1749] mode=indexing
                        n1041 = property class="Ctl"(reference=w1748, "Blinking"=w1749) -> ()  [unwired: 1 in, 2 out]
                      }
                    }
                    frame 13 {
                      n1042 = control-ref of="1 31"() -> (w1750:refnum<vi>)
                      n1043 = property class="Clust (严格)"(reference=w1750) -> ("Controls[]"=w1752:refnum<vi>[])  [unwired: 1 in, 2 out]
                      n1044 = for {
                        tunnel: w1752 -> [w1753] mode=indexing
                        tunnel: w1751 -> [w1754] mode=indexing
                        n1045 = property class="Ctl"(reference=w1753, "Blinking"=w1754) -> ()  [unwired: 1 in, 2 out]
                      }
                    }
                    frame 14 {
                      n1046 = control-ref of="1 32"() -> (w1755:refnum<vi>)
                      n1047 = property class="Clust (严格)"(reference=w1755) -> ("Controls[]"=w1757:refnum<vi>[])  [unwired: 1 in, 2 out]
                      n1048 = for {
                        tunnel: w1757 -> [w1758] mode=indexing
                        tunnel: w1756 -> [w1759] mode=indexing
                        n1049 = property class="Ctl"(reference=w1758, "Blinking"=w1759) -> ()  [unwired: 1 in, 2 out]
                      }
                    }
                    frame 15 {
                      n1050 = control-ref of="1 33"() -> (w1760:refnum<vi>)
                      n1051 = property class="Clust (严格)"(reference=w1760) -> ("Controls[]"=w1762:refnum<vi>[])  [unwired: 1 in, 2 out]
                      n1052 = for {
                        tunnel: w1762 -> [w1763] mode=indexing
                        tunnel: w1761 -> [w1764] mode=indexing
                        n1053 = property class="Ctl"(reference=w1763, "Blinking"=w1764) -> ()  [unwired: 1 in, 2 out]
                      }
                    }
                    frame 99, Default {
                    }
                  }
                }
              }
              frame "单体温度" {
                w1825 = 17 ("y")
                n1054 = global read "单体信息全局.vi" "PF2"() -> (w1824:i32)
                n1055 = global read "单体信息全局.vi" "数据 2"() -> (w1838:dbl[])
                n1056 = Array Subset(array=w1838, length=w1824) -> (w1837:dbl[])  [unwired: 1 in]
                n1057 = Subtract(x="基准", y="偏差") -> (x-y=w1834:dbl)
                n1058 = Quotient & Remainder(x=w1824, y=12) -> (x-y*floor(x/y)=w1830:i32, floor(x/y)=w1828:i32)
                n1059 = Add(x="基准", y="偏差") -> (x+y=w1833:dbl)
                n1060 = Equal To 0?(x=w1830) -> (x = 0?=w1829:bool)
                n1061 = In Range and Coerce(upper limit=w1833, x=w1837, lower limit=w1834) -> (In Range?=w1832:bool[])  [unwired: 1 out]
                n1062 = Increment(x=w1828) -> (x+1=w1827:i32)
                n1063 = Select(t=w1828, s=w1829, f=w1827) -> (s? t:f=w1823:i32)
                n1064 = Not(x=w1832) -> (.not. x?=w1822:bool[])
                n1065 = Greater Or Equal?(x=w1823, y=w1825) -> (x >= y?=w1826:bool)
                n1066 = case shown="真" w1826 {
                  tunnel: w1823 -> [w1928 _]
                  tunnel: w1825 -> [w1925 _]
                  tunnel: w1822 -> [w1926 _]
                  frame True {
                    n1067 = Decrement(x=w1925) -> (x-1=w1924:i32)
                    n1068 = Subtract(x=w1928, y=w1924) -> (x-y=w1927:i32)
                    n1069 = for {
                      N: w1927 -> [_]
                      tunnel: w1926 -> [w1934]
                      tunnel: w1924 -> [w1929]
                      i -> [w1935]
                      w1932 = 12 ("y")
                      n1070 = Add(x=w1929, y=w1935) -> (x+y=w1930:i32)
                      n1071 = Multiply(x=w1930, y=w1932) -> (x*y=w1933:i32)
                      n1072 = Array Subset(array=w1934, index=w1933, length=w1932) -> (w1931:bool[])
                      n1073 = case shown="0" w1935 {
                        tunnel: w1931 -> [w1937 w1942 w1947 w1952 w1957 w1962 w1967 w1972 w1977 _]
                        frame 0 {
                          n1074 = control-ref of="1 18"() -> (w1936:refnum<vi>)
                          n1075 = property class="Clust (严格)"(reference=w1936) -> ("Controls[]"=w1938:refnum<vi>[])  [unwired: 1 in, 2 out]
                          n1076 = for {
                            tunnel: w1938 -> [w1939] mode=indexing
                            tunnel: w1937 -> [w1940] mode=indexing
                            n1077 = property class="Ctl"(reference=w1939, "Blinking"=w1940) -> ()  [unwired: 1 in, 2 out]
                          }
                        }
                        frame 1 {
                          n1078 = control-ref of="1 19"() -> (w1941:refnum<vi>)
                          n1079 = property class="Clust (严格)"(reference=w1941) -> ("Controls[]"=w1943:refnum<vi>[])  [unwired: 1 in, 2 out]
                          n1080 = for {
                            tunnel: w1943 -> [w1944] mode=indexing
                            tunnel: w1942 -> [w1945] mode=indexing
                            n1081 = property class="Ctl"(reference=w1944, "Blinking"=w1945) -> ()  [unwired: 1 in, 2 out]
                          }
                        }
                        frame 2 {
                          n1082 = control-ref of="1 20"() -> (w1946:refnum<vi>)
                          n1083 = property class="Clust (严格)"(reference=w1946) -> ("Controls[]"=w1948:refnum<vi>[])  [unwired: 1 in, 2 out]
                          n1084 = for {
                            tunnel: w1948 -> [w1949] mode=indexing
                            tunnel: w1947 -> [w1950] mode=indexing
                            n1085 = property class="Ctl"(reference=w1949, "Blinking"=w1950) -> ()  [unwired: 1 in, 2 out]
                          }
                        }
                        frame 3 {
                          n1086 = control-ref of="1 21"() -> (w1951:refnum<vi>)
                          n1087 = property class="Clust (严格)"(reference=w1951) -> ("Controls[]"=w1953:refnum<vi>[])  [unwired: 1 in, 2 out]
                          n1088 = for {
                            tunnel: w1953 -> [w1954] mode=indexing
                            tunnel: w1952 -> [w1955] mode=indexing
                            n1089 = property class="Ctl"(reference=w1954, "Blinking"=w1955) -> ()  [unwired: 1 in, 2 out]
                          }
                        }
                        frame 4 {
                          n1090 = control-ref of="1 22"() -> (w1956:refnum<vi>)
                          n1091 = property class="Clust (严格)"(reference=w1956) -> ("Controls[]"=w1958:refnum<vi>[])  [unwired: 1 in, 2 out]
                          n1092 = for {
                            tunnel: w1958 -> [w1959] mode=indexing
                            tunnel: w1957 -> [w1960] mode=indexing
                            n1093 = property class="Ctl"(reference=w1959, "Blinking"=w1960) -> ()  [unwired: 1 in, 2 out]
                          }
                        }
                        frame 5 {
                          n1094 = control-ref of="1 23"() -> (w1961:refnum<vi>)
                          n1095 = property class="Clust (严格)"(reference=w1961) -> ("Controls[]"=w1963:refnum<vi>[])  [unwired: 1 in, 2 out]
                          n1096 = for {
                            tunnel: w1963 -> [w1964] mode=indexing
                            tunnel: w1962 -> [w1965] mode=indexing
                            n1097 = property class="Ctl"(reference=w1964, "Blinking"=w1965) -> ()  [unwired: 1 in, 2 out]
                          }
                        }
                        frame 6 {
                          n1098 = control-ref of="1 24"() -> (w1966:refnum<vi>)
                          n1099 = property class="Clust (严格)"(reference=w1966) -> ("Controls[]"=w1968:refnum<vi>[])  [unwired: 1 in, 2 out]
                          n1100 = for {
                            tunnel: w1968 -> [w1969] mode=indexing
                            tunnel: w1967 -> [w1970] mode=indexing
                            n1101 = property class="Ctl"(reference=w1969, "Blinking"=w1970) -> ()  [unwired: 1 in, 2 out]
                          }
                        }
                        frame 7 {
                          n1102 = control-ref of="1 25"() -> (w1971:refnum<vi>)
                          n1103 = property class="Clust (严格)"(reference=w1971) -> ("Controls[]"=w1973:refnum<vi>[])  [unwired: 1 in, 2 out]
                          n1104 = for {
                            tunnel: w1973 -> [w1974] mode=indexing
                            tunnel: w1972 -> [w1975] mode=indexing
                            n1105 = property class="Ctl"(reference=w1974, "Blinking"=w1975) -> ()  [unwired: 1 in, 2 out]
                          }
                        }
                        frame 8 {
                          n1106 = control-ref of="1 6"() -> (w1976:refnum<vi>)
                          n1107 = property class="Clust (严格)"(reference=w1976) -> ("Controls[]"=w1978:refnum<vi>[])  [unwired: 1 in, 2 out]
                          n1108 = for {
                            tunnel: w1978 -> [w1979] mode=indexing
                            tunnel: w1977 -> [w1980] mode=indexing
                            n1109 = property class="Ctl"(reference=w1979, "Blinking"=w1980) -> ()  [unwired: 1 in, 2 out]
                          }
                        }
                        frame 99, Default {
                        }
                      }
                    }
                  }
                  frame False {
                  }
                }
                n1110 = for {
                  N: w1823 -> [_]
                  tunnel: w1822 -> [w1842]
                  i -> [w1843]
                  w1840 = 12 ("y")
                  n1111 = Multiply(x=w1843, y=w1840) -> (x*y=w1841:i32)
                  n1112 = Array Subset(array=w1842, index=w1841, length=w1840) -> (w1839:bool[])
                  n1113 = case shown="15" w1843 {
                    tunnel: w1839 -> [w1845 w1850 w1855 w1860 w1865 w1870 w1875 w1880 w1885 w1890 w1895 w1900 w1905 w1910 w1915 w1920 _]
                    frame 0 {
                      n1114 = control-ref of="1 102"() -> (w1844:refnum<vi>)
                      n1115 = property class="Clust (严格)"(reference=w1844) -> ("Controls[]"=w1846:refnum<vi>[])  [unwired: 1 in, 2 out]
                      n1116 = for {
                        tunnel: w1846 -> [w1847] mode=indexing
                        tunnel: w1845 -> [w1848] mode=indexing
                        n1117 = property class="Ctl"(reference=w1847, "Blinking"=w1848) -> ()  [unwired: 1 in, 2 out]
                      }
                    }
                    frame 1 {
                      n1118 = control-ref of="1 3"() -> (w1849:refnum<vi>)
                      n1119 = property class="Clust (严格)"(reference=w1849) -> ("Controls[]"=w1851:refnum<vi>[])  [unwired: 1 in, 2 out]
                      n1120 = for {
                        tunnel: w1851 -> [w1852] mode=indexing
                        tunnel: w1850 -> [w1853] mode=indexing
                        n1121 = property class="Ctl"(reference=w1852, "Blinking"=w1853) -> ()  [unwired: 1 in, 2 out]
                      }
                    }
                    frame 2 {
                      n1122 = control-ref of="1 4"() -> (w1854:refnum<vi>)
                      n1123 = property class="Clust (严格)"(reference=w1854) -> ("Controls[]"=w1856:refnum<vi>[])  [unwired: 1 in, 2 out]
                      n1124 = for {
                        tunnel: w1856 -> [w1857] mode=indexing
                        tunnel: w1855 -> [w1858] mode=indexing
                        n1125 = property class="Ctl"(reference=w1857, "Blinking"=w1858) -> ()  [unwired: 1 in, 2 out]
                      }
                    }
                    frame 3 {
                      n1126 = control-ref of="1 6"() -> (w1859:refnum<vi>)
                      n1127 = property class="Clust (严格)"(reference=w1859) -> ("Controls[]"=w1861:refnum<vi>[])  [unwired: 1 in, 2 out]
                      n1128 = for {
                        tunnel: w1861 -> [w1862] mode=indexing
                        tunnel: w1860 -> [w1863] mode=indexing
                        n1129 = property class="Ctl"(reference=w1862, "Blinking"=w1863) -> ()  [unwired: 1 in, 2 out]
                      }
                    }
                    frame 4 {
                      n1130 = control-ref of="1 7"() -> (w1864:refnum<vi>)
                      n1131 = property class="Clust (严格)"(reference=w1864) -> ("Controls[]"=w1866:refnum<vi>[])  [unwired: 1 in, 2 out]
                      n1132 = for {
                        tunnel: w1866 -> [w1867] mode=indexing
                        tunnel: w1865 -> [w1868] mode=indexing
                        n1133 = property class="Ctl"(reference=w1867, "Blinking"=w1868) -> ()  [unwired: 1 in, 2 out]
                      }
                    }
                    frame 5 {
                      n1134 = control-ref of="1 8"() -> (w1869:refnum<vi>)
                      n1135 = property class="Clust (严格)"(reference=w1869) -> ("Controls[]"=w1871:refnum<vi>[])  [unwired: 1 in, 2 out]
                      n1136 = for {
                        tunnel: w1871 -> [w1872] mode=indexing
                        tunnel: w1870 -> [w1873] mode=indexing
                        n1137 = property class="Ctl"(reference=w1872, "Blinking"=w1873) -> ()  [unwired: 1 in, 2 out]
                      }
                    }
                    frame 6 {
                      n1138 = control-ref of="1 9"() -> (w1874:refnum<vi>)
                      n1139 = property class="Clust (严格)"(reference=w1874) -> ("Controls[]"=w1876:refnum<vi>[])  [unwired: 1 in, 2 out]
                      n1140 = for {
                        tunnel: w1876 -> [w1877] mode=indexing
                        tunnel: w1875 -> [w1878] mode=indexing
                        n1141 = property class="Ctl"(reference=w1877, "Blinking"=w1878) -> ()  [unwired: 1 in, 2 out]
                      }
                    }
                    frame 7 {
                      n1142 = control-ref of="1 10"() -> (w1879:refnum<vi>)
                      n1143 = property class="Clust (严格)"(reference=w1879) -> ("Controls[]"=w1881:refnum<vi>[])  [unwired: 1 in, 2 out]
                      n1144 = for {
                        tunnel: w1881 -> [w1882] mode=indexing
                        tunnel: w1880 -> [w1883] mode=indexing
                        n1145 = property class="Ctl"(reference=w1882, "Blinking"=w1883) -> ()  [unwired: 1 in, 2 out]
                      }
                    }
                    frame 8 {
                      n1146 = control-ref of="1 26"() -> (w1884:refnum<vi>)
                      n1147 = property class="Clust (严格)"(reference=w1884) -> ("Controls[]"=w1886:refnum<vi>[])  [unwired: 1 in, 2 out]
                      n1148 = for {
                        tunnel: w1886 -> [w1887] mode=indexing
                        tunnel: w1885 -> [w1888] mode=indexing
                        n1149 = property class="Ctl"(reference=w1887, "Blinking"=w1888) -> ()  [unwired: 1 in, 2 out]
                      }
                    }
                    frame 9 {
                      n1150 = control-ref of="1 27"() -> (w1889:refnum<vi>)
                      n1151 = property class="Clust (严格)"(reference=w1889) -> ("Controls[]"=w1891:refnum<vi>[])  [unwired: 1 in, 2 out]
                      n1152 = for {
                        tunnel: w1891 -> [w1892] mode=indexing
                        tunnel: w1890 -> [w1893] mode=indexing
                        n1153 = property class="Ctl"(reference=w1892, "Blinking"=w1893) -> ()  [unwired: 1 in, 2 out]
                      }
                    }
                    frame 10 {
                      n1154 = control-ref of="1 28"() -> (w1894:refnum<vi>)
                      n1155 = property class="Clust (严格)"(reference=w1894) -> ("Controls[]"=w1896:refnum<vi>[])  [unwired: 1 in, 2 out]
                      n1156 = for {
                        tunnel: w1896 -> [w1897] mode=indexing
                        tunnel: w1895 -> [w1898] mode=indexing
                        n1157 = property class="Ctl"(reference=w1897, "Blinking"=w1898) -> ()  [unwired: 1 in, 2 out]
                      }
                    }
                    frame 11 {
                      n1158 = control-ref of="1 29"() -> (w1899:refnum<vi>)
                      n1159 = property class="Clust (严格)"(reference=w1899) -> ("Controls[]"=w1901:refnum<vi>[])  [unwired: 1 in, 2 out]
                      n1160 = for {
                        tunnel: w1901 -> [w1902] mode=indexing
                        tunnel: w1900 -> [w1903] mode=indexing
                        n1161 = property class="Ctl"(reference=w1902, "Blinking"=w1903) -> ()  [unwired: 1 in, 2 out]
                      }
                    }
                    frame 12 {
                      n1162 = control-ref of="1 30"() -> (w1904:refnum<vi>)
                      n1163 = property class="Clust (严格)"(reference=w1904) -> ("Controls[]"=w1906:refnum<vi>[])  [unwired: 1 in, 2 out]
                      n1164 = for {
                        tunnel: w1906 -> [w1907] mode=indexing
                        tunnel: w1905 -> [w1908] mode=indexing
                        n1165 = property class="Ctl"(reference=w1907, "Blinking"=w1908) -> ()  [unwired: 1 in, 2 out]
                      }
                    }
                    frame 13 {
                      n1166 = control-ref of="1 31"() -> (w1909:refnum<vi>)
                      n1167 = property class="Clust (严格)"(reference=w1909) -> ("Controls[]"=w1911:refnum<vi>[])  [unwired: 1 in, 2 out]
                      n1168 = for {
                        tunnel: w1911 -> [w1912] mode=indexing
                        tunnel: w1910 -> [w1913] mode=indexing
                        n1169 = property class="Ctl"(reference=w1912, "Blinking"=w1913) -> ()  [unwired: 1 in, 2 out]
                      }
                    }
                    frame 14 {
                      n1170 = control-ref of="1 32"() -> (w1914:refnum<vi>)
                      n1171 = property class="Clust (严格)"(reference=w1914) -> ("Controls[]"=w1916:refnum<vi>[])  [unwired: 1 in, 2 out]
                      n1172 = for {
                        tunnel: w1916 -> [w1917] mode=indexing
                        tunnel: w1915 -> [w1918] mode=indexing
                        n1173 = property class="Ctl"(reference=w1917, "Blinking"=w1918) -> ()  [unwired: 1 in, 2 out]
                      }
                    }
                    frame 15 {
                      n1174 = control-ref of="1 33"() -> (w1919:refnum<vi>)
                      n1175 = property class="Clust (严格)"(reference=w1919) -> ("Controls[]"=w1921:refnum<vi>[])  [unwired: 1 in, 2 out]
                      n1176 = for {
                        tunnel: w1921 -> [w1922] mode=indexing
                        tunnel: w1920 -> [w1923] mode=indexing
                        n1177 = property class="Ctl"(reference=w1922, "Blinking"=w1923) -> ()  [unwired: 1 in, 2 out]
                      }
                    }
                    frame 99, Default {
                    }
                  }
                }
              }
            }
            n1178 = local write "一次置位"(TRUE ("一次置位")) -> ()
          }
        }
      }
    }
    frame Disabled {
    }
  }
  n1179 = local write "213"(TRUE ("213")) -> ()
  n1180 = disable-structure shown="禁用" {
    frame Disabled {
      n1181 = control-ref of="选项卡控件"() -> (w1981:refnum<vi>)
      n1182 = control-ref of="均衡信息"() -> (w1982:refnum<vi>)
      n1183 = call "单数据解析_new.vi"(8:w1981) -> ("PF"=w1984:i32, "均衡标记"=w1983:i32[][])  [unwired: 1 in, 8 out]
      n1184 = call "均衡解析.vi"("位置"=w1984, "均衡标记"=w1983, "均衡引用"=w1982) -> ()  [unwired: 9 out]
    }
    frame Enabled {
    }
  }
  n1185 = local write "一次置位"(TRUE ("一次置位")) -> ()
  n1186 = for {
    N: 16 -> [_]
    i -> [w1986]
    n1187 = case shown="8" w1986 {
      tunnel: bool[] [FALSE, FALSE, FALSE, FALSE, FALSE, FALSE, FALSE, FALSE, FALSE, FALSE, FALSE, FALSE, FALSE] -> [w1988 w1993 w1998 w2003 w2008 w2013 w2018 w2023 w2028 w2033 w2038 w2043 w2048 w2053 w2058 w2063 _]
      frame 0 {
        n1188 = control-ref of="1 102"() -> (w1987:refnum<vi>)
        n1189 = property class="Clust (严格)"(reference=w1987) -> ("Controls[]"=w1989:refnum<vi>[])  [unwired: 1 in, 2 out]
        n1190 = for {
          tunnel: w1989 -> [w1990] mode=indexing
          tunnel: w1988 -> [w1991] mode=indexing
          n1191 = property class="Ctl"(reference=w1990, "Blinking"=w1991) -> ()  [unwired: 1 in, 2 out]
        }
      }
      frame 1 {
        n1192 = control-ref of="1 3"() -> (w1992:refnum<vi>)
        n1193 = property class="Clust (严格)"(reference=w1992) -> ("Controls[]"=w1994:refnum<vi>[])  [unwired: 1 in, 2 out]
        n1194 = for {
          tunnel: w1994 -> [w1995] mode=indexing
          tunnel: w1993 -> [w1996] mode=indexing
          n1195 = property class="Ctl"(reference=w1995, "Blinking"=w1996) -> ()  [unwired: 1 in, 2 out]
        }
      }
      frame 2 {
        n1196 = control-ref of="1 4"() -> (w1997:refnum<vi>)
        n1197 = property class="Clust (严格)"(reference=w1997) -> ("Controls[]"=w1999:refnum<vi>[])  [unwired: 1 in, 2 out]
        n1198 = for {
          tunnel: w1999 -> [w2000] mode=indexing
          tunnel: w1998 -> [w2001] mode=indexing
          n1199 = property class="Ctl"(reference=w2000, "Blinking"=w2001) -> ()  [unwired: 1 in, 2 out]
        }
      }
      frame 3 {
        n1200 = control-ref of="1 6"() -> (w2002:refnum<vi>)
        n1201 = property class="Clust (严格)"(reference=w2002) -> ("Controls[]"=w2004:refnum<vi>[])  [unwired: 1 in, 2 out]
        n1202 = for {
          tunnel: w2004 -> [w2005] mode=indexing
          tunnel: w2003 -> [w2006] mode=indexing
          n1203 = property class="Ctl"(reference=w2005, "Blinking"=w2006) -> ()  [unwired: 1 in, 2 out]
        }
      }
      frame 4 {
        n1204 = control-ref of="1 7"() -> (w2007:refnum<vi>)
        n1205 = property class="Clust (严格)"(reference=w2007) -> ("Controls[]"=w2009:refnum<vi>[])  [unwired: 1 in, 2 out]
        n1206 = for {
          tunnel: w2009 -> [w2010] mode=indexing
          tunnel: w2008 -> [w2011] mode=indexing
          n1207 = property class="Ctl"(reference=w2010, "Blinking"=w2011) -> ()  [unwired: 1 in, 2 out]
        }
      }
      frame 5 {
        n1208 = control-ref of="1 8"() -> (w2012:refnum<vi>)
        n1209 = property class="Clust (严格)"(reference=w2012) -> ("Controls[]"=w2014:refnum<vi>[])  [unwired: 1 in, 2 out]
        n1210 = for {
          tunnel: w2014 -> [w2015] mode=indexing
          tunnel: w2013 -> [w2016] mode=indexing
          n1211 = property class="Ctl"(reference=w2015, "Blinking"=w2016) -> ()  [unwired: 1 in, 2 out]
        }
      }
      frame 6 {
        n1212 = control-ref of="1 9"() -> (w2017:refnum<vi>)
        n1213 = property class="Clust (严格)"(reference=w2017) -> ("Controls[]"=w2019:refnum<vi>[])  [unwired: 1 in, 2 out]
        n1214 = for {
          tunnel: w2019 -> [w2020] mode=indexing
          tunnel: w2018 -> [w2021] mode=indexing
          n1215 = property class="Ctl"(reference=w2020, "Blinking"=w2021) -> ()  [unwired: 1 in, 2 out]
        }
      }
      frame 7 {
        n1216 = control-ref of="1 10"() -> (w2022:refnum<vi>)
        n1217 = property class="Clust (严格)"(reference=w2022) -> ("Controls[]"=w2024:refnum<vi>[])  [unwired: 1 in, 2 out]
        n1218 = for {
          tunnel: w2024 -> [w2025] mode=indexing
          tunnel: w2023 -> [w2026] mode=indexing
          n1219 = property class="Ctl"(reference=w2025, "Blinking"=w2026) -> ()  [unwired: 1 in, 2 out]
        }
      }
      frame 8 {
        n1220 = control-ref of="1 26"() -> (w2027:refnum<vi>)
        n1221 = property class="Clust (严格)"(reference=w2027) -> ("Controls[]"=w2029:refnum<vi>[])  [unwired: 1 in, 2 out]
        n1222 = for {
          tunnel: w2029 -> [w2030] mode=indexing
          tunnel: w2028 -> [w2031] mode=indexing
          n1223 = property class="Ctl"(reference=w2030, "Blinking"=w2031) -> ()  [unwired: 1 in, 2 out]
        }
      }
      frame 9 {
        n1224 = control-ref of="1 27"() -> (w2032:refnum<vi>)
        n1225 = property class="Clust (严格)"(reference=w2032) -> ("Controls[]"=w2034:refnum<vi>[])  [unwired: 1 in, 2 out]
        n1226 = for {
          tunnel: w2034 -> [w2035] mode=indexing
          tunnel: w2033 -> [w2036] mode=indexing
          n1227 = property class="Ctl"(reference=w2035, "Blinking"=w2036) -> ()  [unwired: 1 in, 2 out]
        }
      }
      frame 10 {
        n1228 = control-ref of="1 28"() -> (w2037:refnum<vi>)
        n1229 = property class="Clust (严格)"(reference=w2037) -> ("Controls[]"=w2039:refnum<vi>[])  [unwired: 1 in, 2 out]
        n1230 = for {
          tunnel: w2039 -> [w2040] mode=indexing
          tunnel: w2038 -> [w2041] mode=indexing
          n1231 = property class="Ctl"(reference=w2040, "Blinking"=w2041) -> ()  [unwired: 1 in, 2 out]
        }
      }
      frame 11 {
        n1232 = control-ref of="1 29"() -> (w2042:refnum<vi>)
        n1233 = property class="Clust (严格)"(reference=w2042) -> ("Controls[]"=w2044:refnum<vi>[])  [unwired: 1 in, 2 out]
        n1234 = for {
          tunnel: w2044 -> [w2045] mode=indexing
          tunnel: w2043 -> [w2046] mode=indexing
          n1235 = property class="Ctl"(reference=w2045, "Blinking"=w2046) -> ()  [unwired: 1 in, 2 out]
        }
      }
      frame 12 {
        n1236 = control-ref of="1 30"() -> (w2047:refnum<vi>)
        n1237 = property class="Clust (严格)"(reference=w2047) -> ("Controls[]"=w2049:refnum<vi>[])  [unwired: 1 in, 2 out]
        n1238 = for {
          tunnel: w2049 -> [w2050] mode=indexing
          tunnel: w2048 -> [w2051] mode=indexing
          n1239 = property class="Ctl"(reference=w2050, "Blinking"=w2051) -> ()  [unwired: 1 in, 2 out]
        }
      }
      frame 13 {
        n1240 = control-ref of="1 31"() -> (w2052:refnum<vi>)
        n1241 = property class="Clust (严格)"(reference=w2052) -> ("Controls[]"=w2054:refnum<vi>[])  [unwired: 1 in, 2 out]
        n1242 = for {
          tunnel: w2054 -> [w2055] mode=indexing
          tunnel: w2053 -> [w2056] mode=indexing
          n1243 = property class="Ctl"(reference=w2055, "Blinking"=w2056) -> ()  [unwired: 1 in, 2 out]
        }
      }
      frame 14 {
        n1244 = control-ref of="1 32"() -> (w2057:refnum<vi>)
        n1245 = property class="Clust (严格)"(reference=w2057) -> ("Controls[]"=w2059:refnum<vi>[])  [unwired: 1 in, 2 out]
        n1246 = for {
          tunnel: w2059 -> [w2060] mode=indexing
          tunnel: w2058 -> [w2061] mode=indexing
          n1247 = property class="Ctl"(reference=w2060, "Blinking"=w2061) -> ()  [unwired: 1 in, 2 out]
        }
      }
      frame 15 {
        n1248 = control-ref of="1 33"() -> (w2062:refnum<vi>)
        n1249 = property class="Clust (严格)"(reference=w2062) -> ("Controls[]"=w2064:refnum<vi>[])  [unwired: 1 in, 2 out]
        n1250 = for {
          tunnel: w2064 -> [w2065] mode=indexing
          tunnel: w2063 -> [w2066] mode=indexing
          n1251 = property class="Ctl"(reference=w2065, "Blinking"=w2066) -> ()  [unwired: 1 in, 2 out]
        }
      }
      frame 99, Default {
      }
    }
  }
  n1252 = for {
    N: 9 -> [_]
    i -> [w2068]
    n1253 = case shown="7" w2068 {
      tunnel: bool[] [FALSE, FALSE, FALSE, FALSE, FALSE, FALSE, FALSE, FALSE, FALSE, FALSE, FALSE, FALSE, FALSE] -> [w2070 w2075 w2080 w2085 w2090 w2095 w2100 w2105 w2110 _]
      frame 0 {
        n1254 = control-ref of="1 18"() -> (w2069:refnum<vi>)
        n1255 = property class="Clust (严格)"(reference=w2069) -> ("Controls[]"=w2071:refnum<vi>[])  [unwired: 1 in, 2 out]
        n1256 = for {
          tunnel: w2071 -> [w2072] mode=indexing
          tunnel: w2070 -> [w2073] mode=indexing
          n1257 = property class="Ctl"(reference=w2072, "Blinking"=w2073) -> ()  [unwired: 1 in, 2 out]
        }
      }
      frame 1 {
        n1258 = control-ref of="1 19"() -> (w2074:refnum<vi>)
        n1259 = property class="Clust (严格)"(reference=w2074) -> ("Controls[]"=w2076:refnum<vi>[])  [unwired: 1 in, 2 out]
        n1260 = for {
          tunnel: w2076 -> [w2077] mode=indexing
          tunnel: w2075 -> [w2078] mode=indexing
          n1261 = property class="Ctl"(reference=w2077, "Blinking"=w2078) -> ()  [unwired: 1 in, 2 out]
        }
      }
      frame 2 {
        n1262 = control-ref of="1 20"() -> (w2079:refnum<vi>)
        n1263 = property class="Clust (严格)"(reference=w2079) -> ("Controls[]"=w2081:refnum<vi>[])  [unwired: 1 in, 2 out]
        n1264 = for {
          tunnel: w2081 -> [w2082] mode=indexing
          tunnel: w2080 -> [w2083] mode=indexing
          n1265 = property class="Ctl"(reference=w2082, "Blinking"=w2083) -> ()  [unwired: 1 in, 2 out]
        }
      }
      frame 3 {
        n1266 = control-ref of="1 21"() -> (w2084:refnum<vi>)
        n1267 = property class="Clust (严格)"(reference=w2084) -> ("Controls[]"=w2086:refnum<vi>[])  [unwired: 1 in, 2 out]
        n1268 = for {
          tunnel: w2086 -> [w2087] mode=indexing
          tunnel: w2085 -> [w2088] mode=indexing
          n1269 = property class="Ctl"(reference=w2087, "Blinking"=w2088) -> ()  [unwired: 1 in, 2 out]
        }
      }
      frame 4 {
        n1270 = control-ref of="1 22"() -> (w2089:refnum<vi>)
        n1271 = property class="Clust (严格)"(reference=w2089) -> ("Controls[]"=w2091:refnum<vi>[])  [unwired: 1 in, 2 out]
        n1272 = for {
          tunnel: w2091 -> [w2092] mode=indexing
          tunnel: w2090 -> [w2093] mode=indexing
          n1273 = property class="Ctl"(reference=w2092, "Blinking"=w2093) -> ()  [unwired: 1 in, 2 out]
        }
      }
      frame 5 {
        n1274 = control-ref of="1 23"() -> (w2094:refnum<vi>)
        n1275 = property class="Clust (严格)"(reference=w2094) -> ("Controls[]"=w2096:refnum<vi>[])  [unwired: 1 in, 2 out]
        n1276 = for {
          tunnel: w2096 -> [w2097] mode=indexing
          tunnel: w2095 -> [w2098] mode=indexing
          n1277 = property class="Ctl"(reference=w2097, "Blinking"=w2098) -> ()  [unwired: 1 in, 2 out]
        }
      }
      frame 6 {
        n1278 = control-ref of="1 24"() -> (w2099:refnum<vi>)
        n1279 = property class="Clust (严格)"(reference=w2099) -> ("Controls[]"=w2101:refnum<vi>[])  [unwired: 1 in, 2 out]
        n1280 = for {
          tunnel: w2101 -> [w2102] mode=indexing
          tunnel: w2100 -> [w2103] mode=indexing
          n1281 = property class="Ctl"(reference=w2102, "Blinking"=w2103) -> ()  [unwired: 1 in, 2 out]
        }
      }
      frame 7 {
        n1282 = control-ref of="1 25"() -> (w2104:refnum<vi>)
        n1283 = property class="Clust (严格)"(reference=w2104) -> ("Controls[]"=w2106:refnum<vi>[])  [unwired: 1 in, 2 out]
        n1284 = for {
          tunnel: w2106 -> [w2107] mode=indexing
          tunnel: w2105 -> [w2108] mode=indexing
          n1285 = property class="Ctl"(reference=w2107, "Blinking"=w2108) -> ()  [unwired: 1 in, 2 out]
        }
      }
      frame 8 {
        n1286 = control-ref of="1 6"() -> (w2109:refnum<vi>)
        n1287 = property class="Clust (严格)"(reference=w2109) -> ("Controls[]"=w2111:refnum<vi>[])  [unwired: 1 in, 2 out]
        n1288 = for {
          tunnel: w2111 -> [w2112] mode=indexing
          tunnel: w2110 -> [w2113] mode=indexing
          n1289 = property class="Ctl"(reference=w2112, "Blinking"=w2113) -> ()  [unwired: 1 in, 2 out]
        }
      }
      frame 99, Default {
      }
    }
  }
  n1290 = local write "充电均衡"(T9 {"充电1"=13816530, "充电1"=13816530, "充电1"=13816530, "充电1"=13816530, "充电1"=13816530, "充电1"=13816530, "充电1"=13816530, "充电1"=13816530, "充电1"=13816530, "充电1"=13816530, "充电1"=13816530, "充电1"=13816530} ("充电均衡")) -> ()
  n1291 = disable-structure shown="禁用" {
    frame Disabled {
      n1292 = Not A Number/Path/Refnum?(number/path/refnum="数据") -> (NaN/Path/Refnum?=w2118:bool)
      n1293 = Not A Number/Path/Refnum?(number/path/refnum="数据位置") -> (NaN/Path/Refnum?=w2117:bool)
      n1294 = Or(x=w2118, y=w2117) -> (x .or. y?=w2116:bool)
      n1295 = case shown="假" w2116 {
        tunnel: "数据位置" -> [w2122 _]
        tunnel: "数据" -> [w2120 _]
        frame False {
          n1296 = property class="Arr (严格)"(reference=w2122) -> ("Value"=w2121:dbl[])  [unwired: 1 in, 2 out]
          n1297 = property class="Arr (严格)"(reference=w2120) -> ("Value"=w2119:dbl[])  [unwired: 1 in, 2 out]
          n1298 = call "数组去零.vi"("输入"=w2121) -> ("输出"=w2123:dbl[])
          n1299 = Array Size(array=w2123) -> (size(s)=w2124:i32)
          n1300 = Quotient & Remainder(x=w2124, y=24) -> (x-y*floor(x/y)=w2130:i32, floor(x/y)=w2127:i32)
          n1301 = Equal To 0?(x=w2130) -> (x = 0?=w2129:bool)
          n1302 = Increment(x=w2127) -> (x+1=w2126:i32)
          n1303 = Select(t=w2127, s=w2129, f=w2126) -> (s? t:f=w2128:i32)
          n1304 = Array Subset(array=w2119, length=w2124) -> (w2132:dbl[])  [unwired: 1 in]
          n1305 = for {
            N: w2128 -> [_]
            tunnel: w2132 -> [w2145]
            tunnel: [w2136] -> w2125
            tunnel: w2123 -> [w2139]
            i -> [w2142]
            w2137 = 24 ("y")
            n1306 = Multiply(x=w2142, y=w2137) -> (x*y=w2138:i32)
            n1307 = Increment(x=w2142) -> (x+1=w2140:i32)
            n1308 = Array Subset(array=w2145, index=w2138, length=w2137) -> (w2141:dbl[])
            n1309 = Array Subset(array=w2139, index=w2138, length=w2137) -> (w2135:dbl[])
            n1310 = Multiply(x=w2140, y=3) -> (x*y=w2143:i32)
            n1311 = Decrement(x=w2143) -> (x-1=w2134:i32)
            n1312 = Decrement(x=w2134) -> (x-1=w2133:i32)
            n1313 = call "表格数据输入(数值)-8.6.vi"("列数"=w2133, "数值数组"=w2135, "表格引用"=w2136) -> ()  [unwired: 9 out]
            n1314 = call "表格数据输入(数值)-8.6.vi"("列数"=w2134, "数值数组"=w2141, "表格引用"=w2136) -> ()  [unwired: 9 out]
          }
        }
        frame True {
        }
      }
    }
    frame Enabled {
    }
  }
  n1315 = disable-structure shown="禁用" {
    frame Disabled {
      n1316 = Multiply(x=12, y=24) -> (x*y=w2152:i32)
      n1317 = for {
        N: 12 -> [_]
        tunnel: [w2157] -> w2154 mode=indexing
        tunnel: [w2156] -> _
        tunnel: w2152 -> [w2156]
        i -> [w2163]
        n1318 = Increment(x=w2163) -> (x+1=w2162:i32)
        n1319 = Add(x=w2156, y=w2162) -> (x+y=w2158:i32)
        n1320 = Number To Decimal String(number=w2158) -> (decimal integer string=w2161:string)  [unwired: 1 out]
        n1321 = Concatenate Strings("第" ("字符串"), w2161, "串" ("字符串")) -> (w2157:string)
      }
      n1322 = Multiply(x=12, y=3) -> (x*y=w2149:i32)
      n1323 = call "表格数据输入-8.6.vi"("行数"=u32 0, "列数"=w2149, "字符串数组"=w2154) -> ("表格引用"=w2155:refnum<vi>)  [unwired: 8 out]
    }
    frame Enabled {
    }
  }
  n1324 = local write "停止"(FALSE ("停止")) -> ()
  "单选选项2" <- FALSE ("单选选项2")
